vi "Multichannel Lockin.vi"() -> ()   [LabVIEW 2019, in "Instrument.Lockin.lvclass"]
uses:
  Instrument.Lockin/Instrument.Lockin.lvclass
  <vilib>/Utility/error.llb/DialogType.ctl
  <vilib>/measure/NI_MAPro.lvlib
  <vilib>/Waveform/WDTOps.llb/WDT Waveform to XY Pairs DBL.vi
  <vilib>/Utility/config.llb/NI_LVConfig.lvlib
  <vilib>/JKI/JKI SMO/SMO/SMO.lvclass
  Lockin.DAQ/Lockin.DAQ.lvclass
  <userlib>/LevyLab/Levylab Instruments/SMOs/RemoteControl/RemoteControl.lvclass
  <userlib>/LevyLab/Levylab Instruments/SMOs/RemoteControl/Typedefs/Message--Cluster.ctl
  <userlib>/LevyLab/Levylab Instruments/SMOs/RemoteControl/Typedefs/PrivateEvents--RemoteControl.Configure.ctl
  Lockin.DAQ/Typedefs/Results--Cluster.ctl
  <userlib>/LevyLab/Levylab Instruments/SMOs/Instrument/Instrument.lvclass
  Lockin.DAQ/Typedefs/Set State-enum.ctl
  <vilib>/JKI/JKI SMO/SMO/Typedefs/Reserve State--Enum.ctl
  <vilib>/JKI/JKI SMO/SMO/Typedefs/Public Events.ctl
  <vilib>/JKI/JKI SMO/SMO/Typedefs/SMOState --Enum.ctl
  Lockin.DAQ/Typedefs/Sample Mode--Ring.ctl
  Lockin.DAQ/Typedefs/Sweep Configuration--Cluster.ctl
  Lockin.DAQ/Typedefs/SweepResults--Cluster.ctl
  Lockin.DAQ/Typedefs/PrivateEvents--Lockin.DAQ.zeroOffset.ctl
  Lockin.DAQ/Typedefs/PrivateEvents--Lockin.DAQ.measureOffset.ctl
  Instrument.Lockinl.UI/Instrument.Lockin.UI.lvclass
  Lockin.DAQ/Typedefs/PublicEvents--Lockin.DAQ.getSweepWaveforms.ctl
  Lockin.DAQ/Typedefs/PrivateEvents--LockinDAQ.setCalibration.ctl
  Instrument.Lockin/Typedefs/Offset Mode--Enum.ctl
  Lockin.DAQ/Typedefs/Sweep Pattern--Enum.ctl
  Instrument.Lockinl.UI/Typedefs/Sweep Channel--Cluster.ctl
  Lockin.DAQ/Typedefs/Sampling.ctl
  Lockin.DAQ/Typedefs/PrivateEvents--Lockin.DAQ.Reset Phase.ctl
  <vilib>/Platform/browser.llb/Open URL in Default Browser (string).vi
  <vilib>/Waveform/WDTOps.llb/WDT Waveform Duration DBL.vi
  Lockin.DAQ/Typedefs/AO_Channel-Numeric.ctl
  Instrument.Lockin/Typedefs/API/Lockin.setAUX--cluster.ctl
  <userlib>/_OpenG.lib/error/error.llb/Filter Error Codes (Array)__ogtk.vi
  <userlib>/LevyLab/Levylab Instruments/SMOs/Logger.Error/Logger.Error.lvclass
  <vilib>/Utility/sysdir.llb/System Directory Type.ctl
  C:/Program Files (x86)/National Instruments/LabVIEW 2019/vi.lib/JKI/JKI SMO/SMO/SMO.lvclass
  b3b4868b-d429-4095-be3c-1c606df9f133.vi
  f8e81ae1-39f2-419c-8ba3-60eeaa59b30a.vi
  69b91500-227a-4616-af62-c626a830a60f.vi
  C:/Program Files (x86)/National Instruments/LabVIEW 2019/user.lib/LevyLab/Levylab Instruments/SMOs/Instrument/Instrument.lvclass
  C:/Program Files (x86)/National Instruments/LabVIEW 2019/user.lib/LevyLab/Levylab Instruments/SMOs/Logger/Logger.lvclass
  <vilib>/measure/maspectr.llb/FFT Power Spectrum and PSD for N Chan.vi
  Lockin.DAQ/Typedefs/AI.coupling-enum.ctl
  Lockin.DAQ/Typedefs/446xAI-enum.ctl
  Lockin.DAQ/Typedefs/446xAO-enum.ctl
  Lockin.DAQ/Typedefs/Function-enum.ctl
  Lockin.DAQ/Typedefs/Cal Info - Cluster.ctl
  Lockin.DAQ/Typedefs/DAQType-enum.ctl
  Instrument.Lockinl.UI/Typedefs/Display-Enum.ctl
  Lockin.DAQ/Typedefs/AI Simulation-enum.ctl
  Instrument.Lockin/Typedefs/Sample Mode--Enum.ctl
  Instrument.Lockinl.UI/Typedefs/Device Configuration--Cluster.ctl
  Instrument.Lockinl.UI/Typedefs/AO Channel--Cluster.ctl
  Instrument.Lockinl.UI/Typedefs/REF Channel--Cluster.ctl
  Instrument.Lockinl.UI/Typedefs/AI Channel--Cluster.ctl
  Instrument.Lockin/Typedefs/Results Type--Enum.ctl
panel:
  out "Results Plot Names":string[](array[string])
  out "Version":string="vDevelopment" caption="V"
  in  "Tab Control 4":T1(tab)
  in  "Disable all AI Ref":bool
  in  "Enable only AI Ref1":bool
  in  "Reset Phase":bool
  in  "AI Channels":T2[](array[typedef]) {"References" items=["", "1"]}
  in  "AO freq link":dbl=13.0 format="%.3p"
  in  "AO Amp Limit":dbl=0.009999999 format="%.3p"
  in  "Limit Amplitudes":bool
  in  "Link Frequencies":bool
  in  "LP f (Hz)":dbl=100.0 format="%.3p"
  in  "Line":bool
  in  "Lowpass":bool
  in  "AO Channels":T3[](array[typedef]) {"Phase" format="%.3g"; "Frequency" min=0.0001 max=10000.0 format="%.3g"; "Offset" format="%.3p"; "Amplitude" min=0.0 max=10.0 format="%.3p"}
  in  "REF Channels":T5[](array[typedef]) {"Roll-Off" min=1; "TC" min=0.0001 format="%#_3p"; "Phase" format="%.3g"; "Frequency" min=0.0001 max=10000.0 format="%.3g"}
  in  "DAQ Config":T6[](array[typedef]) {"AI.Coupling" items=["AC"=10045, "DC"=10050, "GND"=10066]}
  in  "auto DAQ":bool
  in  "Max Fs Refresh Rate (Hz)":dbl=10.0 format="%#_13g"
  in  "Sampling Mode":T10
  in  "Sampling":T11={"Fs"=10000.0, "#s"=1000}
  in  "DAQ Type":T12=enum."PXI 446x"
  in  "Auto x*F1":dbl=5000.0 format="%#_13g"
  in  "Load Configuration":bool
  in  "Save Configuration":bool
  in  "AI Simulation mode":T13=enum."AI = noise*AO"
  in  "decimating factor":i32=1
  in  "Remove":bool
  in  "Measure":bool
  in  "Stop Sweep":bool caption="Stop"
  in  "Sweep Time (s)":dbl=20.0 format="%#_1f"
  in  "Start Sweep":bool caption="Start"
  in  "Initial Wait (s)":dbl=1.0
  out "Sweep Timer (s)":dbl caption="Timer (s)"
  in  "Return to Start?":bool
  in  "Channels: Sweep":T14[](array[typedef]) {"Channel" items=["AO1"=1, "AO2"=2, "AO3"=3, "AO4"=4, "AO5"=5, "AO6"=6, "AO7"=7, "AO8"=8]; "Start" format="%#_6p"; "End" format="%#_6p"}
  out "Sampling Status":string="Good"
  in  "Output Gain":cluster{"AI.Ch":string, "Gain":dbl}[](array[cluster])=[{"AI.Ch"="AO1", "Gain"=1.0}, {"AI.Ch"="AO2", "Gain"=1.0}, {"AI.Ch"="AO3", "Gain"=1.0}, {"AI.Ch"="AO4", "Gain"=1.0}, {"AI.Ch"="AO5", "Gain"=1.0}, {"AI.Ch"="AO6", "Gain"=1.0}, {"AI.Ch"="AO7", "Gain"=1.0}, {"AI.Ch"="AO8", "Gain"=1.0}, {"AI.Ch"="AO9", "Gain"=1.0}, {"AI.Ch"="AO10", "Gain"=1.0}, {"AI.Ch"="AO11", "Gain"=1.0}, {"AI.Ch"="AO12", "Gain"=1.0}, {"AI.Ch"="AO13", "Gain"=1.0}, {"AI.Ch"="AO14", "Gain"=1.0}, {"AI.Ch"="AO15", "Gain"=1.0}, {"AI.Ch"="AO16", "Gain"=1.0}]
  in  "Input Gain":cluster{"AI.Ch":string, "Gain":dbl}[](array[cluster])=[{"AI.Ch"="AI1", "Gain"=1.0}, {"AI.Ch"="AI2", "Gain"=1.0}, {"AI.Ch"="AI3", "Gain"=1.0}, {"AI.Ch"="AI4", "Gain"=1.0}, {"AI.Ch"="AI5", "Gain"=1.0}, {"AI.Ch"="AI6", "Gain"=1.0}, {"AI.Ch"="AI7", "Gain"=1.0}, {"AI.Ch"="AI8", "Gain"=1.0}, {"AI.Ch"="AI9", "Gain"=1.0}, {"AI.Ch"="AI10", "Gain"=1.0}, {"AI.Ch"="AI11", "Gain"=1.0}, {"AI.Ch"="AI12", "Gain"=1.0}, {"AI.Ch"="AI13", "Gain"=1.0}, {"AI.Ch"="AI14", "Gain"=1.0}, {"AI.Ch"="AI15", "Gain"=1.0}, {"AI.Ch"="AI16", "Gain"=1.0}]
  out "State History":string=" Exit\r Data: Cleanup\r Events: Unregister\r UI: Cleanup\r UI: Disable Buttons\r Configuration: Write\r Error Logger: Destroy\r Lockin SMO: Stop\r Remote SMO: Stop\r Macro: Exit\r UI: Update Sweep Timer\r UI: Update Lockin Graphs\r UI: Update Waveform Graphs\r 4461: OUT\r UI: Update Sweep Timer\r UI: Update Lockin Graphs\r UI: Update Waveform Graphs\r 4461: OUT\r UI: Update Sweep Timer\r UI: Update Lockin Graphs\r UI: Update Waveform Graphs\r 4461: OUT"
  out "Refresh time (ms)":u32=103
  out "LockinDAQ SMO State":T16=enum."Stopped" caption="SMO State"
  out "RC SMO State":T16=enum."Stopped" caption="SMO State"
  in  "Update":bool
  in  "Enable Output":bool caption="Enable"
  in  "Output Channel":i32=1 min=1
  out "Output (V)":dbl
  in  "Aux Channel":tag="Dev2/ao0"
  in  "Voltage Output (V)":dbl min=-50.0 max=50.0
  in  "Amplifier Gain":dbl=1.0 min=-15.0 max=15.0
  out "DAQ Output (V)":dbl=-0.0 min=-3.5 max=3.5
  out "Amplified Output (V)":dbl=-0.0 min=-3.5 max=3.5
  in  "AI Channel":i32=1
  in  "Reference Channel":i32=1
  in  "Type":T17
  in  "Allowed remote system":string
  in  "Get Calibration":bool
  out "Cal Info":T18[](array[typedef]) {"SelfCal.LastDate/Time" format="%<%I:%M %p\n%m/%d/%Y>T"}
  in  "Self Calibrate":bool
  in  "Save":bool
  in  "Path":path=path "C:/Data/lockin"
  in  "Notes":string
  in  "Tab Control 3":enum32{"Page 1"}(tab)
  out "X":dbl=0.0014996100939563214 caption="X (V)" format="%#_3p"
  out "Y":dbl=-29.79492153733761 caption="Y (V)" format="%#_3p"
  in  "Channel":i32(ring)=1 items=["AI1 Ref1", "AI2 Ref1", "AI3 Ref1", "AI4 Ref1", "AI5 Ref1", "AI6 Ref1", "AI7 Ref1", "AI8 Ref1"]
  out "R":dbl=0.0014996100939563214 caption="R (V)" format="%#_3p"
  out "Theta":dbl=-29.79492153733761 caption="Theta (°)" format="%#_3p"
  in  "Display":T19=enum."R and Theta" caption="Enum"
  in  "Close":bool
  out "Status":string="Shutdown"
  in  "Pause":bool
  in  "Reset":bool
  in  "Start":bool
  in  "Help":bool
  in  "Trigger":bool
  in  "Tab Control 2":T20(tab)
  in  "AI Graph All":bool
  in  "AI Graph None":bool
  in  "Y Axis (Output)":enum16{"Analog Output", "Reference"}(ring) caption="Enum 3"
  in  "Y Axis (Input)":enum16{"Device", "ADC"}(ring) caption="Enum 3"
  in  "Decimate":enum16{"1", "10", "100", "1000"}(ring) caption="Enum 3"
  in  "X Axis":enum16{"Time", "Samples"}(ring) caption="Enum 3"
  out "AI Graph":waveform(dbl)[](graph)
  out "AO Graph":waveform(dbl)[](graph)
  in  "AO Graph All":bool
  in  "AO Graph None":bool
  in  "Y/Theta Range":dbl caption="Axis Range" format="%#_6p"
  in  "X/R Range":dbl caption="Axis Range" format="%#_6p"
  out "Lockin 2":waveform(dbl)[](graph) caption="Lockin Display 2"
  out "Lockin 1":waveform(dbl)[](graph)
  in  "Lockin 1 None":bool
  in  "Lockin 1 All":bool
  out "Results":string[][](table)
  out "XY Graph":cluster{"Wavenumber":dbl[], "Data":dbl[]}[](graph)
  in  "Numeric":dbl caption="Axis Range" format="%#_6p"
  out "Sweep Results Y":waveform(dbl)[](graph)
  out "Sweep Results X":waveform(dbl)[](graph)
  out "Sweep Results AI":waveform(dbl)[](graph)
  out "Sweep Results AO":waveform(dbl)[](graph)
  in  "# averages":u32=10 min=1
  in  "weighting mode":enum16{"Linear", "Exponential"}(ring)=enum."Exponential"
  in  "averaging mode":T21(ring)=enum."RMS averaging"
  in  "window":u16(ring) items=["Rectangle", "Hanning"]
  in  "export mode":u16(ring)=1 items=["Power Spectrum", "Power Spectral Density"]
  in  "restart":bool
  out "done?":bool=TRUE
  out "PS Chart":dbl[][](graph)
  out "PS WFGraph":cluster{"f0":dbl, "df":dbl, "magnitude":dbl[]}[](graph)
  out "averages":dbl=180.0
  # "Output"
  # "Input"
  # ">> DEVICE >>"
  # "Amp (V)"
  # "(*)"
  # "Ch"
  # "DC (V)"
  # "f (Hz)"
  # "Phase (°)"
  # "Function"
  # "Sweep"
  # "(*)"
  # "Ch"
  # "Ref1   2     3    4"
  # "Input: Pre-Filter"
  # "Output Settings"
  # "Reference"
  # "Reference Settings"
  # "Ch"
  # "f (Hz)"
  # "Phase (°)"
  # "TC (s)"
  # "Order"
  # "DAQ Channels"
  # "AI"
  # "Device"
  # "AO"
  # "Input: Offset"
  # "Ch"
  # "Range"
  # "Ch"
  # "Range"
  # "Coupling"
  # "Other Configuration"
  # "Sampling"
  # "Changing settings in this box will automatically\nreset the lockin and restart acquisition"
  # "Sweep"
  # "Channel"
  # "Start"
  # "End"
  # "Pattern"
  # "Status"
  # "Channel"
  # "Channel"
  # "Input Gain"
  # "Output Gain"
  # "Auxiliary Output"
  # "Configuration"
  # "- Use to control an auxiliiary card such as a multifunction DAQ (6115, 6120, etc)"
  # "Forward Lockin Input --> Lockin Output"
  # "- Choose an input lockin channel and value (X,Y, etc) and it will be written as a DC value to an output channel of your choosing.\n- Output is scaled by the input amplifier gain."
  # "Calibration"
  # "Self Cal\nLast Time"
  # "Self Cal\nLast Temp"
  # "Temp\nNow"
  # "Cal\nDue"
  # "Device"
  # "AI Graph"
  # "AO/Reference Graph"
  # "Lockin Results 1"
  # "Lockin Results 2"
  # "Lockin Results 2"
  # "Sweep Results"
  # "Sweep AO/AI"
  # "Power Spectra"
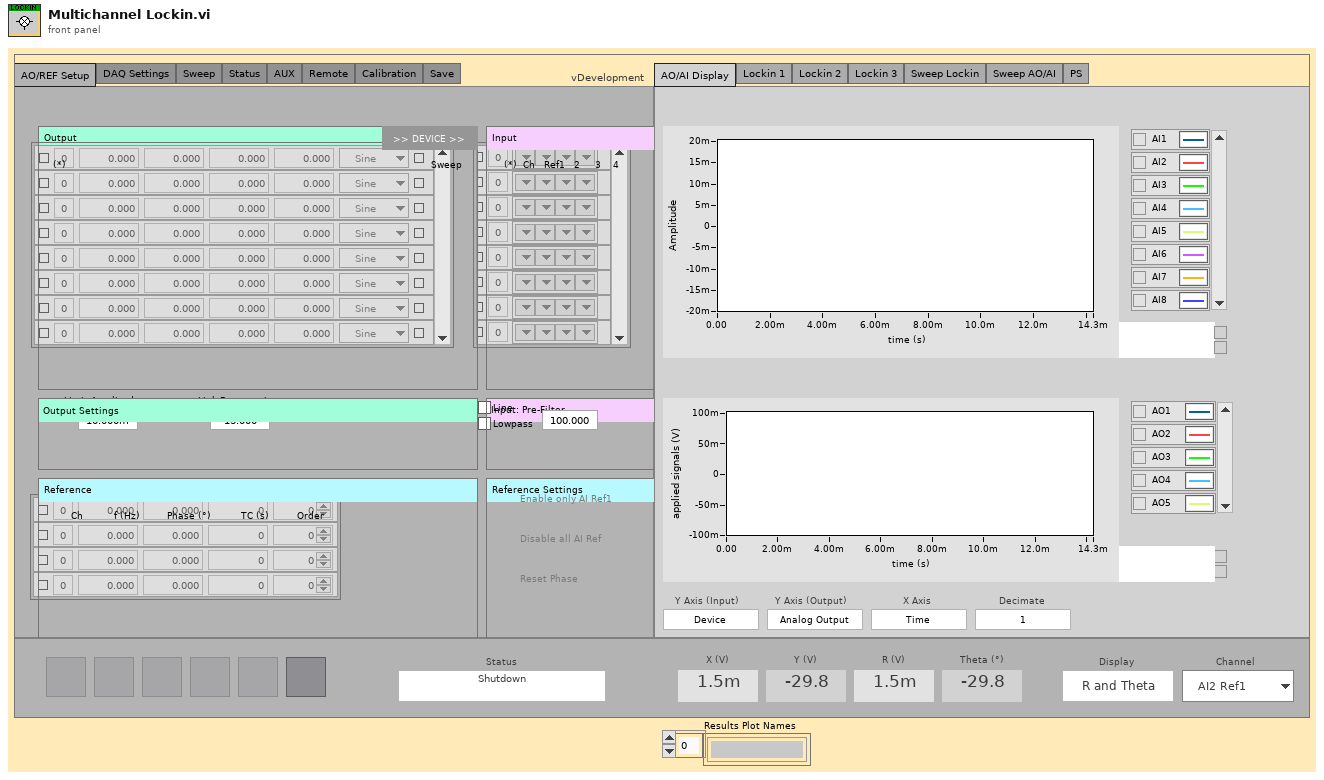
[diagram p1: front panel]
types:
  T1 = enum32{"AO/REF Setup", "DAQ Settings", "Sweep", "Status", "AUX", "Remote", "Calibration", "Save"}
  T2 = typedef "Instrument.Lockin.UI.lvclass/AI Channel--Cluster.ctl" = cluster{"Enable?":bool, "Channel":i32, "References":u16[]}
  T3 = typedef "Instrument.Lockin.UI.lvclass/AO Channel--Cluster.ctl" = cluster{"Enable?":bool, "Channel":i32, "Amplitude":dbl, "Offset":dbl, "Frequency":dbl, "Phase":dbl, "Function":T4, "Sweeping?":bool}
  T4 = typedef "Lockin.DAQ.lvclass/Function-enum.ctl" = enum16{"Sine", "Triangle", "Square"}
  T5 = typedef "Instrument.Lockin.UI.lvclass/REF Channel--Cluster.ctl" = cluster{"Enable?":bool, "Channel":i32, "Frequency":dbl, "Phase":dbl, "TC":dbl, "Roll-Off":i32}
  T6 = typedef "Instrument.Lockin.UI.lvclass/Device Configuration--Cluster.ctl" = cluster{"Device":string, "AO.Ch":string, "AO.Range":T7, "AI.Ch":string, "AI.Range":T8, "AI.Coupling":T9}
  T7 = typedef "Lockin.DAQ.lvclass/446xAO-enum.ctl" = enum16{"±0.1", "±1.0", "±10.0"}
  T8 = typedef "Lockin.DAQ.lvclass/446xAI-enum.ctl" = enum16{"±0.316", "±1.00", "±3.16", "±10.0", "±31.6", "±42.4"}
  T9 = typedef "Lockin.DAQ.lvclass/AI.coupling-enum.ctl" = u16
  T10 = typedef "Instrument.Lockin.lvclass/Sample Mode--Enum.ctl" = enum16{"Manual", "Auto Fs", "Max Fs"}
  T11 = typedef "Lockin.DAQ.lvclass/Sampling.ctl" = cluster{"Fs":dbl, "#s":i32}
  T12 = typedef "Lockin.DAQ.lvclass/DAQType-enum.ctl" = enum16{"None", "USB 4431", "PXI 446x"}
  T13 = typedef "Lockin.DAQ.lvclass/AI Simulation-enum.ctl" = enum16{"AI = HW simulated", "AI = noise*AO", "AI = waveguide"}
  T14 = typedef "Instrument.Lockin.UI.lvclass/Sweep Channel--Cluster.ctl" = cluster{"End":dbl, "Start":dbl, "Channel":u16, "Pattern":T15}
  T15 = typedef "Lockin.DAQ.lvclass/Sweep Pattern--Enum.ctl" = enum16{"Ramp /", "Ramp /\\", "Smooth Ramp _/", "Smooth Ramp _/\\_", "Frequency"}
  T16 = typedef "SMO.lvclass/SMOState --Enum.ctl" = enum16{"unknown", "Created", "Started", "Stopped"}
  T17 = typedef "Instrument.Lockin.lvclass/Results Type--Enum.ctl" = enum16{"X", "Y", "R", "Theta", "Mean"}
  T18 = typedef "Lockin.DAQ.lvclass/Cal Info - Cluster.ctl" = cluster{"Active Device":string, "SelfCal.LastDate/Time":dbl, "SelfCal.LastTemp":dbl, "DevTemp":dbl, "calibration due?":bool}
  T19 = typedef "Instrument.Lockin.UI.lvclass/Display-Enum.ctl" = enum16{"X and Y", "R and Theta", "Mean"}
  T20 = enum32{"AO/AI Display", "Lockin 1", "Lockin 2", "Lockin 3", "Sweep Lockin", "Sweep AO/AI", "PS"}
  T21 = enum16{"No averaging", "Vector averaging", "RMS averaging", "Peak hold"}
  T22 = typedef "Lockin.DAQ.lvclass/Set State-enum.ctl" = enum16{"start", "stop", "reset", "start sweep", "stop sweep"}
  T23 = typedef "Lockin.DAQ.lvclass/Sweep Configuration--Cluster.ctl" = cluster{"Sweep Time (s)":dbl, "Initial Wait (s)":dbl, "Return to Start":bool, "Channels":T14[]}
  T24 = enum32{"invalid app kind", "Development System", "Run Time System", "Student Edition", "Embedded LabVIEW", "Evaluation", "Custom"}
  T25 = enum8{"Enabled", "Disabled", "Disabled and Grayed Out"}
  T26 = enum32{"Invalid", "Standard", "Closed", "Hidden", "Minimized", "Maximized"}
  T27 = typedef "Lockin.DAQ.lvclass/PrivateEvents--LockinDAQ.setCalibration.ctl" = bool
  T28 = typedef "Lockin.DAQ.lvclass/PrivateEvents--Lockin.DAQ.Reset Phase.ctl" = bool
  T29 = typedef "Lockin.DAQ.lvclass/PrivateEvents--Lockin.DAQ.measureOffset.ctl" = bool
  T30 = typedef "Lockin.DAQ.lvclass/PrivateEvents--Lockin.DAQ.zeroOffset.ctl" = bool
  T31 = cluster{"averaging mode":enum16{"No averaging", "Vector averaging", "RMS averaging", "Peak hold"}, "weighting mode":enum16{"Linear", "Exponential"}, "number of averages":u32}
  T32 = typedef "Instrument.Lockin.lvclass/Lockin.setAUX--cluster.ctl" = cluster{"AO Channel":T33, "AUX (V)":dbl}
  T33 = typedef "Lockin.DAQ.lvclass/AO_Channel-Numeric.ctl" = i32
  T34 = typedef "Instrument.Lockin.lvclass/Offset Mode--Enum.ctl" = enum16{"Measure", "Remove"}
  T35 = typedef "Lockin.DAQ.lvclass/State-enum.ctl" = enum16{"idle", "created", "started", "stopped", "sweeping"}
  T36 = typedef "Lockin.DAQ.lvclass/PublicEvents--Lockin.DAQ.getAO.ctl" = waveform(dbl)[]
  T37 = typedef "RemoteControl.lvclass/PrivateEvents--RemoteControl.Configure.ctl" = cluster{"address":string, "Port":u16, "AllowedRemote":string, "Commands":string[], "timeout":i32}
  T38 = typedef "RemoteControl.lvclass/Message--Cluster.ctl" = cluster{"Command":string, "Data":variant, "ID":string}
  T39 = typedef "Lockin.DAQ.lvclass/SweepResults--Cluster.ctl" = cluster{"X results":waveform(dbl)[], "Y Results":waveform(dbl)[]}
  T40 = typedef "Lockin.DAQ.lvclass/PublicEvents--Lockin.DAQ.getSweepWaveforms.ctl" = cluster{"Sweep_AO":waveform(dbl)[], "Sweep_AI":waveform(dbl)[]}
  T41 = cluster{"Core":cluster{"Current VI Reference":refnum<vi>, "Close Panel on Exit?":bool}, "to":i32, "Lockin":refnum<class "Instrument.Lockin.lvclass">, "RemoteControl":refnum<class "RemoteControl.lvclass">, "Lockin.DAQ":refnum<class "Lockin.DAQ.lvclass">, "Logger.Error":refnum<class "Logger.Error.lvclass">, "RemoteControl.Configure":T37, "Message":T38, "HandledMessage":T38, "SweepResults":T39, "SweepWaveforms":T40}
  T42 = typedef "Lockin.DAQ.lvclass/PublicEvents--Lockin.DAQ.getAI.ctl" = waveform(dbl)[]
  T43 = cluster{"X":waveform(dbl)[], "Y":waveform(dbl)[]}
  T44 = typedef "Lockin.DAQ.lvclass/Results--Cluster.ctl" = cluster{"Time Stamp":timestamp, "Results (Dictionary)":cluster{"key":string, "value":dbl}[]}
  T45 = typedef "Lockin.DAQ.lvclass/AO-cluster.ctl" = T3[]
  T46 = typedef "Lockin.DAQ.lvclass/REF-cluster.ctl" = T5[]
  T47 = typedef "Lockin.DAQ.lvclass/PublicEvents--Lockin.DAQ.getCalibration.ctl" = T18[]
  T48 = typedef "Lockin.DAQ.lvclass/PublicEvents--Lockin.DAQ.getDAQconfig.ctl" = T6[]
  T49 = typedef "Lockin.DAQ.lvclass/AO.config-array.ctl" = T50[]
  T50 = typedef "Lockin.DAQ.lvclass/AO.config-cluster.ctl" = cluster{"AO.channels":tag, "AO.Range":T7, "output terminal configuration":i32, "DAQ Type":T12}
  T51 = typedef "Lockin.DAQ.lvclass/AI.config-array.ctl" = T52[]
  T52 = typedef "Lockin.DAQ.lvclass/AI.config-cluster.ctl" = cluster{"AI.channels":tag, "AI.Coupling":T9, "AI.Range":T8, "input terminal configuration":i32, "DAQ Type":T12}
  T53 = typedef "Lockin.DAQ.lvclass/Sample Mode--Ring.ctl" = i32
  T54 = typedef "DialogType.ctl" = u16
  T55 = cluster{"Current VI Reference":refnum<vi>, "Close Panel on Exit?":bool}
  T56 = typedef "SMO.lvclass/Public Events.ctl" = cluster{"Error":refnum<user-event>, "State":refnum<user-event>, "Reserve State":refnum<user-event>}
  T57 = typedef "RemoteControl.lvclass/PublicEvents--Cluster.ctl" = cluster{"SendMessageFromProcess":refnum<user-event>}
  T58 = typedef "Lockin.DAQ.lvclass/PublicEvents--Cluster.ctl" = cluster{"getAO":refnum<user-event>, "getAI":refnum<user-event>, "getREF":refnum<user-event>, "getResults":refnum<user-event>, "getCalibration":refnum<user-event>, "getAOChannels":refnum<user-event>, "getREFChannels":refnum<user-event>, "getDAQState":refnum<user-event>, "getSweepResults":refnum<user-event>, "getSweepWaveforms":refnum<user-event>, "getDAQconfig":refnum<user-event>}
  T59 = typedef "Lockin.DAQ.lvclass/AI-cluster.ctl" = T2[]
  T60 = typedef "System Directory Type.ctl" = i32
  T61 = typedef "RemoteControl.lvclass/RC Com Type--enum.ctl" = enum16{"RC", "STM", "ZMQ"}
  T62 = typedef "Lockin.DAQ.lvclass/AI Prefilter-cluster.ctl" = cluster{"60 Hz prefilter":bool, "LP prefilter":bool, "LP cutoff (Hz)":dbl}
  T63 = typedef "Instrument.Lockin.lvclass/Lockin.Configuration--Cluster.ctl" = cluster{"AO Channels":T45, "REF Channels":T46, "AI Channels":T59, "REF Filter":T62, "Amplifers":cluster{"offsets":dbl[], "Input Gain":dbl[], "Output Gain":dbl[], "Amplifiers":T64}, "DAQ":cluster{"sampling":T11, "sample mode":i32, "buffer size (S)":u32, "decimation":u32}, "Calibration":cluster{"Cal Info":T18[]}, "AI Configuration":T51, "AO Configuration":T49, "Aux Channel":tag, "Simulation mode":T13}
  T64 = typedef "Lockin.DAQ.lvclass/AmplifierType-enum.ctl" = enum16{"Manual", "Krohn Hite", "Femto"}
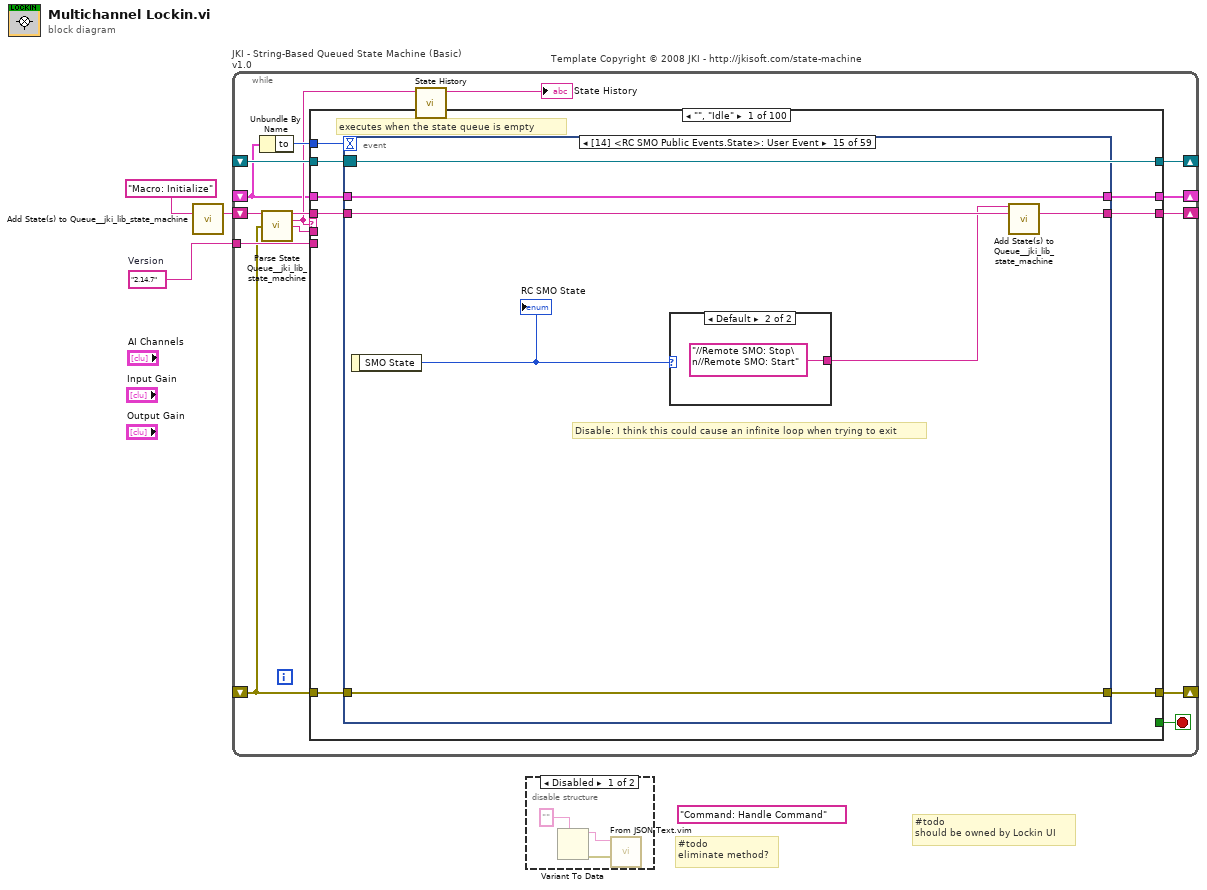
[diagram p0: block diagram]
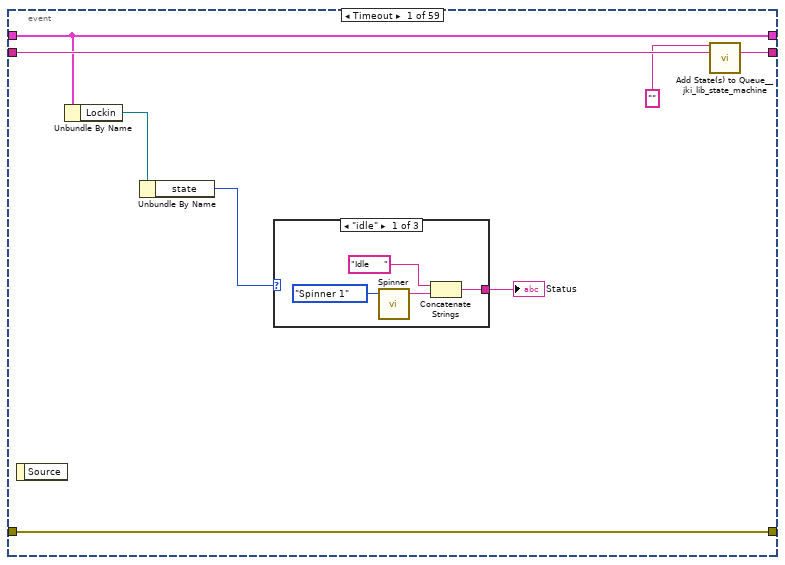
[diagram p3: hidden frame]
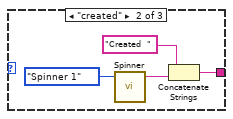
[diagram p4: hidden frame]
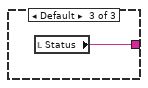
[diagram p5: hidden frame]
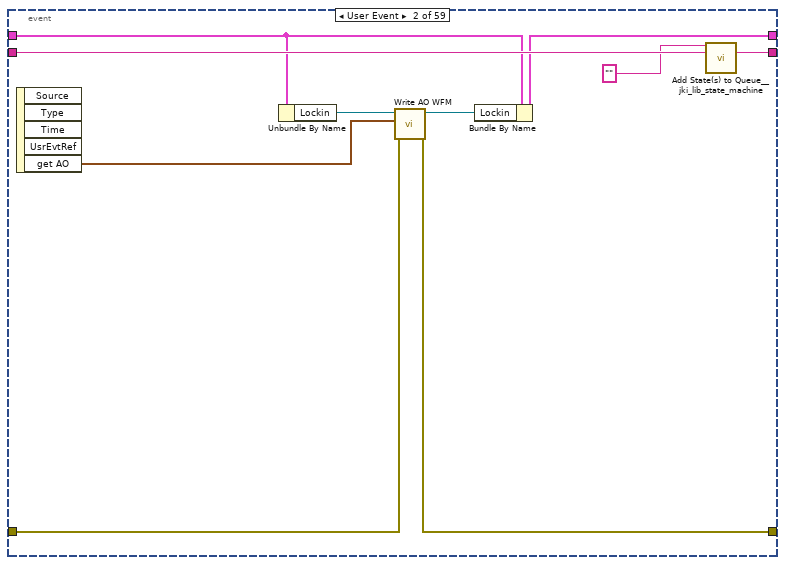
[diagram p6: hidden frame]
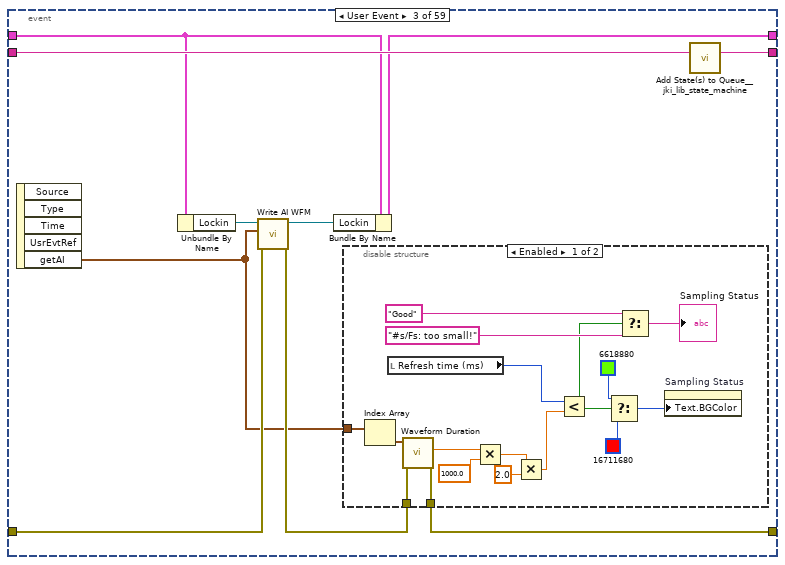
[diagram p7: hidden frame]
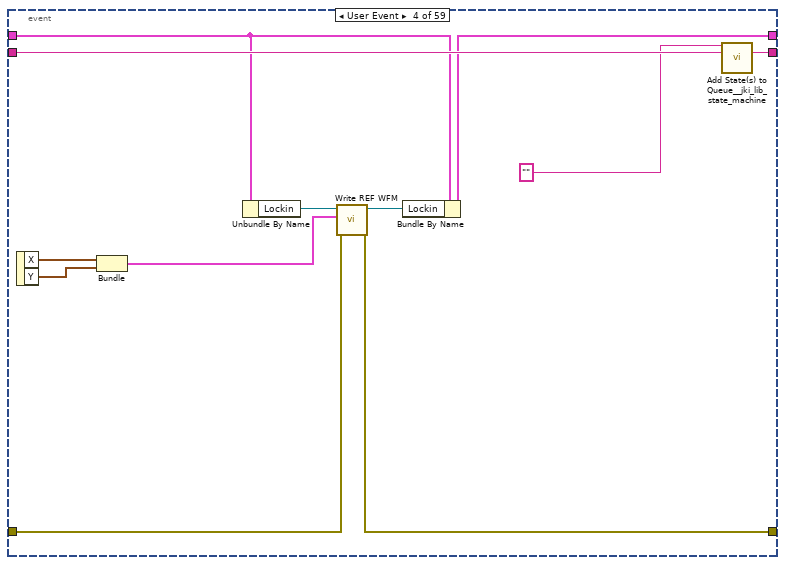
[diagram p9: hidden frame]
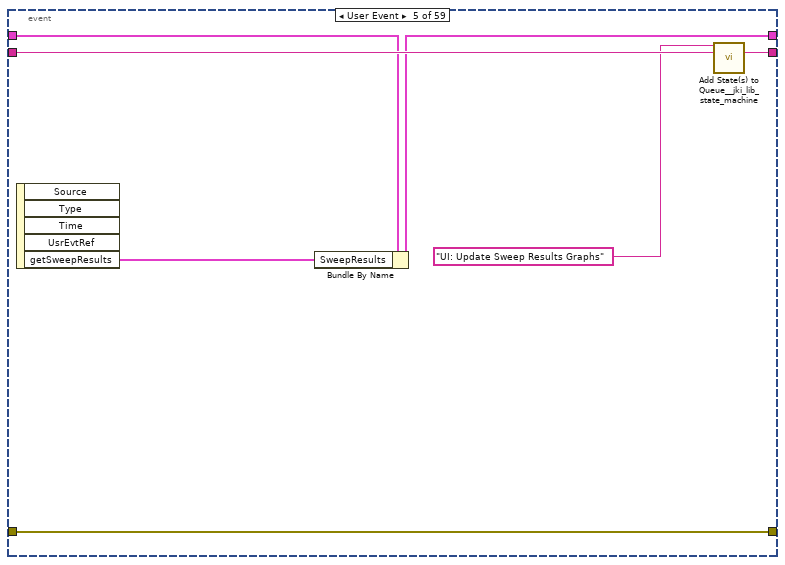
[diagram p10: hidden frame]
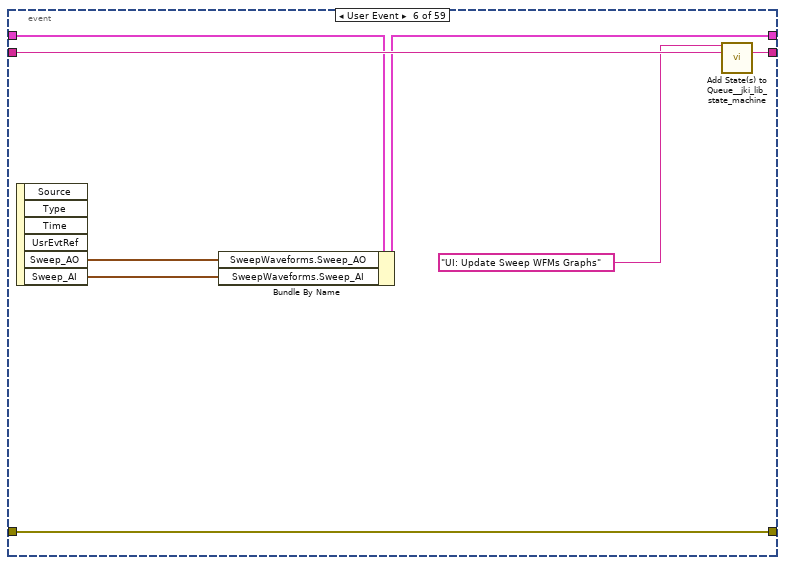
[diagram p11: hidden frame]
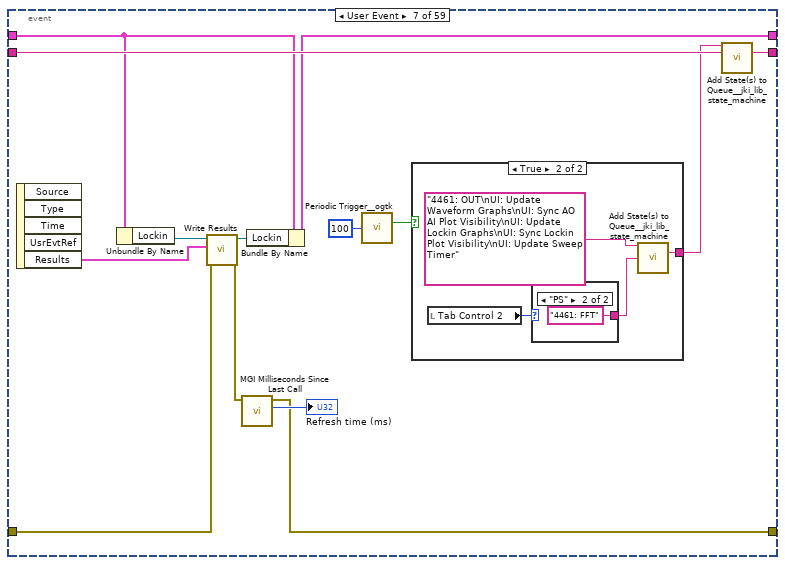
[diagram p12: hidden frame]
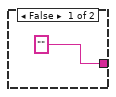
[diagram p13: hidden frame]
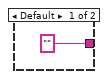
[diagram p14: hidden frame]
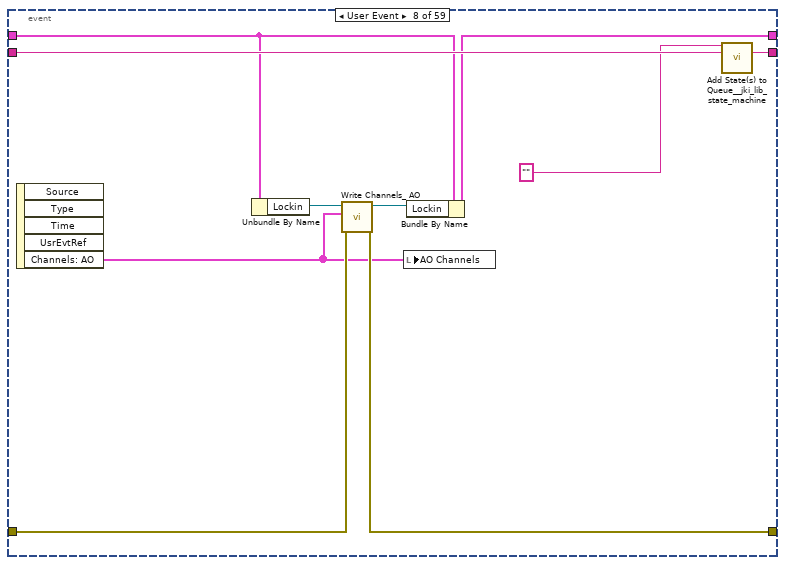
[diagram p15: hidden frame]
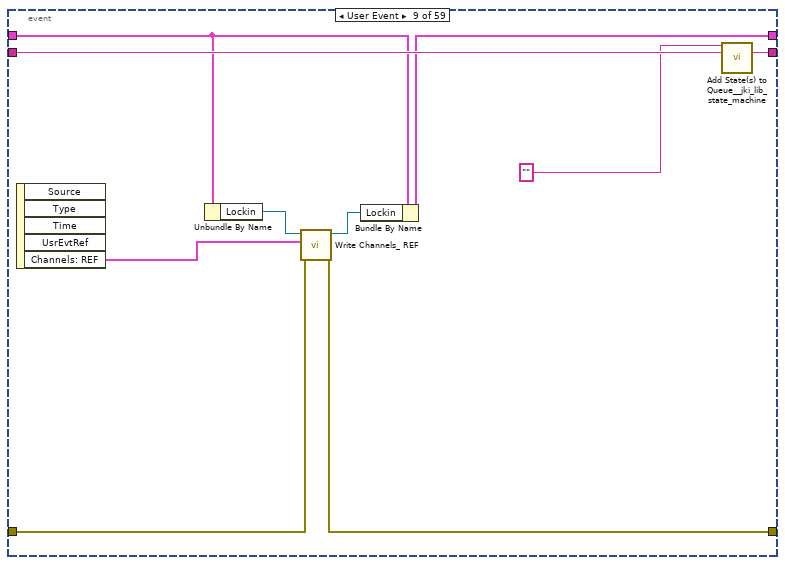
[diagram p16: hidden frame]
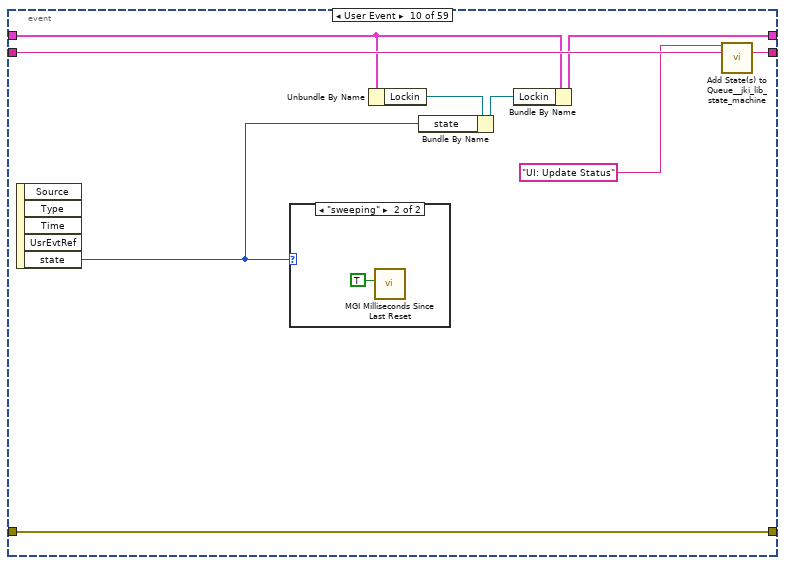
[diagram p17: hidden frame]
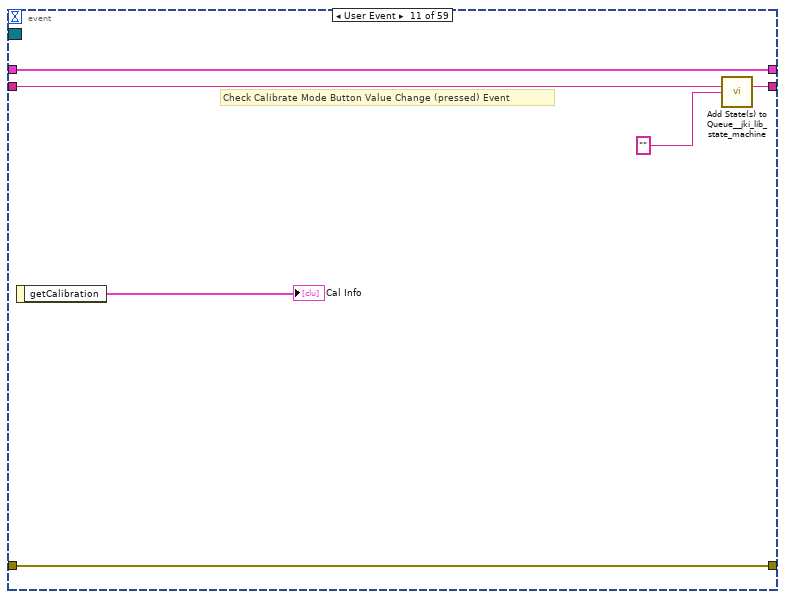
[diagram p19: hidden frame]
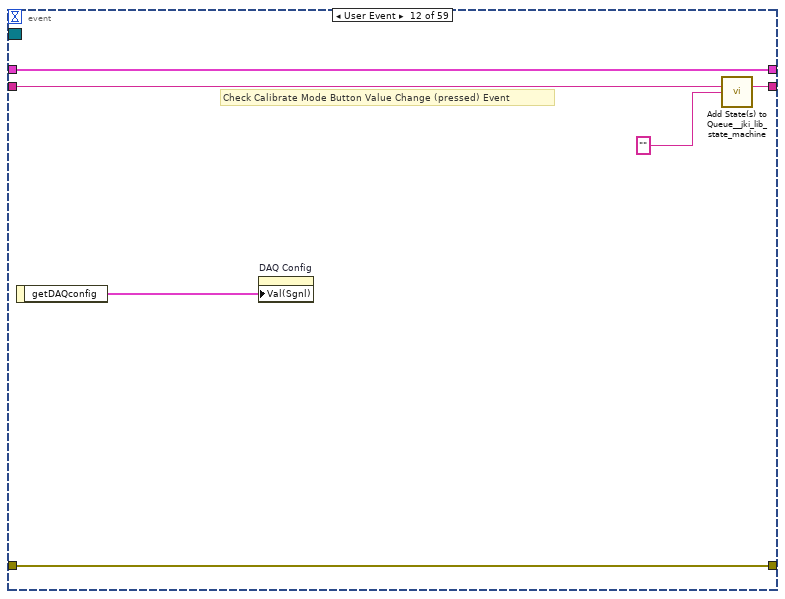
[diagram p20: hidden frame]
diagram:
  (unwired) "Command: Handle Command" ("State(s) in Front (\"\")")
  w1 = "2.14.7"  # Version
  # "#todo\nshould be owned by Lockin UI"
  # "#todo\neliminate method?"
  # "Template Copyright © 2008 JKI - http://jkisoft.com/state-machine"
  n1 = call <vilib>:"Add State(s) to Queue__jki_lib_state_machine.vi"("State(s) in (\"\")"="Macro: Initialize") -> ("States Out"=w3:string)  [unwired: 14 in]
  n2 = while "JKI - String-Based Queued State Machine (Basic) v1.0" {
    shift-right: [w10] -> _
    shift-left: _ -> [w4]
    shift-right: [w7] -> _
    shift-left: _ -> [w5]
    shift-right: [w17] -> _
    shift-left: w3 -> [w14]
    shift-right: [w11] -> _
    shift-left: _ -> [w12]
    tunnel: w1 -> [w6]
    stop <- w16 stop-if-true
    n3 = Unbundle By Name(w4) -> ("to"=w13:i32)
    n4 = call <vilib>:"Parse State Queue__jki_lib_state_machine.vi"("State Queue"=w14, "Error In (no error)"=w5) -> ("Remaining States"=w15:string, "Current State"=w8:string, "Arguments"=w18:string)  [unwired: 11 in]
    n5 = case shown="\"\", \"Idle\"" w8 {
      selector: w8 -> [_ _ w646 _ _ _ _ _ _ _ _ _ _ _ _ _ _ _ _ _ _ _ _ _ _ _ _ _ _ _ _ _ _ _ _ _ _ _ _ _ _ _ _ _ _ _ _ _ _ _ _ _ _ _ _ _ _ _ _ _ _ _ _ _ _ _ _ _ _ _ _ _ _ _ _ _ _ _ _ _ _ _ _ _ _ _ _ _ _ _ _ _ _ _ _ _ _ _ _ _]
      tunnel: w18 -> [_ _ _ _ _ _ _ _ _ _ _ _ _ _ _ _ _ _ w833 _ _ w897 _ _ _ _ w1055 w1069 w1088 _ _ _ _ _ _ _ _ _ w1244 w1257 w1267 _ _ _ _ _ _ _ _ _ _ _ _ _ _ _ _ _ _ _ _ _ _ w1643 _ _ w1684 _ _ _ _ _ _ _ w1769 _ _ _ _ _ _ _ _ _ _ _ _ _ _ _ _ _ _ _ _ _ _ _ _ _]
      tunnel: [w25 w642 w649 w667 w680 w692 w697 w713 w734 w741 w746 w771 w777 w782 w798 w809 w820 w831 w844 w864 w882 w905 w947 w1004 w1033 w1046 w1059 w1072 w1091 w1120 w1150 w1163 w1174 w1182 w1197 w1204 w1212 w1232 w1249 w1258 w1270 w1302 w1307 w1314 w1321 w1329 w1355 w1380 w1399 w1421 w1426 w1455 w1464 w1478 w1491 w1529 w1547 w1556 w1565 w1579 w1592 w1611 w1629 w1649 w1669 w1678 w1691 w1702 w1719 w1731 w1740 w1749 w1758 w1767 w1776 w1785 w1793 w1801 w1809 w1814 w1829 w1857 w1897 w1918 w1943 w1948 w1963 w1968 w1980 w1989 w2006 w2025 w2039 w2044 w2054 w2071 w2087 w2094 w2099 w2104] -> w17
      tunnel: [_ _ _ _ _ TRUE _ _ _ _ _ _ _ _ _ _ _ _ _ _ _ _ _ _ _ _ _ _ _ _ _ _ _ _ _ _ _ _ _ _ _ _ _ _ _ _ _ _ _ _ _ _ _ _ _ _ _ _ _ _ _ _ _ _ _ _ _ _ _ _ _ _ _ _ _ _ _ _ _ _ _ _ _ _ _ _ _ _ _ _ _ _ _ _ _ _ _ _ _ _] -> w16
      tunnel: w13 -> [w20 _ _ _ _ _ _ _ _ _ _ _ _ _ _ _ _ _ _ _ _ _ _ _ _ _ _ _ _ _ _ _ _ _ _ _ _ _ _ _ _ _ _ _ _ _ _ _ _ _ _ _ _ _ _ _ _ _ _ _ _ _ _ _ _ _ _ _ _ _ _ _ _ _ _ _ _ _ _ _ _ _ _ _ _ _ _ _ _ _ _ _ _ _ _ _ _ _ _ _]
      tunnel: w15 -> [w26 w643 w650 w668 w681 w693 w698 w714 w735 w742 w747 w772 w778 w783 w799 w810 w821 w832 w845 w865 w883 w906 w948 w1005 w1034 w1047 w1060 w1073 w1092 w1121 w1151 w1164 w1175 w1183 w1198 w1205 w1213 w1233 w1250 w1259 w1271 w1303 w1308 w1309 w1322 w1330 w1356 w1375 w1400 w1422 w1427 w1456 w1465 w1479 w1492 w1530 w1548 w1557 w1566 w1580 w1593 w1612 w1630 w1650 w1670 w1679 w1692 w1703 w1720 w1732 w1741 w1750 w1759 w1768 w1777 w1786 w1794 w1802 w1810 w1815 w1830 w1856 w1893 w1905 w1944 w1949 w1964 w1969 w1981 w1988 w2005 w2026 w2040 w2045 w2055 w2072 w2088 w2095 w2100 w2105]
      tunnel: w12 -> [w19 w640 w645 w656 w676 w689 w695 w711 w733 w740 w744 _ w774 w779 w796 w808 w819 w830 w843 w863 w881 w904 w945 w1003 w1030 w1043 w1057 w1070 w1089 w1119 w1149 w1161 w1171 w1179 w1195 w1202 w1210 w1229 w1247 w1255 w1264 w1300 w1304 w1312 w1318 w1328 w1354 w1378 w1397 w1414 w1423 w1454 w1463 w1475 w1485 w1524 w1546 w1555 w1561 w1576 w1587 w1607 w1620 w1648 w1668 w1677 w1690 w1701 w1718 w1730 w1739 w1748 w1757 w1766 w1775 w1784 w1792 w1800 w1808 w1811 w1828 w1855 w1894 w1910 w1940 w1945 w1962 w1965 w1979 w1987 w2004 w2022 w2038 w2041 w2053 w2070 w2086 w2091 w2096 w2101]
      tunnel: [w19 w640 w645 w656 w676 w689 w695 w711 w733 w740 w744 w770 w774 w779 w796 w808 w819 w830 w843 w863 w881 w904 w945 w1003 w1030 w1043 w1057 w1070 w1089 w1119 w1149 w1161 w1171 w1179 w1195 w1202 w1210 w1229 w1247 w1255 w1264 w1300 w1304 w1312 w1318 w1328 w1354 w1378 w1397 w1414 w1423 w1454 w1463 w1475 w1485 w1524 w1546 w1555 w1561 w1576 w1587 w1607 w1620 w1648 w1668 w1677 w1690 w1701 w1718 w1730 w1739 w1748 w1757 w1766 w1775 w1784 w1792 w1800 w1808 w1811 w1828 w1855 w1894 w1910 w1940 w1945 w1962 w1965 w1979 w1987 w2004 w2022 w2038 w2041 w2053 w2070 w2086 w2091 w2096 w2101] -> w11
      tunnel: [w22 w639 w648 w666 w673 w688 w694 w708 w720 w737 w743 w769 w776 w780 w797 w807 w818 w829 w842 w862 w880 w890 w946 w999 w1031 w1044 w1058 w1071 w1090 w1111 w1148 w1162 w1172 w1180 w1194 w1201 w1208 w1230 w1248 w1256 w1266 w1301 w1305 w1310 w1319 w1324 w1350 w1376 w1385 w1415 w1424 w1428 w1462 w1476 w1481 w1519 w1545 w1553 w1560 w1577 w1582 w1601 w1619 w1641 w1662 w1672 w1682 w1695 w1710 w1726 w1737 w1742 w1755 w1762 w1774 w1783 w1791 w1795 w1804 w1812 w1816 w1851 w1891 w1904 w1941 w1946 w1957 w1966 w1975 w1982 w1994 w2023 w2028 w2042 w2046 w2068 w2083 w2092 w2097 w2102] -> w10
      tunnel: [w24 w641 w652 w665 w674 w691 w696 w705 w716 w736 w745 w750 w773 w781 w795 w800 w811 w823 w840 w851 w867 w902 w936 w1000 w1032 w1045 w1050 w1063 w1076 w1097 w1136 w1153 w1173 w1181 w1196 w1203 w1211 w1231 w1245 w1253 w1265 w1298 w1306 w1313 w1320 w1323 w1349 w1379 w1398 w1420 w1425 w1435 w1457 w1477 w1490 w1522 w1543 w1551 w1559 w1578 w1584 w1605 w1628 w1645 w1665 w1674 w1687 w1698 w1711 w1728 w1734 w1746 w1751 w1760 w1771 w1780 w1788 w1796 w1803 w1813 w1824 w1852 w1874 w1909 w1942 w1947 w1950 w1967 w1972 w1986 w2003 w2024 w2030 w2043 w2052 w2057 w2074 w2093 w2098 w2103] -> w7
      tunnel: w6 -> [_ _ _ _ _ _ _ _ _ _ _ _ _ _ w786 _ _ _ _ _ _ _ _ _ _ _ _ _ _ _ _ _ _ _ _ _ _ _ _ _ _ _ _ _ _ _ _ _ _ _ _ _ _ _ _ _ _ _ _ _ _ _ _ _ _ _ _ _ _ _ _ _ _ _ _ _ _ _ _ _ _ _ _ _ _ _ _ _ _ _ _ _ _ _ _ _ _ _ _ _]
      tunnel: w5 -> [w23 w641 w651 w665 w670 w691 w696 w705 w723 w738 w745 w749 w773 w781 w793 w803 w814 w825 w835 w859 w877 w887 w937 w995 w1032 w1045 w1054 w1068 w1086 w1101 w1143 w1156 w1173 w1181 w1196 w1203 w1211 w1231 w1246 w1254 w1269 w1298 w1306 w1313 w1320 w1326 w1352 w1379 w1398 w1420 w1425 w1431 w1458 w1477 w1489 w1528 w1544 w1552 w1562 w1578 w1581 w1604 w1622 w1646 w1666 w1675 w1688 w1699 w1716 w1725 w1735 w1743 w1753 w1761 w1772 w1781 w1789 w1797 w1805 w1813 w1825 w1850 w1879 w1909 w1942 w1947 w1951 w1967 w1971 w1983 w2002 w2024 w2031 w2043 w2052 w2056 w2076 w2093 w2098 w2103]
      tunnel: w4 -> [w21 w639 w648 w659 w673 w688 w694 _ w721 w737 w743 w769 w776 w780 w797 w806 w817 w828 w841 w861 w879 w890 w946 w999 w1031 w1044 w1058 w1071 w1090 w1111 w1148 w1162 w1172 w1180 w1194 w1201 w1208 w1230 w1248 w1256 w1266 w1301 w1305 w1310 w1319 w1324 w1350 w1376 w1385 w1415 w1424 w1437 w1462 w1476 w1482 w1520 w1545 w1553 w1560 w1577 w1583 w1600 w1619 w1641 w1662 w1672 w1682 w1695 w1710 w1726 w1737 w1742 w1755 w1762 w1774 w1783 w1791 w1795 w1804 w1812 w1817 w1851 w1891 w1904 w1941 w1946 w1953 w1966 w1970 w1982 w1996 w2023 w2029 w2042 w2050 w2066 w2082 w2092 w2097 w2102]
      frame "", "Idle" {
        # "executes when the state queue is empty"
        n6 = event shown="[14] <RC SMO Public Events.State>: User Event" {
          selector: w19 -> [_ _ _ _ _ _ _ _ _ _ _ _ _ _ _ _ _ _ _ _ _ _ _ _ _ _ _ _ _ _ _ _ _ _ _ _ _ _ _ _ _ _ w444 _ _ _ _ _ _ _ _ _ _ _ _ _ _ _ _]
          dyn-events: _ -> [_ _ _ _ _ _ _ _ _ _ _ _ _ _ _ _ _ _ _ _ _ _ _ _ _ _ _ _ _ _ _ _ _ _ _ _ _ _ _ _ _ _ _ _ _ _ _ _ _ _ _ _ _ _ _ _ _ _ _]
          timeout: w20 -> [_ _ _ _ _ _ _ _ _ _ _ _ _ _ _ _ _ _ _ _ _ _ _ _ _ _ _ _ _ _ _ _ _ _ _ _ _ _ _ _ _ _ _ _ _ _ _ _ _ _ _ _ _ _ _ _ _ _ _]
          tunnel: w26 -> [w34 w53 w63 w93 w100 w108 w122 w139 w149 w158 w165 w171 w177 w192 w199 w206 w222 w227 w238 w244 w253 w262 w278 w306 w322 w335 w337 w347 w353 w357 w362 w367 w372 w377 w382 w387 w392 w397 w402 w407 w412 w421 w451 w499 w511 w521 w528 w536 w544 w551 w558 w564 w584 w593 w602 w611 w617 w623 w630]
          tunnel: [w32 w52 w62 w92 w99 w107 w121 w138 w148 w157 w164 w170 w176 w191 w198 w207 w223 w228 w237 w243 w254 w263 w279 w305 w321 w334 w338 w346 w352 w358 w363 w368 w373 w378 w383 w388 w393 w398 w403 w408 w413 w420 w450 w498 w510 w520 w527 w535 w543 w550 w557 w563 w583 w592 w601 w610 w616 w622 w634] -> w25
          tunnel: [w29 w45 w55 w85 w97 w103 w110 w131 w140 w155 w162 w168 w174 w186 w195 w203 w217 w224 w233 w242 w247 w255 w270 w299 w310 w328 w339 w345 w351 w355 w360 w365 w370 w375 w380 w385 w390 w395 w400 w405 w410 w419 w445 w497 w508 w518 w525 w533 w541 w548 w555 w562 w569 w591 w599 w608 w614 w619 w633] -> w24
          tunnel: w23 -> [w29 w46 w57 w86 w97 w103 w116 w133 w141 w155 w162 w168 w174 w186 w195 w203 w209 w224 w234 w242 w248 w255 w271 w301 w314 w328 w339 w345 w351 w355 w360 w365 w370 w375 w380 w385 w390 w395 w400 w405 w410 w419 w446 w497 w508 w518 w525 w533 w541 w548 w555 w562 w582 w591 w599 w608 w614 w620 w633]
          tunnel: [w33 w50 w61 w90 w95 w105 w120 w136 w146 w150 w163 w169 w172 w193 w200 w204 w220 w225 w236 w241 w252 w261 w276 w304 w319 w332 w340 w343 w349 w356 w361 w366 w371 w376 w381 w386 w391 w396 w401 w406 w411 w418 w449 w496 w509 w519 w526 w534 w542 w549 w556 w561 w573 w590 w600 w609 w615 w621 w632] -> w22
          tunnel: w21 -> [w33 w49 w60 w89 w96 w104 w119 w135 w145 w151 w163 w169 w172 w194 w200 w204 w218 w225 w232 w241 w250 w259 w273 w303 w318 w331 w340 w343 w349 w356 w361 w366 w371 w376 w381 w386 w391 w396 w401 w406 w411 w417 w448 w496 w509 w519 w526 w534 w542 w549 w556 w561 w573 w590 w600 w609 w615 w621 w632]
          event Timeout {
            n7 = event-data() -> ()  [unwired: 1 in, 1 out]
            n8 = Unbundle By Name(w33) -> ("Lockin"=w28:refnum<class "Instrument.Lockin.lvclass">)
            n9 = Unbundle By Name(w28) -> ("state"=w27:T35)
            n10 = case shown="\"idle\"" w27 {
              tunnel: [w37 w41 w43] -> w31
              frame "idle" {
                n11 = call "Spinner.vi"("Enum"=enum16{"Spinner 1", "Spinner 2", "Spinner 3"}."Spinner 1") -> ("Spinner Out"=w35:string)  [unwired: 4 in]
                n12 = Concatenate Strings("Idle     " ("Status"), w35) -> (w37:string)
              }
              frame "created" {
                n13 = call "Spinner.vi"("Enum"=enum16{"Spinner 1", "Spinner 2", "Spinner 3"}."Spinner 1") -> ("Spinner Out"=w39:string)  [unwired: 4 in]
                n14 = Concatenate Strings("Created  " ("Status"), w39) -> (w41:string)
              }
              frame Default {
                n15 = local read "Status"() -> (w43:string)
              }
            }
            "Status" <- w31
            n16 = call <vilib>:"Add State(s) to Queue__jki_lib_state_machine.vi"("State(s) in Front (\"\")"="" ("t"), "State(s) in (\"\")"=w34) -> ("States Out"=w32:string)  [unwired: 13 in]
          }
          event User Event {
            n17 = event-data() -> ("get AO"=w47:T36)  [unwired: 1 in, 4 out]
            n18 = Unbundle By Name(w49) -> ("Lockin"=w48:refnum<class "Instrument.Lockin.lvclass">)
            n19 = call "Write AO WFM.vi"("error in (no error)"=w46, "AO WFM"=w47, "Instrument.Lockin in"=w48) -> ("error out"=w45:errorcluster, "Instrument.Lockin out"=w44:refnum<class "Instrument.Lockin.lvclass">)  [unwired: 7 in]
            n20 = Bundle By Name(cluster=w49, "Lockin"=w44) -> (w50:T41)
            n21 = call <vilib>:"Add State(s) to Queue__jki_lib_state_machine.vi"("State(s) in Front (\"\")"="" ("State(s) in Front (\"\")"), "State(s) in (\"\")"=w53) -> ("States Out"=w52:string)  [unwired: 13 in]
          }
          event User Event {
            n22 = event-data() -> ("getAI"=w54:T42)  [unwired: 1 in, 4 out]
            n23 = Unbundle By Name(w60) -> ("Lockin"=w59:refnum<class "Instrument.Lockin.lvclass">)
            n24 = call "Write AI WFM.vi"("error in (no error)"=w57, "AI WFM"=w54, "Instrument.Lockin in"=w59) -> ("error out"=w56:errorcluster, "Instrument.Lockin out"=w58:refnum<class "Instrument.Lockin.lvclass">)  [unwired: 7 in]
            n25 = Bundle By Name(cluster=w60, "Lockin"=w58) -> (w61:T41)
            n26 = disable-structure shown="Enabled" {
              disable-tunnel: w56 -> [w70 w81]
              disable-tunnel: [w69 w81] -> w55
              disable-tunnel: w54 -> [w68 _]
              frame Enabled {
                n27 = Index Array(array=w68) -> (element=w80:waveform(dbl))  [unwired: 1 in]
                n28 = local read "Refresh time (ms)"() -> (w64:u32)
                n29 = call-poly <vilib>:"Waveform Duration.vi"("error in (no error)"=w70, "waveform in"=w80) -> ("error out"=w69:errorcluster, "duration"=w79:dbl)  [unwired: 7 in, 1 out]
                n30 = Multiply(x=w79, y=1000.0) -> (x*y=w66:dbl)
                n31 = Multiply(x=w66, y=2.0) -> (x*y=w65:dbl)
                n32 = Less?(x=w64, y=w65) -> (x < y?=w71:bool)
                n33 = Select(t=u32 6618880, s=w71, f=u32 16711680) -> (s? t:f=w75:u32)
                n34 = Select(t="Good", s=w71, f="#s/Fs: too small!") -> (s? t:f=→"Sampling Status":string)
                n35 = property on="Sampling Status" class="Str"("Text.BGColor"=w75) -> ()  [unwired: 2 in, 2 out]
              }
              frame Disabled {
              }
            }
            n36 = call <vilib>:"Add State(s) to Queue__jki_lib_state_machine.vi"("State(s) in (\"\")"=w63) -> ("States Out"=w62:string)  [unwired: 14 in]
          }
          event User Event {
            n37 = event-data() -> ("X"=w84:waveform(dbl)[], "Y"=w83:waveform(dbl)[])  [unwired: 1 in]
            n38 = Bundle("X"=w84, "Y"=w83) -> (w82:T43)  [unwired: 1 in]
            n39 = Unbundle By Name(w89) -> ("Lockin"=w88:refnum<class "Instrument.Lockin.lvclass">)
            n40 = call "Write REF WFM.vi"("error in (no error)"=w86, "Reference"=w82, "Instrument.Lockin in"=w88) -> ("error out"=w85:errorcluster, "Instrument.Lockin out"=w87:refnum<class "Instrument.Lockin.lvclass">)  [unwired: 7 in]
            n41 = Bundle By Name(cluster=w89, "Lockin"=w87) -> (w90:T41)
            n42 = call <vilib>:"Add State(s) to Queue__jki_lib_state_machine.vi"("State(s) in Front (\"\")"="" ("State(s) in Front (\"\")"), "State(s) in (\"\")"=w93) -> ("States Out"=w92:string)  [unwired: 13 in]
          }
          event User Event {
            n43 = event-data() -> ("getSweepResults"=w94:T39)  [unwired: 1 in, 4 out]
            n44 = Bundle By Name(cluster=w96, "SweepResults"=w94) -> (w95:T41)
            n45 = call <vilib>:"Add State(s) to Queue__jki_lib_state_machine.vi"("State(s) in Front (\"\")"="UI: Update Sweep Results Graphs" ("State(s) in Front (\"\")"), "State(s) in (\"\")"=w100) -> ("States Out"=w99:string)  [unwired: 13 in]
          }
          event User Event {
            n46 = event-data() -> ("Sweep_AO"=w102:waveform(dbl)[], "Sweep_AI"=w101:waveform(dbl)[])  [unwired: 1 in, 4 out]
            n47 = Bundle By Name(cluster=w104, "SweepWaveforms.Sweep_AO"=w102, "SweepWaveforms.Sweep_AI"=w101) -> (w105:T41)
            n48 = call <vilib>:"Add State(s) to Queue__jki_lib_state_machine.vi"("State(s) in Front (\"\")"="UI: Update Sweep WFMs Graphs" ("State(s) in Front (\"\")"), "State(s) in (\"\")"=w108) -> ("States Out"=w107:string)  [unwired: 13 in]
          }
          event User Event {
            n49 = event-data() -> ("Results"=w115:T44)  [unwired: 1 in, 4 out]
            n50 = Unbundle By Name(w119) -> ("Lockin"=w118:refnum<class "Instrument.Lockin.lvclass">)
            n51 = call "Write Results.vi"("error in (no error)"=w116, "Results"=w115, "Instrument.Lockin in"=w118) -> ("error out"=w112:errorcluster, "Instrument.Lockin out"=w117:refnum<class "Instrument.Lockin.lvclass">)  [unwired: 7 in]
            n52 = call <userlib>:"MGI Milliseconds Since Last Call.vi"("Error In"=w112) -> ("ms"=→"Refresh time (ms)":u32, "Error Out"=w110:errorcluster)  [unwired: 5 in]
            n53 = Bundle By Name(cluster=w119, "Lockin"=w117) -> (w120:T41)
            n54 = call <userlib>:"Periodic Trigger__ogtk.vi"("time (ms)"=u32 100) -> ("Triggered"=w114:bool)  [unwired: 12 in, 2 out]
            n55 = case shown="True" w114 {
              tunnel: ["" ("State(s) in Front (\"\")") w126] -> w109
              frame False {
              }
              frame True {
                n56 = local read "Tab Control 2"() -> (w127:T20)
                n57 = case shown="\"PS\"" w127 {
                  tunnel: ["" ("State(s) in Front (\"\")") "4461: FFT" ("State(s) in Front (\"\")")] -> w125
                  frame Default {
                  }
                  frame "PS" {
                  }
                }
                n58 = call <vilib>:"Add State(s) to Queue__jki_lib_state_machine.vi"("State(s) in Front (\"\")"="4461: OUT\nUI: Update Waveform Graphs\nUI: Sync AO AI Plot Visibility\nUI: Update Lockin Graphs\nUI: Sync Lockin Plot Visibility\nUI: Update Sweep Timer" ("State(s) in Front (\"\")"), "State(s) at Back (\"\")"=w125) -> ("States Out"=w126:string)  [unwired: 13 in]
              }
            }
            n59 = call <vilib>:"Add State(s) to Queue__jki_lib_state_machine.vi"("State(s) in Front (\"\")"=w109, "State(s) in (\"\")"=w122) -> ("States Out"=w121:string)  [unwired: 13 in]
          }
          event User Event {
            n60 = event-data() -> ("Channels: AO"=w130:T45)  [unwired: 1 in, 4 out]
            n61 = Unbundle By Name(w135) -> ("Lockin"=w134:refnum<class "Instrument.Lockin.lvclass">)
            n62 = call "Write Channels_ AO.vi"("error in (no error)"=w133, "Channels: AO"=w130, "Instrument.Lockin in"=w134) -> ("error out"=w131:errorcluster, "Instrument.Lockin out"=w132:refnum<class "Instrument.Lockin.lvclass">)  [unwired: 7 in]
            n63 = local write "AO Channels"(w130) -> ()
            n64 = Bundle By Name(cluster=w135, "Lockin"=w132) -> (w136:T41)
            n65 = call <vilib>:"Add State(s) to Queue__jki_lib_state_machine.vi"("State(s) in Front (\"\")"="" ("State(s) in Front (\"\")"), "State(s) in (\"\")"=w139) -> ("States Out"=w138:string)  [unwired: 13 in]
          }
          event User Event {
            n66 = event-data() -> ("Channels: REF"=w142:T46)  [unwired: 1 in, 4 out]
            n67 = Unbundle By Name(w145) -> ("Lockin"=w144:refnum<class "Instrument.Lockin.lvclass">)
            n68 = call "Write Channels_ REF.vi"("error in (no error)"=w141, "Channels: REF"=w142, "Instrument.Lockin in"=w144) -> ("error out"=w140:errorcluster, "Instrument.Lockin out"=w143:refnum<class "Instrument.Lockin.lvclass">)  [unwired: 7 in]
            n69 = Bundle By Name(cluster=w145, "Lockin"=w143) -> (w146:T41)
            n70 = call <vilib>:"Add State(s) to Queue__jki_lib_state_machine.vi"("State(s) in Front (\"\")"="" ("State(s) in Front (\"\")"), "State(s) in (\"\")"=w149) -> ("States Out"=w148:string)  [unwired: 13 in]
          }
          event User Event {
            n71 = event-data() -> ("state"=w152:T35)  [unwired: 1 in, 4 out]
            n72 = case shown="\"sweeping\"" w152 {
              frame Default {
              }
              frame "sweeping" {
                n73 = call <userlib>:"MGI Milliseconds Since Last Reset.vi"("Reset (F)"=TRUE) -> ()  [unwired: 5 in, 2 out]
              }
            }
            n74 = Unbundle By Name(w151) -> ("Lockin"=w154:refnum<class "Instrument.Lockin.lvclass">)
            n75 = Bundle By Name(cluster=w154, "state"=w152) -> (w153:refnum<class "Instrument.Lockin.lvclass">)
            n76 = Bundle By Name(cluster=w151, "Lockin"=w153) -> (w150:T41)
            n77 = call <vilib>:"Add State(s) to Queue__jki_lib_state_machine.vi"("State(s) in Front (\"\")"="UI: Update Status" ("State(s) in Front (\"\")"), "State(s) in (\"\")"=w158) -> ("States Out"=w157:string)  [unwired: 13 in]
          }
          event User Event {
            # "Check Calibrate Mode Button Value Change (pressed) Event"
            n78 = event-data() -> ("getCalibration"=→"Cal Info":T47)  [unwired: 1 in]
            n79 = call <vilib>:"Add State(s) to Queue__jki_lib_state_machine.vi"("State(s) in (\"\")"=w165, "State(s) at Back (\"\")"="" ("State(s) at Back (\"\")")) -> ("States Out"=w164:string)  [unwired: 13 in]
          }
          event User Event {
            # "Check Calibrate Mode Button Value Change (pressed) Event"
            n80 = event-data() -> ("getDAQconfig"=w166:T48)  [unwired: 1 in]
            n81 = property on="DAQ Config" class="Arr (strict)"("Val(Sgnl)"=w166) -> ()  [unwired: 2 in, 2 out]
            n82 = call <vilib>:"Add State(s) to Queue__jki_lib_state_machine.vi"("State(s) in (\"\")"=w171, "State(s) at Back (\"\")"="" ("State(s) at Back (\"\")")) -> ("States Out"=w170:string)  [unwired: 13 in]
          }
          event User Event {
            # "#framework\n????"
            n83 = event-data() -> ("SMO State"=w173:T16)  [unwired: 1 in]
            "LockinDAQ SMO State" <- w173
            n84 = case shown="Default" w173 {
              tunnel: ["UI: Enable Buttons" ("State Queue") "Lockin SMO: Stop\nLockin SMO: Start" ("State Queue")] -> w175
              frame "Started" {
              }
              frame Default {
              }
            }
            n85 = call <vilib>:"Add State(s) to Queue__jki_lib_state_machine.vi"("State(s) in Front (\"\")"=w175, "State(s) in (\"\")"=w177) -> ("States Out"=w176:string)  [unwired: 13 in]
          }
          event User Event {
            # "#framework"
            # "here command should be argument?"
            # "#todo: future: call Command: Handle Command"
            # "Message sent by the RemoteControl.lvclass:process"
            n86 = event-data() -> ("Message"=w187:T38, "Message.Command"=w183:string)  [unwired: 1 in, 3 out]
            n87 = Concatenate Strings("Command: ", w183) -> (w182:string)
            n88 = call <userlib>:"MGI String Pattern Match Exists.vi"("Patterns to Try"=string[] ["getAOconfig", "getSampling", "getREFconfig", "getInputGain", "getOutputGain", "getAO", "getAI", "getResults", "getStatus", "getSweepResults", "getSweepWaveforms", "getAutoSampling", "getState", "setAO", "setAO_Amplitude", "setAO_DC", "setAO_Frequency", "setAO_Phase", "setAO_Function", "setREF", "setREF_Frequency", "setREF_Phase", "setREF_TC", "setREF_RollOff", "setSweepConfiguration", "setState", "setSampling", "setSamplingMode", "setInputGain", "setOutputGain", "setDAQ", "HELP", "ACK", "getAll"] ("Array"), "String"=w183) -> ("Match Found"=w185:bool)  [unwired: 1 out]
            n89 = Select(t="Command: Handle Command" ("State(s) in Front (\"\")"), s=w185, f=w182) -> (s? t:f=w180:string)
            n90 = Bundle By Name(cluster=w194, "Message"=w187) -> (w193:T41)
            n91 = call <vilib>:"Add State(s) to Queue__jki_lib_state_machine.vi"("State(s) in Front (\"\")"=w180, "State(s) at Back (\"\")"="Remote SMO: Reply to Command") -> ("States Out"=w189:string)  [unwired: 13 in]
            n92 = call <vilib>:"Add State(s) to Queue__jki_lib_state_machine.vi"("State(s) in Front (\"\")"=w189, "State(s) in (\"\")"=w192) -> ("States Out"=w191:string)  [unwired: 13 in]
          }
          event User Event {
            # "Disable: I think this could cause an infinite loop when trying to exit"
            n93 = event-data() -> ("SMO State"=w196:T16)  [unwired: 1 in]
            "RC SMO State" <- w196
            n94 = case shown="Default" w196 {
              tunnel: ["" ("State Queue") "//Remote SMO: Stop\n//Remote SMO: Start" ("State Queue")] -> w197
              frame "Started" {
              }
              frame Default {
              }
            }
            n95 = call <vilib>:"Add State(s) to Queue__jki_lib_state_machine.vi"("State(s) in Front (\"\")"=w197, "State(s) in (\"\")"=w199) -> ("States Out"=w198:string)  [unwired: 13 in]
          }
          event Value Change {
            n96 = event-data() -> ()  [unwired: 1 in, 6 out]
            n97 = call <vilib>:"Add State(s) to Queue__jki_lib_state_machine.vi"("State(s) in Front (\"\")"="Configuration: Write" ("State(s) in Front (\"\")"), "State(s) in (\"\")"=w206) -> ("States Out"=w207:string)  [unwired: 13 in]
          }
          event "DAQ Config": Value Change {
            w212 = -1 items=["Default"=-1, "RSE"=10083, "Differential"=10106, "Pseudodifferential"=12529] ("output terminal configuration")
            w213 = -1 items=["Default"=-1, "RSE"=10083, "NRSE"=10078, "Differential"=10106, "Pseudodifferential"=12529] ("input terminal configuration")
            n98 = event-data() -> ("NewVal"=w211:T6[])  [unwired: 1 in]
            n99 = Unbundle By Name(w218) -> ("Lockin"=w214:refnum<class "Instrument.Lockin.lvclass">)
            n100 = call "config UI to not UI (AO and AI).vi"("output terminal configuration"=w212, "input terminal configuration"=w213, "New Ch []"=w211) -> ("AO Config"=w216:T49, "AI Config"=w210:T51)  [unwired: 7 in]
            n101 = call "Write AI Configuration.vi"("error in (no error)"=w209, "AI Configuration"=w210, "Instrument.Lockin in"=w214) -> ("error out"=w208:errorcluster, "Instrument.Lockin out"=w215:refnum<class "Instrument.Lockin.lvclass">)  [unwired: 7 in]
            n102 = call "Write AO Configuration.vi"("error in (no error)"=w208, "AO Configuration"=w216, "Instrument.Lockin in"=w215) -> ("error out"=w217:errorcluster, "Instrument.Lockin out"=w219:refnum<class "Instrument.Lockin.lvclass">)  [unwired: 7 in]
            n103 = Bundle By Name(cluster=w218, "Lockin"=w219) -> (w220:T41)
            n104 = call <vilib>:"Add State(s) to Queue__jki_lib_state_machine.vi"("State(s) in Front (\"\")"="Configuration: Write\nLockin SMO: Set AO Config\nLockin SMO: Set AI Config\nUI: Initialize REF Ch\nUI: Initialize AO Ch\nUI: Update AI Ch\nUI: Initialize Gains\nUI: Update Plot Names" ("State(s) in Front (\"\")"), "State(s) in (\"\")"=w222) -> ("States Out"=w223:string)  [unwired: 13 in]
          }
          event Value Change {
            n105 = event-data() -> ()  [unwired: 1 in, 1 out]
            n106 = call <vilib>:"Add State(s) to Queue__jki_lib_state_machine.vi"("State(s) in Front (\"\")"="Configuration: Write\nLockin SMO: Set AI Config" ("State(s) in Front (\"\")"), "State(s) in (\"\")"=w227) -> ("States Out"=w228:string)  [unwired: 13 in]
          }
          event Value Change {
            n107 = event-data() -> ("NewVal"=w231:T11)  [unwired: 1 in, 1 out]
            n108 = Unbundle By Name(w232) -> ("Lockin"=w230:refnum<class "Instrument.Lockin.lvclass">)
            n109 = call "Write sampling.vi"("error in (no error)"=w234, "sampling"=w231, "Instrument.Lockin in"=w230) -> ("error out"=w233:errorcluster, "Instrument.Lockin out"=w235:refnum<class "Instrument.Lockin.lvclass">)  [unwired: 7 in]
            n110 = Bundle By Name(cluster=w232, "Lockin"=w235) -> (w236:T41)
            n111 = call <vilib>:"Add State(s) to Queue__jki_lib_state_machine.vi"("State(s) in Front (\"\")"="Macro: Update Sampling" ("State(s) in Front (\"\")"), "State(s) in (\"\")"=w238) -> ("States Out"=w237:string)  [unwired: 13 in]
          }
          event "Auto x*F1", "Max Fs Refresh Rate (Hz)", "decimating factor": Value Change {
            n112 = event-data() -> ()  [unwired: 1 in, 6 out]
            n113 = call <vilib>:"Add State(s) to Queue__jki_lib_state_machine.vi"("State(s) in Front (\"\")"="Macro: Update Sampling" ("State(s) in Front (\"\")")) -> ("States Out"=w240:string)  [unwired: 14 in]
            n114 = call <vilib>:"Add State(s) to Queue__jki_lib_state_machine.vi"("State(s) in Front (\"\")"=w240, "State(s) in (\"\")"=w244) -> ("States Out"=w243:string)  [unwired: 13 in]
          }
          event "AO Channels": Value Change {
            n115 = event-data() -> ("NewVal"=w245:T3[])  [unwired: 1 in, 5 out]
            n116 = Unbundle By Name(w250) -> ("Lockin"=w249:refnum<class "Instrument.Lockin.lvclass">)
            n117 = call "Write Channels_ AO.vi"("error in (no error)"=w248, "Channels: AO"=w245, "Instrument.Lockin in"=w249) -> ("error out"=w247:errorcluster, "Instrument.Lockin out"=w246:refnum<class "Instrument.Lockin.lvclass">)  [unwired: 7 in]
            n118 = Bundle By Name(cluster=w250, "Lockin"=w246) -> (w252:T41)
            n119 = call <vilib>:"Add State(s) to Queue__jki_lib_state_machine.vi"("State(s) in Front (\"\")"="Data: Adjust Channels\nUI: Update Rings\nConfiguration: Write\nLockin SMO: Set AO" ("f"), "State(s) in (\"\")"=w253) -> ("States Out"=w254:string)  [unwired: 13 in]
          }
          event "AI Channels": Value Change {
            n120 = event-data() -> ("NewVal"=w256:T2[])  [unwired: 1 in]
            n121 = Unbundle By Name(w259) -> ("Lockin"=w258:refnum<class "Instrument.Lockin.lvclass">)
            n122 = Bundle By Name(cluster=w258, "AI Channels"=w256) -> (w257:refnum<class "Instrument.Lockin.lvclass">)
            n123 = Bundle By Name(cluster=w259, "Lockin"=w257) -> (w261:T41)
            n124 = call <vilib>:"Add State(s) to Queue__jki_lib_state_machine.vi"("State(s) in Front (\"\")"="UI: Update Rings\nConfiguration: Write\nLockin SMO: Set AI" ("f"), "State(s) in (\"\")"=w262) -> ("States Out"=w263:string)  [unwired: 13 in]
          }
          event "REF Channels": Value Change {
            # "#todo\nthis \"macro\" needs to\nbe handled by Lockin.DAQ\nor Handle Command"
            # "if number of lockin channels is not the same as before reset the lockin\nupdate: no, just reset phase...?"
            n125 = event-data() -> ("NewVal"=w266:T5[], "OldVal"=w267:T5[])  [unwired: 1 in]
            n126 = Unbundle By Name(w273) -> ("Lockin"=w272:refnum<class "Instrument.Lockin.lvclass">)
            n127 = Not Equal?(x=w266, y=w267) -> (x != y?=w268:bool)
            n128 = call "Write Channels_ REF.vi"("error in (no error)"=w271, "Channels: REF"=w266, "Instrument.Lockin in"=w272) -> ("error out"=w270:errorcluster, "Instrument.Lockin out"=w265:refnum<class "Instrument.Lockin.lvclass">)  [unwired: 7 in]
            n129 = Unbundle By Name(w265) -> ("state"=w264:T35)
            n130 = case shown="\"created\"" w264 {
              tunnel: ["" ("f") w287] -> _
              tunnel: w268 -> [_ w286]
              frame "idle", Default {
              }
              frame "created" {
                n131 = Format Into String(Set_State-enum."start" ("State")) -> (resulting string=w289:string)  [unwired: 3 in, 1 out]
                n132 = call <vilib>:"Build State String with Arguments__JKI_lib_State_Machine.vi"("Arguments (\"\")"=w289, "State"="Lockin SMO: Set State" ("f")) -> ("State with Arguments"=w292:string)  [unwired: 4 in]
                n133 = Select(t=w292, s=w286, f="") -> (s? t:f=w287:string)
              }
            }
            n134 = case shown="\"created\"" w264 {
              tunnel: ["" ("State with Arguments") w281] -> w274
              frame "idle", Default {
              }
              frame "created" {
                n135 = Format Into String(Set_State-enum."stop" ("State")) -> (resulting string=w284:string)  [unwired: 3 in, 1 out]
                n136 = call <vilib>:"Build State String with Arguments__JKI_lib_State_Machine.vi"("Arguments (\"\")"=w284, "State"="Lockin SMO: Set State" ("f")) -> ("State with Arguments"=w281:string)  [unwired: 4 in]
              }
            }
            n137 = Bundle By Name(cluster=w273, "Lockin"=w265) -> (w276:T41)
            n138 = Select(t=w274, s=w268, f="") -> ()  [unwired: 1 out]
            n139 = call <vilib>:"Add State(s) to Queue__jki_lib_state_machine.vi"("State(s) in (\"\")"="Data: Adjust Channels\nUI: Update Rings\nUI: Update Plot Names\nConfiguration: Write\nLockin SMO: Set REF\nLockin SMO: Reset Phase" ("f")) -> ("States Out"=w275:string)  [unwired: 14 in]
            n140 = call <vilib>:"Add State(s) to Queue__jki_lib_state_machine.vi"("State(s) in Front (\"\")"=w275, "State(s) in (\"\")"=w278) -> ("States Out"=w279:string)  [unwired: 13 in]
          }
          event "Input Gain": Value Change {
            n141 = event-data() -> ("NewVal"=w296:cluster{"AI.Ch":string, "Gain":dbl}[])  [unwired: 1 in, 5 out]
            n142 = for {
              tunnel: w296 -> [w308] mode=indexing
              tunnel: [w307] -> w295 mode=indexing
              n143 = Unbundle(w308) -> ("Gain"=w307:dbl)  [unwired: 1 out]
            }
            n144 = Unbundle By Name(w303) -> ("Lockin"=w302:refnum<class "Instrument.Lockin.lvclass">)
            n145 = call "Write Input Gain.vi"("error in (no error)"=w301, "InputGain"=w295, "Instrument.Lockin in"=w302) -> ("error out"=w300:errorcluster, "Instrument.Lockin out"=w298:refnum<class "Instrument.Lockin.lvclass">)  [unwired: 7 in]
            n146 = call "Initialize Input Gain.vi"("error in (no error)"=w300, "Instrument.Lockin"=w298) -> ("error out"=w299:errorcluster, "Input Gain"=w294:cluster{string, "Gain":dbl}[], "Instrument.Lockin out"=w297:refnum<class "Instrument.Lockin.lvclass">)  [unwired: 7 in]
            n147 = local write "Input Gain"(w294) -> ()
            n148 = Bundle By Name(cluster=w303, "Lockin"=w297) -> (w304:T41)
            n149 = call <vilib>:"Add State(s) to Queue__jki_lib_state_machine.vi"("State(s) in Front (\"\")"="Configuration: Write\nLockin SMO: Set Input Gain" ("State(s) in Front (\"\")"), "State(s) in (\"\")"=w306) -> ("States Out"=w305:string)  [unwired: 13 in]
          }
          event "Output Gain": Value Change {
            n150 = event-data() -> ("NewVal"=w317:cluster{"AI.Ch":string, "Gain":dbl}[])  [unwired: 1 in, 5 out]
            n151 = for {
              tunnel: w317 -> [w324] mode=indexing
              tunnel: [w323] -> w316 mode=indexing
              n152 = Unbundle(w324) -> ("Gain"=w323:dbl)  [unwired: 1 out]
            }
            n153 = Unbundle By Name(w318) -> ("Lockin"=w315:refnum<class "Instrument.Lockin.lvclass">)
            n154 = call "Write Output Gain.vi"("error in (no error)"=w314, "OutputGain"=w316, "Instrument.Lockin in"=w315) -> ("error out"=w312:errorcluster, "Instrument.Lockin out"=w313:refnum<class "Instrument.Lockin.lvclass">)  [unwired: 7 in]
            n155 = call "Initialize Ouput Gain.vi"("error in (no error)"=w312, "Instrument.Lockin"=w313) -> ("error out"=w310:errorcluster, "Ouput Gain"=w309:cluster{string, "Gain":dbl}[], "Instrument.Lockin out"=w311:refnum<class "Instrument.Lockin.lvclass">)  [unwired: 7 in]
            n156 = local write "Output Gain"(w309) -> ()
            n157 = Bundle By Name(cluster=w318, "Lockin"=w311) -> (w319:T41)
            n158 = call <vilib>:"Add State(s) to Queue__jki_lib_state_machine.vi"("State(s) in Front (\"\")"="Configuration: Write\nLockin SMO: Set Output Gain" ("State(s) in Front (\"\")"), "State(s) in (\"\")"=w322) -> ("States Out"=w321:string)  [unwired: 13 in]
          }
          event "Line", "Lowpass", "LP f (Hz)": Value Change {
            n159 = event-data() -> ()  [unwired: 1 in, 6 out]
            n160 = Unbundle By Name(w331) -> ("Lockin"=w330:refnum<class "Instrument.Lockin.lvclass">)
            n161 = Bundle By Name(cluster=w330, "60 Hz prefilter"="Line", "LP prefilter"="Lowpass", "LP cutoff (Hz)"="LP f (Hz)") -> (w329:refnum<class "Instrument.Lockin.lvclass">)
            n162 = Bundle By Name(cluster=w331, "Lockin"=w329) -> (w332:T41)
            n163 = call <vilib>:"Add State(s) to Queue__jki_lib_state_machine.vi"("State(s) in Front (\"\")"="Configuration: Write\nLockin SMO: Set Prefilter" ("State(s) in Front (\"\")"), "State(s) in (\"\")"=w335) -> ("States Out"=w334:string)  [unwired: 13 in]
          }
          event "Allowed remote system": Value Change {
            n164 = event-data() -> ()  [unwired: 1 in, 6 out]
            n165 = call <vilib>:"Add State(s) to Queue__jki_lib_state_machine.vi"("State(s) in Front (\"\")"="Remote SMO: AllowedRemote" ("State(s) in Front (\"\")"), "State(s) in (\"\")"=w337) -> ("States Out"=w338:string)  [unwired: 13 in]
          }
          event "Self Calibrate": Value Change {
            # "Self Calibrate Mode Button Value Change (pressed) Event"
            n166 = event-data() -> ()  [unwired: 1 in, 2 out]
            n167 = local write "Self Calibrate"(FALSE ("Self Calibrate")) -> ()
            n168 = property on="Pause" class="Bool (strict)"("Val(Sgnl)"=TRUE ("Value (Signaling)")) -> ()  [unwired: 2 in, 2 out]
            n169 = call <vilib>:"Add State(s) to Queue__jki_lib_state_machine.vi"("State(s) in Front (\"\")"="\nLockin SMO: Calibration >> True" ("f"), "State(s) in (\"\")"=w347) -> ("States Out"=w346:string)  [unwired: 13 in]
          }
          event "Get Calibration": Value Change {
            # "Self Calibrate Mode Button Value Change (pressed) Event"
            n170 = event-data() -> ()  [unwired: 1 in, 2 out]
            n171 = local write "Get Calibration"(FALSE ("Self Calibrate")) -> ()
            n172 = call <vilib>:"Add State(s) to Queue__jki_lib_state_machine.vi"("State(s) in Front (\"\")"="Lockin SMO: Calibration >> False" ("f"), "State(s) in (\"\")"=w353) -> ("States Out"=w352:string)  [unwired: 13 in]
          }
          event "X Axis": Value Change {
            # "X Axis, Y Axis Out Value Change (pressed) Event\ncall: UI: Update Waveform Graph Labels"
            n173 = event-data() -> ()  [unwired: 1 in, 6 out]
            n174 = call <vilib>:"Add State(s) to Queue__jki_lib_state_machine.vi"("State(s) in Front (\"\")"="UI: Update Waveform Graph Labels" ("State(s) in Front (\"\")"), "State(s) in (\"\")"=w357) -> ("States Out"=w358:string)  [unwired: 13 in]
          }
          event "Y Axis (Output)": Value Change {
            # "X Axis, Y Axis Out Value Change (pressed) Event\ncall: UI: Update Waveform Graph Labels"
            n175 = event-data() -> ()  [unwired: 1 in, 6 out]
            n176 = call <vilib>:"Add State(s) to Queue__jki_lib_state_machine.vi"("State(s) in Front (\"\")"="UI: Update Plot Names" ("State(s) in Front (\"\")"), "State(s) in (\"\")"=w362) -> ("States Out"=w363:string)  [unwired: 13 in]
          }
          event "AI Graph All": Value Change {
            # "X Axis, Y Axis Out Value Change (pressed) Event\ncall: UI: Update Waveform Graph Labels"
            n177 = event-data() -> ()  [unwired: 1 in, 6 out]
            n178 = call <vilib>:"Add State(s) to Queue__jki_lib_state_machine.vi"("State(s) in Front (\"\")"="UI: AI Graph Plot Visible >> All" ("State(s) in Front (\"\")"), "State(s) in (\"\")"=w367) -> ("States Out"=w368:string)  [unwired: 13 in]
          }
          event "AI Graph None": Value Change {
            # "X Axis, Y Axis Out Value Change (pressed) Event\ncall: UI: Update Waveform Graph Labels"
            n179 = event-data() -> ()  [unwired: 1 in, 6 out]
            n180 = call <vilib>:"Add State(s) to Queue__jki_lib_state_machine.vi"("State(s) in Front (\"\")"="UI: AI Graph Plot Visible >> None" ("State(s) in Front (\"\")"), "State(s) in (\"\")"=w372) -> ("States Out"=w373:string)  [unwired: 13 in]
          }
          event "AO Graph All": Value Change {
            # "X Axis, Y Axis Out Value Change (pressed) Event\ncall: UI: Update Waveform Graph Labels"
            n181 = event-data() -> ()  [unwired: 1 in, 6 out]
            n182 = call <vilib>:"Add State(s) to Queue__jki_lib_state_machine.vi"("State(s) in Front (\"\")"="UI: AO Graph Plot Visible >> All" ("State(s) in Front (\"\")"), "State(s) in (\"\")"=w377) -> ("States Out"=w378:string)  [unwired: 13 in]
          }
          event "AO Graph None": Value Change {
            # "X Axis, Y Axis Out Value Change (pressed) Event\ncall: UI: Update Waveform Graph Labels"
            n183 = event-data() -> ()  [unwired: 1 in, 6 out]
            n184 = call <vilib>:"Add State(s) to Queue__jki_lib_state_machine.vi"("State(s) in Front (\"\")"="UI: AO Graph Plot Visible >> None" ("State(s) in Front (\"\")"), "State(s) in (\"\")"=w382) -> ("States Out"=w383:string)  [unwired: 13 in]
          }
          event "Lockin 1 All": Value Change {
            # "X Axis, Y Axis Out Value Change (pressed) Event\ncall: UI: Update Waveform Graph Labels"
            n185 = event-data() -> ()  [unwired: 1 in, 6 out]
            n186 = call <vilib>:"Add State(s) to Queue__jki_lib_state_machine.vi"("State(s) in Front (\"\")"="UI: Lockin 1 Plot Visible >> All" ("State(s) in Front (\"\")"), "State(s) in (\"\")"=w387) -> ("States Out"=w388:string)  [unwired: 13 in]
          }
          event "Lockin 1 None": Value Change {
            # "X Axis, Y Axis Out Value Change (pressed) Event\ncall: UI: Update Waveform Graph Labels"
            n187 = event-data() -> ()  [unwired: 1 in, 6 out]
            n188 = call <vilib>:"Add State(s) to Queue__jki_lib_state_machine.vi"("State(s) in Front (\"\")"="UI: Lockin 1 Plot Visible >> None" ("State(s) in Front (\"\")"), "State(s) in (\"\")"=w392) -> ("States Out"=w393:string)  [unwired: 13 in]
          }
          event "Update": Value Change {
            # "Update Value Change (pressed) Event\ncall: AUX: Set AUX"
            n189 = event-data() -> ()  [unwired: 1 in, 6 out]
            n190 = call <vilib>:"Add State(s) to Queue__jki_lib_state_machine.vi"("State(s) in Front (\"\")"="AUX: Set AUX" ("State(s) in Front (\"\")"), "State(s) in (\"\")"=w397) -> ("States Out"=w398:string)  [unwired: 13 in]
          }
          event "Numeric", "X/R Range", "Y/Theta Range": Value Change {
            # "X&Y Axis Range\", \"XorR Axis Range\", \"YorTheta Axis Range\" Value Change (pressed) Event\ncall: UI: Update Lockin Graph Range"
            n191 = event-data() -> ()  [unwired: 1 in, 6 out]
            n192 = call <vilib>:"Add State(s) to Queue__jki_lib_state_machine.vi"("State(s) in Front (\"\")"="UI: Update Lockin Graph Range" ("State(s) in Front (\"\")"), "State(s) in (\"\")"=w402) -> ("States Out"=w403:string)  [unwired: 13 in]
          }
          event "Link Frequencies", "Limit Amplitudes", "AO freq link": Value Change {
            # "Same f\", \"Limit Amp\", \"AO freq link\": Value Change Value Change (pressed) Event\ncall:\nData: Adjust Channels\nConfiguration: Write\nLockin SMO: Set AO\nLockin SMO: Set REF"
            n193 = event-data() -> ()  [unwired: 1 in, 6 out]
            n194 = call <vilib>:"Add State(s) to Queue__jki_lib_state_machine.vi"("State(s) in Front (\"\")"="Data: Adjust Channels\nUI: Update Rings\nConfiguration: Write\nLockin SMO: Set AO\nLockin SMO: Set REF" ("f"), "State(s) in (\"\")"=w407) -> ("States Out"=w408:string)  [unwired: 13 in]
          }
          event Value Change {
            # "Display Value Change Value Change (pressed) Event\ncall:\nUI: Update Displays"
            n195 = event-data() -> ()  [unwired: 1 in, 6 out]
            n196 = call <vilib>:"Add State(s) to Queue__jki_lib_state_machine.vi"("State(s) in Front (\"\")"="UI: Update Displays" ("f"), "State(s) in (\"\")"=w412) -> ("States Out"=w413:string)  [unwired: 13 in]
          }
          event "Start": Value Change {
            # "Start Button Value Change (pressed) Event\nIf DAQ=idle:\n1. Set Sampling to Continuous Samples\n2. Start acquisition\n3. Set Pause=False\n4. Set timout=10\n\nIf DAQ=running:\n1. Do nothing"
            n197 = event-data() -> ()  [unwired: 1 in, 2 out]
            n198 = Unbundle By Name(w417) -> ("Lockin"=w415:refnum<class "Instrument.Lockin.lvclass">)
            n199 = Unbundle By Name(w415) -> ("state"=w414:T35)
            n200 = case shown="\"idle\", Default" w414 {
              tunnel: [w428 "" ("State with Arguments")] -> w416
              tunnel: w417 -> [w434 w440]
              tunnel: [w433 w440] -> w418
              frame "idle", Default {
                w429 = T53 10123 items=["Finite Samples"=10178, "Continuous Samples"=10123] ("Sample Mode")
                n201 = local write "Pause"(FALSE ("Pause")) -> ()
                n202 = Format Into String(w429) -> (resulting string=w430:string)  [unwired: 3 in, 1 out]
                n203 = Format Into String(Set_State-enum."start" ("State")) -> (resulting string=w438:string)  [unwired: 3 in, 1 out]
                n204 = First Call?() -> (First Call?: T/F=w425:bool)
                n205 = call <vilib>:"Build State String with Arguments__JKI_lib_State_Machine.vi"("Arguments (\"\")"=w430, "State"="Lockin SMO: Set Sampling" ("f")) -> ("State with Arguments"=w427:string)  [unwired: 4 in]
                n206 = call <vilib>:"Build State String with Arguments__JKI_lib_State_Machine.vi"("Arguments (\"\")"=w438, "State"="Lockin SMO: Set State" ("f")) -> ("State with Arguments"=w426:string)  [unwired: 4 in]
                n207 = Select(t="Macro: Update Sampling" ("f"), s=w425, f="") -> (s? t:f=w423:string)
                n208 = call <vilib>:"Add State(s) to Queue__jki_lib_state_machine.vi"("State(s) in Front (\"\")"=w423, "State(s) in (\"\")"=w427, "State(s) at Back (\"\")"=w426) -> ("States Out"=w428:string)  [unwired: 12 in]
                n209 = Bundle By Name(cluster=w434, "to"=-1) -> (w433:T41)
              }
              frame "created" {
              }
            }
            n210 = call <vilib>:"Add State(s) to Queue__jki_lib_state_machine.vi"("State(s) in (\"\")"=w421, "State(s) at Back (\"\")"=w416) -> ("States Out"=w420:string)  [unwired: 13 in]
          }
          event "Pause": Value Change {
            # "Pause Button Value Change (pressed) Event\nPause=True & DAQ=running:\n1. Set Sampling to Finite Samples\n2. STOP acquisition\n3. Set timeout=-1 (wait forever)\nPause=True & DAQ=idle\n1. Set timeout=-1\n2. Set Sampling to Finite\nPause=False:\n1. send T=Val(Sgnl) to Start"
            n211 = event-data() -> ("NewVal"=w447:bool)  [unwired: 1 in]
            n212 = Unbundle By Name(w448) -> ("Lockin"=w442:refnum<class "Instrument.Lockin.lvclass">)
            n213 = Unbundle By Name(w442) -> ("state"=w441:T35)
            n214 = Flush Event Queue(0:w444, 3:w446) -> (11:w445:errorcluster)  [unwired: 4 in, 2 out]
            n215 = case shown="True" w447 {
              tunnel: [w453 "" ("States Out")] -> w443
              tunnel: w448 -> [w455 w481]
              tunnel: [w454 w481] -> w449
              tunnel: w441 -> [w452 _]
              frame True {
                n216 = case shown="\"started\"" w452 {
                  tunnel: w455 -> [w460 w476]
                  tunnel: [w459 w475] -> w454
                  tunnel: [w456 w466] -> w453
                  frame "idle", Default {
                    w462 = T53 10178 items=["Finite Samples"=10178, "Continuous Samples"=10123] ("Sample Mode")
                    n217 = Format Into String(w462) -> (resulting string=w463:string)  [unwired: 3 in, 1 out]
                    n218 = call <vilib>:"Build State String with Arguments__JKI_lib_State_Machine.vi"("Arguments (\"\")"=w463, "State"="Lockin SMO: Set Sampling" ("f")) -> ("State with Arguments"=w457:string)  [unwired: 4 in]
                    n219 = call <vilib>:"Add State(s) to Queue__jki_lib_state_machine.vi"("State(s) at Back (\"\")"=w457) -> ("States Out"=w456:string)  [unwired: 14 in]
                    n220 = Bundle By Name(cluster=w460, "to"=100) -> (w459:T41)
                  }
                  frame "started" {
                    w471 = T53 10178 items=["Finite Samples"=10178, "Continuous Samples"=10123] ("Sample Mode")
                    n221 = Format Into String(Set_State-enum."stop" ("State")) -> (resulting string=w479:string)  [unwired: 3 in, 1 out]
                    n222 = Format Into String(w471) -> (resulting string=w472:string)  [unwired: 3 in, 1 out]
                    n223 = call <vilib>:"Build State String with Arguments__JKI_lib_State_Machine.vi"("Arguments (\"\")"=w479, "State"="Lockin SMO: Set State" ("f")) -> ("State with Arguments"=w464:string)  [unwired: 4 in]
                    n224 = call <vilib>:"Build State String with Arguments__JKI_lib_State_Machine.vi"("Arguments (\"\")"=w472, "State"="Lockin SMO: Set Sampling" ("f")) -> ("State with Arguments"=w465:string)  [unwired: 4 in]
                    n225 = local write "Status"("Finite Acquisition" ("Status")) -> ()
                    n226 = call <vilib>:"Add State(s) to Queue__jki_lib_state_machine.vi"("State(s) in Front (\"\")"="Lockin SMO: Set AO Zero Amplitude" ("f"), "State(s) in (\"\")"=w465, "State(s) at Back (\"\")"=w464) -> ("States Out"=w468:string)  [unwired: 12 in]
                    n227 = Bundle By Name(cluster=w476, "to"=100) -> (w475:T41)
                    n228 = call <vilib>:"Add State(s) to Queue__jki_lib_state_machine.vi"("State(s) in Front (\"\")"=w468, "State(s) at Back (\"\")"="Lockin SMO: Set AO" ("f")) -> ("States Out"=w466:string)  [unwired: 13 in]
                  }
                }
              }
              frame False {
                n229 = property on="Start" class="Bool (strict)"("Val(Sgnl)"=TRUE ("Value (Signaling)")) -> ()  [unwired: 2 in, 2 out]
              }
            }
            n230 = call <vilib>:"Add State(s) to Queue__jki_lib_state_machine.vi"("State(s) in Front (\"\")"=w443, "State(s) in (\"\")"=w451) -> ("States Out"=w450:string)  [unwired: 13 in]
          }
          event "Trigger": Value Change {
            w495 = T53 10178 items=["Finite Samples"=10178, "Continuous Samples"=10123] ("Sample Mode")
            # "Trigger Button Value Change (pressed) Event\nIf DAQ=idle:\n1. put into finite sample mode\n2. start (one) acquisition)\nIf DAQ=running:\n1. Stop current acquisition\n2. put into finite sample mode\n3. start (one) acquisition)"
            n231 = event-data() -> ()  [unwired: 1 in, 2 out]
            n232 = disable-structure shown="Disabled" {
              frame Disabled {
                n233 = local write "Trigger"(FALSE ("Trigger")) -> ()
              }
              frame Enabled {
              }
            }
            n234 = Unbundle By Name(w496) -> ("Lockin"=w483:refnum<class "Instrument.Lockin.lvclass">)
            n235 = Unbundle By Name(w483) -> ("state"=w484:T35)
            n236 = case shown="\"created\"" w484 {
              tunnel: ["" ("State with Arguments") w502] -> w487
              frame "idle", Default {
              }
              frame "created" {
                n237 = Format Into String(Set_State-enum."stop" ("State")) -> (resulting string=w505:string)  [unwired: 3 in, 1 out]
                n238 = call <vilib>:"Build State String with Arguments__JKI_lib_State_Machine.vi"("Arguments (\"\")"=w505, "State"="Lockin SMO: Set State" ("f")) -> ("State with Arguments"=w502:string)  [unwired: 4 in]
              }
            }
            n239 = local write "Pause"(TRUE ("Pause")) -> ()
            n240 = Format Into String(w495) -> (resulting string=w494:string)  [unwired: 3 in, 1 out]
            n241 = Format Into String(Set_State-enum."start" ("State")) -> (resulting string=w490:string)  [unwired: 3 in, 1 out]
            n242 = call <vilib>:"Build State String with Arguments__JKI_lib_State_Machine.vi"("Arguments (\"\")"=w494, "State"="Lockin SMO: Set Sampling" ("f")) -> ("State with Arguments"=w489:string)  [unwired: 4 in]
            n243 = call <vilib>:"Build State String with Arguments__JKI_lib_State_Machine.vi"("Arguments (\"\")"=w490, "State"="Lockin SMO: Set State" ("f")) -> ("State with Arguments"=w488:string)  [unwired: 4 in]
            n244 = call <vilib>:"Add State(s) to Queue__jki_lib_state_machine.vi"("State(s) in Front (\"\")"=w487, "State(s) in (\"\")"=w489, "State(s) at Back (\"\")"=w488) -> ("States Out"=w486:string)  [unwired: 12 in]
            n245 = call <vilib>:"Add State(s) to Queue__jki_lib_state_machine.vi"("State(s) in Front (\"\")"=w486, "State(s) in (\"\")"=w499) -> ("States Out"=w498:string)  [unwired: 13 in]
          }
          event "Reset": Value Change {
            # "RESET Button Value Change (pressed) Event\n1. Call 4461: SETUP State to calculate new Sampling\ninformation\n2. If sampling information changes, \"Sampling: value\nchange event will be triggered.\n3. Sampling: Value Change will call Stop, Set Sampling, Start"
            n246 = event-data() -> ()  [unwired: 1 in, 1 out]
            n247 = disable-structure shown="Disabled" {
              frame Disabled {
                n248 = Format Into String(Set_State-enum."reset" ("State")) -> (resulting string=w514:string)  [unwired: 3 in, 1 out]
                n249 = call <vilib>:"Build State String with Arguments__JKI_lib_State_Machine.vi"("Arguments (\"\")"=w514, "State"="Lockin SMO: Set State" ("f")) -> ()  [unwired: 4 in, 1 out]
              }
              frame Enabled {
              }
            }
            n250 = local write "Reset"(FALSE ("Reset")) -> ()
            n251 = call <vilib>:"Add State(s) to Queue__jki_lib_state_machine.vi"("State(s) in Front (\"\")"="Macro: Initialize UI\nMacro: Reset DAQ SMO\nMacro: Reset RC SMO\n//UI: Update Plot Names >>Reset" ("State(s) in Front (\"\")"), "State(s) in (\"\")"=w511) -> ("States Out"=w510:string)  [unwired: 13 in]
          }
          event "Measure": Value Change {
            # "Measure Offset Button Value Change (pressed) Event\n1. send \"measure offset\" command to DAQ"
            n252 = event-data() -> ()  [unwired: 1 in, 1 out]
            n253 = local write "Measure"(FALSE ("Measure\nOffset")) -> ()
            n254 = call <vilib>:"Add State(s) to Queue__jki_lib_state_machine.vi"("State(s) in Front (\"\")"="Lockin SMO: Measure Offset" ("State(s) in Front (\"\")")) -> ("States Out"=w517:string)  [unwired: 14 in]
            n255 = call <vilib>:"Add State(s) to Queue__jki_lib_state_machine.vi"("State(s) in Front (\"\")"=w517, "State(s) in (\"\")"=w521) -> ("States Out"=w520:string)  [unwired: 13 in]
          }
          event "Reset Phase": Value Change {
            # "Measure Offset Button Value Change (pressed) Event\n1. send \"measure offset\" command to DAQ"
            n256 = event-data() -> ()  [unwired: 1 in, 1 out]
            n257 = local write "Reset Phase"(FALSE ("Measure\nOffset")) -> ()
            n258 = call <vilib>:"Add State(s) to Queue__jki_lib_state_machine.vi"("State(s) in Front (\"\")"="Lockin SMO: Reset Phase" ("State(s) in Front (\"\")")) -> ("States Out"=w524:string)  [unwired: 14 in]
            n259 = call <vilib>:"Add State(s) to Queue__jki_lib_state_machine.vi"("State(s) in Front (\"\")"=w524, "State(s) in (\"\")"=w528) -> ("States Out"=w527:string)  [unwired: 13 in]
          }
          event "Disable all AI Ref": Value Change {
            # "Measure Offset Button Value Change (pressed) Event\n1. send \"measure offset\" command to DAQ"
            n260 = event-data() -> ()  [unwired: 1 in, 1 out]
            n261 = local write "Disable all AI Ref"(FALSE ("Measure\nOffset")) -> ()
            n262 = call <vilib>:"Build State String with Arguments__JKI_lib_State_Machine.vi"("Arguments (\"\")"="Disable" ("Arguments (\"\")"), "State"="UI: Update AI Reference Channels" ("State(s) in Front (\"\")")) -> ("State with Arguments"=w532:string)  [unwired: 4 in]
            n263 = call <vilib>:"Add State(s) to Queue__jki_lib_state_machine.vi"("State(s) in Front (\"\")"=w532, "State(s) in (\"\")"=w536) -> ("States Out"=w535:string)  [unwired: 13 in]
          }
          event "Enable only AI Ref1": Value Change {
            # "Measure Offset Button Value Change (pressed) Event\n1. send \"measure offset\" command to DAQ"
            n264 = event-data() -> ()  [unwired: 1 in, 1 out]
            n265 = local write "Enable only AI Ref1"(FALSE ("Measure\nOffset")) -> ()
            n266 = call <vilib>:"Build State String with Arguments__JKI_lib_State_Machine.vi"("Arguments (\"\")"="All 1" ("Arguments (\"\")"), "State"="UI: Update AI Reference Channels" ("State(s) in Front (\"\")")) -> ("State with Arguments"=w540:string)  [unwired: 4 in]
            n267 = call <vilib>:"Add State(s) to Queue__jki_lib_state_machine.vi"("State(s) in Front (\"\")"=w540, "State(s) in (\"\")"=w544) -> ("States Out"=w543:string)  [unwired: 13 in]
          }
          event "auto DAQ": Value Change {
            # "Measure Offset Button Value Change (pressed) Event\n1. send \"measure offset\" command to DAQ"
            n268 = event-data() -> ()  [unwired: 1 in, 1 out]
            n269 = local write "auto DAQ"(FALSE ("Measure\nOffset")) -> ()
            n270 = call <vilib>:"Add State(s) to Queue__jki_lib_state_machine.vi"("State(s) in Front (\"\")"="Lockin SMO: Auto DAQ" ("State(s) in Front (\"\")")) -> ("States Out"=w547:string)  [unwired: 14 in]
            n271 = call <vilib>:"Add State(s) to Queue__jki_lib_state_machine.vi"("State(s) in Front (\"\")"=w547, "State(s) in (\"\")"=w551) -> ("States Out"=w550:string)  [unwired: 13 in]
          }
          event "Remove": Value Change {
            # "Zero Offset Button Value Change (pressed) Event\n1. send \"zero offset\" command to DAQ"
            n272 = event-data() -> ()  [unwired: 1 in, 1 out]
            n273 = local write "Remove"(FALSE ("Zero\nOffset")) -> ()
            n274 = call <vilib>:"Add State(s) to Queue__jki_lib_state_machine.vi"("State(s) in Front (\"\")"="Lockin SMO: Remove Offset" ("State(s) in Front (\"\")")) -> ("States Out"=w554:string)  [unwired: 14 in]
            n275 = call <vilib>:"Add State(s) to Queue__jki_lib_state_machine.vi"("State(s) in Front (\"\")"=w554, "State(s) in (\"\")"=w558) -> ("States Out"=w557:string)  [unwired: 13 in]
          }
          event "Close": Value Change {
            w559 = "Macro: Exit"
            # "Stop Button Value Change (pressed) Event\n(this executes Macro: Exit to terminate the VI)"
            n276 = event-data() -> ("OldVal"=w560:bool)  [unwired: 1 in]
            n277 = local write "Close"(w560) -> ()
            n278 = disable-structure shown="Disabled" {
              disable-tunnel: w559 -> [w565 _]
              frame Disabled {
                n279 = Two Button Dialog(message="Are you sure you want to exit?") -> (T button?=w567:bool)  [unwired: 2 in]
                n280 = Select(t=w565, s=w567, f="") -> ()  [unwired: 1 out]
              }
              frame Enabled {
              }
            }
            n281 = call <vilib>:"Add State(s) to Queue__jki_lib_state_machine.vi"("State(s) in Front (\"\")"=w559, "State(s) in (\"\")"=w564) -> ("States Out"=w563:string)  [unwired: 13 in]
          }
          event "Start Sweep": Value Change {
            # "New Start Button Value Change (pressed) Event"
            n282 = event-data() -> ()  [unwired: 1 in, 1 out]
            n283 = Unbundle By Name(w573) -> ("Lockin.DAQ"=w571:refnum<class "Lockin.DAQ.lvclass">)
            n284 = Bundle By Name(cluster=T23 {"Sweep Time (s)"=0.0, "Initial Wait (s)"=0.0, "Return to Start"=FALSE, "Channels"=[]} ("Configure Sweep"), "Channels"="Channels: Sweep", "Sweep Time (s)"="Sweep Time (s)", "Initial Wait (s)"="Initial Wait (s)", "Return to Start"="Return to Start?") -> (w580:T23)
            n285 = call "Lockin.DAQ.setSweep.vi"("error in (no error)"=w582, "setSweep"=w580, "Lockin.DAQ"=w571) -> ("error out"=w569:errorcluster)  [unwired: 7 in, 1 out]
            n286 = Format Into String(Set_State-enum."start sweep" ("State")) -> (resulting string=w579:string)  [unwired: 3 in, 1 out]
            n287 = call <vilib>:"Build State String with Arguments__JKI_lib_State_Machine.vi"("Arguments (\"\")"=w579, "State"="Lockin SMO: Set State" ("f")) -> ("State with Arguments"=w576:string)  [unwired: 4 in]
            n288 = call <vilib>:"Add State(s) to Queue__jki_lib_state_machine.vi"("State(s) in Front (\"\")"=w576, "State(s) in (\"\")"=w584) -> ("States Out"=w583:string)  [unwired: 13 in]
          }
          event "Stop Sweep": Value Change {
            # "New Start Button Value Change (pressed) Event"
            n289 = event-data() -> ()  [unwired: 1 in, 6 out]
            n290 = local write "Stop Sweep"(FALSE ("Sweep Start")) -> ()
            n291 = Format Into String(Set_State-enum."stop sweep" ("State")) -> (resulting string=w588:string)  [unwired: 3 in, 1 out]
            n292 = call <vilib>:"Build State String with Arguments__JKI_lib_State_Machine.vi"("Arguments (\"\")"=w588, "State"="Lockin SMO: Set State" ("f")) -> ("State with Arguments"=w585:string)  [unwired: 4 in]
            n293 = call <vilib>:"Add State(s) to Queue__jki_lib_state_machine.vi"("State(s) in Front (\"\")"=w585, "State(s) in (\"\")"=w593) -> ("States Out"=w592:string)  [unwired: 13 in]
          }
          event "Load Configuration": Value Change {
            # "LOAD CONFIG Button Value Change (pressed) Event"
            n294 = event-data() -> ("NewVal"=w598:bool)  [unwired: 1 in, 1 out]
            n295 = local write "Load Configuration"(FALSE ("load config")) -> ()
            n296 = Select(t="Configuration: Read" ("State(s) at Back (\"\")"), s=w598, f="") -> (s? t:f=w595:string)
            n297 = call <vilib>:"Add State(s) to Queue__jki_lib_state_machine.vi"("State(s) in Front (\"\")"=w595, "State(s) in (\"\")"=w602) -> ("States Out"=w601:string)  [unwired: 13 in]
          }
          event "Save Configuration": Value Change {
            # "save config Button Value Change (pressed) Event"
            n298 = event-data() -> ("NewVal"=w605:bool)  [unwired: 1 in]
            n299 = local write "Save Configuration"(FALSE ("save config")) -> ()
            n300 = Select(t="Configuration: Write" ("State(s) at Back (\"\")"), s=w605, f="") -> (s? t:f=w606:string)
            n301 = call <vilib>:"Add State(s) to Queue__jki_lib_state_machine.vi"("State(s) in Front (\"\")"=w606, "State(s) in (\"\")"=w611) -> ("States Out"=w610:string)  [unwired: 13 in]
          }
          event "Save": Value Change {
            # "Save Mode Button Value Change (pressed) Event"
            n302 = event-data() -> ("OldVal"=w612:bool)  [unwired: 1 in]
            n303 = local write "Save"(w612) -> ()
            n304 = call <vilib>:"Add State(s) to Queue__jki_lib_state_machine.vi"("State(s) in (\"\")"=w617, "State(s) at Back (\"\")"="4461: SAVE") -> ("States Out"=w616:string)  [unwired: 13 in]
          }
          event "Help": Value Change {
            # "Help Button Value Change (pressed) Event\nIf Help = True: Send user to help webpage; Set Help=False\nIf Help=Fale, Do nothing"
            n305 = event-data() -> ("NewVal"=w618:bool)  [unwired: 1 in]
            n306 = case shown="False" w618 {
              tunnel: w620 -> [w624 w628]
              tunnel: [w624 w626] -> w619
              frame False {
              }
              frame True {
                n307 = local write "Help"(FALSE ("Help")) -> ()
                n308 = call-poly <vilib>:"Open URL in Default Browser.vi"("error in (no error)"=w628, "URL"="https://app.asana.com/0/205665857037275/list") -> ("error out"=w626:errorcluster)  [unwired: 4 in, 1 out]
              }
            }
            n309 = call <vilib>:"Add State(s) to Queue__jki_lib_state_machine.vi"("State(s) in (\"\")"=w623) -> ("States Out"=w622:string)  [unwired: 14 in]
          }
          event Panel Close? {
            w629 = "Macro: Exit"
            # "Discard the event because we'll close the front panel ourselves in Macro: Exit"
            # "Close Panel button (pressed) Event\n(this executes Macro: Exit to terminate the VI)"
            n310 = event-data() -> ()  [unwired: 1 in, 1 out]
            n311 = disable-structure shown="Disabled" {
              disable-tunnel: w629 -> [w635 _]
              frame Disabled {
                n312 = Two Button Dialog(message="Are you sure you want to exit?") -> (T button?=w637:bool)  [unwired: 2 in]
                n313 = Select(t=w635, s=w637, f="") -> ()  [unwired: 1 out]
              }
              frame Enabled {
              }
            }
            n314 = call <vilib>:"Add State(s) to Queue__jki_lib_state_machine.vi"("State(s) in Front (\"\")"=w629, "State(s) in (\"\")"=w630) -> ("States Out"=w634:string)  [unwired: 13 in]
            n315 = event-data("Discard?"=TRUE) -> ()  [unwired: 1 in, 1 out]
          }
        }
      }
      frame "---------- Core ----------" {
        # "Do not put any code in this frame.\n(it is a separator no-op)"
        n316 = call <vilib>:"Add State(s) to Queue__jki_lib_state_machine.vi"("State(s) in (\"\")"=w643) -> ("States Out"=w642:string)  [unwired: 14 in]
      }
      frame Default {
        w655 = 42 items=["No error", "Argument error", "Memory is full", "Out of zone", "End of file", "File already open", "Generic file I/O error", "File not found", "File permission error", "Disk is full", "Duplicate path", "Too many files open", "System feature not enabled", "Resource file not found", "Cannot add resource", "Resource not found", "Image not found", "Image memory error", "Pen does not exist", "Config type invalid", "Config token not found", "Config parse error", "Config memory error", "Bad external code format", "Bad external code offset", "External code not present", "Null window", "Destroy window error", "Null menu", "Print aborted", "Bad print record", "Print driver error", "Windows error during printing", "Memory error during printing", "Print dialog error", "Generic print error", "Invalid device refnum", "Device not found", "Device parameter error", "Device unit error", "Cannot open device", "Device call aborted", "Generic error", "Cancelled by user", "Object ID too low", "Object ID too high", "Object not in heap", "Unknown heap", "Unknown object (invalid DefProc)", "Unknown object (DefProc not in table)", "Message out of range", "Invalid (null) method", "Unknown message", "Manager call not supported", "Bad address", "Network operation in progress", "Network operation timed out", "Connection is busy", "Network attribute not supported", "Network error", "Address in use", "System out of memory", "Connection aborted", "Connection refused", "Not connected", "Already connected", "Connection closed", "Initialization error (interapplication manager)", "Bad occurrence", "Wait on unbound occurrence handler", "Occurrence queue overflow", "Datalog type conflict", "Unused", "Unrecognized type (interapplication manager)", "Memory corrupt", "Failed to make temporary DLL", "Old CIN version", "Drag socket not found", "Failed to load drop-object", "Failed to register OLE object", "Failed to release OLE object", "Format specifier type mismatch", "Unknown format specifier", "Too few format specifiers", "Too many format specifiers", "Scan failed", "Newer CIN version", "Error converting to variant", "Runtime menu error", "Password tampered", "Variant attribute not found", "Incompatible variant data type", "Event data is not available", "Event Store is not present", "Occurrence is not found", "Event Queue is not created", "Event info is not available", "Refnum passed is NULL", "Error retrieving Class GUID", "Error retrieving CoClass GUID", "Error retrieving TypeLib GUID.", "Bad built application magic bytes.", "Specific driver is different from the specific driver associated with the Logical Name.", "There is no session opened to the class driver.", "Max Error", "MAX - Error with config objects", "MAX - Error loading configuration", "MAX - Group not supported"]
        # "Current State"
        # "Do not delete, rename, or modify this frame.\n(this is used to capture unhandled states and typos)"
        # "Handle mistyped state name (developer tool)"
        n317 = Format Into String(format string="Software Exception: Unhandled State \"%s\"." ("message"), error in=w651, w646) -> (resulting string=w654:string, error out=w653:errorcluster)  [unwired: 1 in]
        n318 = call <vilib>:"Error Cluster From Error Code.vi"("show call chain? (False)"=TRUE, "error in (no error)"=w653, "error message (\"\")"=w654, "error code (0)"=w655) -> ("error out"=w652:errorcluster)  [unwired: 5 in]
        n319 = call <vilib>:"Add State(s) to Queue__jki_lib_state_machine.vi"("State(s) in (\"\")"=w650) -> ("States Out"=w649:string)  [unwired: 14 in]
      }
      frame "Initialize Core Data" {
        # "Do not delete, rename, or modify this frame.\n(this is used to determine panel behavior on exit)"
        # "originally closed?"
        # "exe?"
        # "If panel starts closed or is an EXE, then close it when we exit"
        n320 = property class="VI"() -> ("Front Panel.Open"=w664:bool)  [unwired: 2 in, 2 out]
        n321 = property class="App"() -> ("App.Kind"=w663:T24)  [unwired: 2 in, 2 out]
        n322 = control-ref of="Current VI Reference"() -> (w657:refnum<vi>)
        n323 = Not(x=w664) -> (.not. x?=w661:bool)
        n324 = Equal?(x=w663, y=T24."Run Time System" ("Application:Kind")) -> (x = y?=w660:bool)
        n325 = Or(x=w661, y=w660) -> (x .or. y?=w658:bool)
        n326 = Bundle By Name(cluster=w659, "Core.Current VI Reference"=w657, "Core.Close Panel on Exit?"=w658) -> (w666:T41)
        n327 = call <vilib>:"Add State(s) to Queue__jki_lib_state_machine.vi"("State(s) in (\"\")"=w668) -> ("States Out"=w667:string)  [unwired: 14 in]
      }
      frame "Error Handler" {
        # "Handle any errors here.\nYou can also output any states to clean-up after errors occur"
        # "Clear error"
        n328 = Unbundle By Name(w673) -> ("Lockin"=w672:refnum<class "Instrument.Lockin.lvclass">)
        n329 = call-dynamic "Handle Error.vi"("Stop on Unhandled Error (T)"=FALSE, "error in"=w670, "SMO"=w672) -> ("handling error"=w669:errorcluster)  [unwired: 6 in, 2 out]
        n330 = call-poly <userlib>:"Filter Error Codes__ogtk.vi"("Error In"=w669, "Error Codes to Filter"=i32[] [-200077, -200462, -200245, -200279]) -> ("Error Out"=w677:errorcluster)  [unwired: 7 in, 2 out]
        n331 = case shown="Error" w677 {
          selector: w677 -> [w682 w687]
          tunnel: ["" "Macro: Exit"] -> w679
          tunnel: [w682 w684] -> w675
          frame No Error {
          }
          frame Error {
            w685 = T54 1 items=["no dialog", "OK message", "continue or stop message", "OK message + warnings", "continue/stop + warnings"] ("type of dialog (OK msg:1)")
            # "Unhandled Error -- Display it"
            n332 = call <vilib>:"General Error Handler.vi"("type of dialog (OK msg:1)"=w685, "error in (no error)"=w687) -> ("error out"=w684:errorcluster)  [unwired: 9 in, 4 out]
          }
        }
        n333 = call <userlib>:"Clear All Errors__ogtk.vi"("Error In"=w675) -> ("Error Out"=w674:errorcluster)  [unwired: 3 in]
        n334 = call <vilib>:"Add State(s) to Queue__jki_lib_state_machine.vi"("State(s) in Front (\"\")"=w679, "State(s) in (\"\")"=w681) -> ("States Out"=w680:string)  [unwired: 13 in]
      }
      frame "Exit" {
        # "Do not put any code in this frame.\n(No errors that occur here will be handled.)"
        n335 = call <vilib>:"Add State(s) to Queue__jki_lib_state_machine.vi"("State(s) in (\"\")"=w693) -> ("States Out"=w692:string)  [unwired: 14 in]
      }
      frame "---------- Data ----------" {
        # "Do not put any code in this frame.\n(It is a separator no-op. You can make a copy of this frame to create a new Data frame)"
        n336 = call <vilib>:"Add State(s) to Queue__jki_lib_state_machine.vi"("State(s) in (\"\")"=w698) -> ("States Out"=w697:string)  [unwired: 14 in]
      }
      frame "Data: Initialize" {
        w699 = T38 {"Command"="", "Data"=variant, "ID"=""}  # Message
        w700 = refnum<class "Logger.Error.lvclass"> refnum  # Logger.Error
        w703 = refnum<class "Lockin.DAQ.lvclass"> refnum  # Lockin.DAQ
        w706 = T40 {"Sweep_AO"=[], "Sweep_AI"=[]}  # SweepWaveforms
        w707 = T39 {"X results"=[], "Y Results"=[]}  # SweepResults
        w709 = T37 {"address"="", "Port"=0, "AllowedRemote"="", "Commands"=[], "timeout"=0}  # RemoteControl.Configure
        (unwired) T44 {"Time Stamp"=timestamp(0 s since 1904-01-01), "Results (Dictionary)"=[]}  # Results
        w710 = T38 {"Command"="", "Data"=variant, "ID"=""}  # HandledMessage
        w702 = refnum<class "Instrument.Lockin.lvclass"> refnum  # Lockin
        w701 = refnum<class "RemoteControl.lvclass"> refnum  # RemoteControl
        (unwired) waveform(dbl)[] []  # AI WFM
        w704 = 100  # to
        (unwired) waveform(dbl)[] []  # AO WFM
        (unwired) waveform(dbl)[] []  # REF WFM
        w712 = T55 {"Current VI Reference"=refnum, "Close Panel on Exit?"=FALSE}  # Core
        # "#todo\nPut all of this stuff on the class wire\nso I can use Handle Command.vi..."
        # "is sent to RC:process"
        # "comes from RC:process"
        # "do not delete - used by framework"
        # "Initialize the shift-register data, here.\n(data names are defined by what you wire into the bundle function)"
        n337 = call <vilib>:"Add State(s) to Queue__jki_lib_state_machine.vi"("State(s) in (\"\")"=w714) -> ("States Out"=w713:string)  [unwired: 14 in]
        n338 = Bundle("Core"=w712, "to"=w704, "Lockin"=w702, "RemoteControl"=w701, "Lockin.DAQ"=w703, "Logger.Error"=w700, "RemoteControl.Configure"=w709, "Message"=w699, "HandledMessage"=w710, "SweepResults"=w707, "SweepWaveforms"=w706) -> (w708:T41)  [unwired: 1 in]
      }
      frame "Data: Adjust Channels" {
        # "#todo\nshould some of these methods be owned by Lockin.DAQ?"
        n339 = Unbundle By Name(w721) -> ("Lockin"=w722:refnum<class "Instrument.Lockin.lvclass">)
        n340 = call "Initialize REF Channels.vi"("error in (no error)"=w723, "Instrument.Lockin"=w722) -> ("error out"=w724:errorcluster, "Instrument.Lockin out"=w725:refnum<class "Instrument.Lockin.lvclass">)  [unwired: 7 in, 1 out]
        n341 = call "Initialize AO Channels.vi"("error in (no error)"=w724, "Instrument.Lockin"=w725) -> ("error out"=w729:errorcluster, "Instrument.Lockin out"=w731:refnum<class "Instrument.Lockin.lvclass">)  [unwired: 7 in, 1 out]
        n342 = call "Limit AO Amplitude.vi"("error in (no error)"=w729, "Limit Amplitudes"="Limit Amplitudes", "AO Amp Limit"="AO Amp Limit", "Instrument.Lockin in"=w731) -> ("error out"=w728:errorcluster, "Instrument.Lockin out"=w730:refnum<class "Instrument.Lockin.lvclass">)  [unwired: 6 in]
        n343 = call "Set all f same.vi"("error in (no error)"=w728, "Link Frequencies"="Link Frequencies", "AO f"="AO freq link", "Instrument.Lockin"=w730) -> ("error out"=w716:errorcluster, "Instrument.Lockin out"=w726:refnum<class "Instrument.Lockin.lvclass">)  [unwired: 6 in]
        n344 = Unbundle By Name(w726) -> ("AO Channels"=w715:T45, "REF Channels"=w732:T46)
        n345 = Bundle By Name(cluster=w721, "Lockin"=w726) -> (w720:T41)
        n346 = local write "REF Channels"(w732) -> ()
        n347 = local write "AO Channels"(w715) -> ()
        n348 = call <vilib>:"Add State(s) to Queue__jki_lib_state_machine.vi"("State(s) in (\"\")"=w735) -> ("States Out"=w734:string)  [unwired: 14 in]
      }
      frame "Data: Cleanup" {
        # "Cleanup any data and references, here.\n(this is called automatically, by the Macro: Exit)"
        n349 = Unbundle By Name(w737) -> ("Core.Current VI Reference"=w739:refnum<vi>)
        n350 = Close Reference(reference=w739, error in (no error)=w738) -> (error out=w736:errorcluster)
        n351 = call <vilib>:"Add State(s) to Queue__jki_lib_state_machine.vi"("State(s) in (\"\")"=w742) -> ("States Out"=w741:string)  [unwired: 14 in]
      }
      frame "---------- Events ----------" {
        # "Template Separator\n(You can make a copy of, or modify, this frame)"
        n352 = call <vilib>:"Add State(s) to Queue__jki_lib_state_machine.vi"("State(s) in (\"\")"=w747) -> ("States Out"=w746:string)  [unwired: 14 in]
      }
      frame "Events: Register" {
        w756 = T56 {"Error"=refnum, "State"=refnum, "Reserve State"=refnum}  # LockinDAQ SMO Public Events
        w765 = T56 {"Error"=refnum, "State"=refnum, "Reserve State"=refnum}  # RC SMO Public Events
        n353 = Unbundle By Name(w769) -> ("RemoteControl"=w761:refnum<class "RemoteControl.lvclass">, "Lockin.DAQ"=w748:refnum<class "Lockin.DAQ.lvclass">)
        n354 = call <vilib>:"GetPublicEvents.vi"("SMO"=w761) -> ("error out"=w760:errorcluster, "Public Events"=w764:T56, "SMO out"=w758:refnum<class "RemoteControl.lvclass">)  [unwired: 8 in]
        n355 = Variant To Data(error in=w760, type=w765, Variant=w764) -> (data=w763:T56, error out=w759:errorcluster)
        n356 = call <vilib>:"GetPublicEvents.vi"("SMO"=w748) -> ("error out"=w753:errorcluster, "Public Events"=w755:T56, "SMO out"=w751:refnum<class "Lockin.DAQ.lvclass">)  [unwired: 8 in]
        n357 = call <userlib>:"RemoteControl.GetPublicEvents.vi"("RemoteControl"=w758) -> ("error out"=w757:errorcluster, "RC Public Events"=w768:T57)  [unwired: 8 in, 1 out]
        n358 = Variant To Data(error in=w753, type=w756, Variant=w755) -> (data=w754:T56, error out=w752:errorcluster)
        n359 = call "Lockin.DAQ.GetPublicEvents.vi"("Lockin.DAQ"=w751) -> ("error out"=w766:errorcluster, "LIADAQ Public Events"=w762:T58)  [unwired: 8 in, 1 out]
        n360 = register-events(w763, w768, w754, w762) -> (reference out=w770:refnum<event-registration>, error out=w767:errorcluster)  [unwired: 2 in]
        n361 = Merge Errors(w767, w766, w757, w752, w759, w749) -> (w750:errorcluster)
        n362 = call <vilib>:"Add State(s) to Queue__jki_lib_state_machine.vi"("State(s) in (\"\")"=w772) -> ("States Out"=w771:string)  [unwired: 14 in]
      }
      frame "Events: Unregister" {
        n363 = Unregister For Events(event registration refnum=w774, error in=w773) -> (error out=w775:errorcluster)
        n364 = call <vilib>:"Clear Errors.vi"("error in (no error)"=w775) -> ()  [unwired: 5 in, 2 out]
        n365 = call <vilib>:"Add State(s) to Queue__jki_lib_state_machine.vi"("State(s) in (\"\")"=w778) -> ("States Out"=w777:string)  [unwired: 14 in]
      }
      frame "---------- UI ----------" {
        # "Do not put any code in this frame.\n(It is a separator no-op. You can make a copy of this frame to create a new UI frame)"
        n366 = call <vilib>:"Add State(s) to Queue__jki_lib_state_machine.vi"("State(s) in (\"\")"=w783) -> ("States Out"=w782:string)  [unwired: 14 in]
      }
      frame "UI: Initialize" {
        w784 = waveform(dbl)[][] [] ("History Data")
        # "Initialize the User Interface, here.\n(this is called automatically, by the Macro: Init)"
        n367 = call <userlib>:"MGI Get Executable Version.vi"() -> ("Version"=w789:string)  [unwired: 7 in]
        n368 = Empty String/Path?(string/path=w789) -> (empty?=w790:bool)
        n369 = invoke on="Start" class="Bool (strict)" method="Reinit To Default"() -> ()  [unwired: 3 in, 3 out]
        n370 = invoke on="Start Sweep" class="Bool (strict)" method="Reinit To Default"() -> ()  [unwired: 3 in, 3 out]
        n371 = Select(t=w786, s=w790, f=w789) -> (s? t:f=w788:string)
        n372 = Format Into String(format string="v%s", w788) -> (resulting string=→"Version":string)  [unwired: 2 in, 1 out]
        n373 = invoke on="Reset" class="Bool (strict)" method="Reinit To Default"() -> ()  [unwired: 3 in, 3 out]
        n374 = invoke on="Close" class="Bool (strict)" method="Reinit To Default"() -> ()  [unwired: 3 in, 3 out]
        n375 = property on="Lockin 1" class="WFChart (strict)"("History Data"=w784) -> ()  [unwired: 2 in, 2 out]
        n376 = local write "Tab Control 2"(T20."AO/AI Display" ("Tab Control 2")) -> ()
        n377 = local write "Tab Control 4"(T1."AO/REF Setup" ("Tab Control 4")) -> ()
        n378 = property on="Lockin 2" class="WFChart (strict)"("History Data"=w784) -> ()  [unwired: 2 in, 2 out]
        n379 = local write "Status"("Starting" ("Status")) -> ()
        n380 = invoke on="Trigger" class="Bool (strict)" method="Reinit To Default"() -> ()  [unwired: 3 in, 3 out]
        n381 = invoke on="Help" class="Bool (strict)" method="Reinit To Default"() -> ()  [unwired: 3 in, 3 out]
        n382 = call <userlib>:"Fit VI window to Largest Dec__ogtk.vi"("error in (no error)"=w793) -> ("error out"=w795:errorcluster)  [unwired: 5 in, 1 out]
        n383 = call <vilib>:"Add State(s) to Queue__jki_lib_state_machine.vi"("State(s) in (\"\")"=w799) -> ("States Out"=w798:string)  [unwired: 14 in]
      }
      frame "UI: Initialize REF Ch" {
        n384 = Unbundle By Name(w806) -> ("Lockin"=w805:refnum<class "Instrument.Lockin.lvclass">)
        n385 = call "Initialize REF Channels.vi"("error in (no error)"=w803, "Instrument.Lockin"=w805) -> ("error out"=w801:errorcluster, "REF Channels out"=w802:T46, "Instrument.Lockin out"=w804:refnum<class "Instrument.Lockin.lvclass">)  [unwired: 7 in]
        n386 = property on="REF Channels" class="Arr (strict)"(error in=w801, "Val(Sgnl)"=w802) -> (error out=w800:errorcluster)  [unwired: 1 in, 1 out]
        n387 = Bundle By Name(cluster=w806, "Lockin"=w804) -> (w807:T41)
        n388 = call <vilib>:"Add State(s) to Queue__jki_lib_state_machine.vi"("State(s) in (\"\")"=w810) -> ("States Out"=w809:string)  [unwired: 14 in]
      }
      frame "UI: Initialize AO Ch" {
        n389 = Unbundle By Name(w817) -> ("Lockin"=w816:refnum<class "Instrument.Lockin.lvclass">)
        n390 = call "Initialize AO Channels.vi"("error in (no error)"=w814, "Instrument.Lockin"=w816) -> ("error out"=w813:errorcluster, "Channels: AO"=w812:T45, "Instrument.Lockin out"=w815:refnum<class "Instrument.Lockin.lvclass">)  [unwired: 7 in]
        n391 = property on="AO Channels" class="Arr (strict)"(error in=w813, "Val(Sgnl)"=w812) -> (error out=w811:errorcluster)  [unwired: 1 in, 1 out]
        n392 = Bundle By Name(cluster=w817, "Lockin"=w815) -> (w818:T41)
        n393 = call <vilib>:"Add State(s) to Queue__jki_lib_state_machine.vi"("State(s) in (\"\")"=w821) -> ("States Out"=w820:string)  [unwired: 14 in]
      }
      frame "UI: Update AI Ch" {
        # "Add or remove AI channels"
        n394 = Unbundle By Name(w828) -> ("Lockin"=w826:refnum<class "Instrument.Lockin.lvclass">)
        n395 = call "Initialize AI Channels.vi"("error in (no error)"=w825, "Instrument.Lockin"=w826) -> ("error out"=w824:errorcluster, "AI Channels"=w827:T2[], "Instrument.Lockin out"=w822:refnum<class "Instrument.Lockin.lvclass">)  [unwired: 7 in]
        n396 = property on="AI Channels" class="Arr (strict)"(error in=w824, "Val(Sgnl)"=w827) -> (error out=w823:errorcluster)  [unwired: 1 in, 1 out]
        n397 = Bundle By Name(cluster=w828, "Lockin"=w822) -> (w829:T41)
        n398 = call <vilib>:"Add State(s) to Queue__jki_lib_state_machine.vi"("State(s) in (\"\")"=w832) -> ("States Out"=w831:string)  [unwired: 14 in]
      }
      frame "UI: Update AI Reference Channels" {
        # "Add or remove AI channels"
        n399 = Unbundle By Name(w841) -> ("Lockin"=w838:refnum<class "Instrument.Lockin.lvclass">)
        n400 = case shown="\"All 1\"" w833 {
          tunnel: [u16[] [1] ("References") u16[] [0] ("References")] -> w834
          frame "All 1" {
          }
          frame "Disable", Default {
          }
        }
        n401 = Unbundle By Name(w838) -> ("AI Channels"=w839:T59)
        n402 = for {
          tunnel: w839 -> [w850] mode=indexing
          tunnel: [w849] -> w837 mode=indexing
          tunnel: w834 -> [w848]
          n403 = Bundle By Name(cluster=w850, "References"=w848) -> (w849:T2)
        }
        n404 = Bundle By Name(cluster=w838, "AI Channels"=w837) -> (w836:refnum<class "Instrument.Lockin.lvclass">)
        n405 = property on="AI Channels" class="Arr (strict)"(error in=w835, "Val(Sgnl)"=w837) -> (error out=w840:errorcluster)  [unwired: 1 in, 1 out]
        n406 = Bundle By Name(cluster=w841, "Lockin"=w836) -> (w842:T41)
        n407 = call <vilib>:"Add State(s) to Queue__jki_lib_state_machine.vi"("State(s) in (\"\")"=w845) -> ("States Out"=w844:string)  [unwired: 14 in]
      }
      frame "UI: Initialize Gains" {
        n408 = Unbundle By Name(w861) -> ("Lockin"=w860:refnum<class "Instrument.Lockin.lvclass">)
        n409 = call "Initialize Input Gain.vi"("error in (no error)"=w859, "Instrument.Lockin"=w860) -> ("error out"=w857:errorcluster, "Input Gain"=w855:cluster{string, "Gain":dbl}[], "Instrument.Lockin out"=w858:refnum<class "Instrument.Lockin.lvclass">)  [unwired: 7 in]
        n410 = property on="Input Gain" class="Arr (strict)"(error in=w857, "Val(Sgnl)"=w855) -> (error out=w856:errorcluster)  [unwired: 1 in, 1 out]
        n411 = call "Initialize Ouput Gain.vi"("error in (no error)"=w856, "Instrument.Lockin"=w858) -> ("error out"=w852:errorcluster, "Ouput Gain"=w854:cluster{string, "Gain":dbl}[], "Instrument.Lockin out"=w853:refnum<class "Instrument.Lockin.lvclass">)  [unwired: 7 in]
        n412 = property on="Output Gain" class="Arr (strict)"(error in=w852, "Val(Sgnl)"=w854) -> (error out=w851:errorcluster)  [unwired: 1 in, 1 out]
        n413 = Bundle By Name(cluster=w861, "Lockin"=w853) -> (w862:T41)
        n414 = call <vilib>:"Add State(s) to Queue__jki_lib_state_machine.vi"("State(s) in (\"\")"=w865) -> ("States Out"=w864:string)  [unwired: 14 in]
      }
      frame "UI: Update Rings" {
        # "update Sweep Channel ring"
        n415 = Unbundle By Name(w879) -> ("Lockin"=w878:refnum<class "Instrument.Lockin.lvclass">)
        n416 = disable-structure shown="Enabled" {
          frame Disabled {
            n417 = call "Get AI REF (f) StringsAndValues.vi"() -> ("error out"=w886:errorcluster, "AI REF (f) StringsAndValues"=w885:cluster{string, i32}[], "Instrument.Lockin out"=w884:refnum<class "Instrument.Lockin.lvclass">)  [unwired: 9 in]
            n418 = property on="Channel" class="Ring (strict)"(error in=w886, "StringsAndValues[]"=w885) -> ()  [unwired: 1 in, 2 out]
          }
          frame Enabled {
          }
        }
        n419 = call "Get AO StringsAndValues.vi"("error in (no error)"=w877, "Instrument.Lockin in"=w878) -> ("error out"=w875:errorcluster, "AO Strings and Values"=w876:cluster{string, i32}[], "Instrument.Lockin out"=w873:refnum<class "Instrument.Lockin.lvclass">)  [unwired: 7 in]
        n420 = property on="Channel" class="Ring (strict)"(error in=w875, "StringsAndValues[]"=w876) -> (error out=w872:errorcluster)  [unwired: 1 in, 1 out]
        n421 = call "Get REF StringsAndValues.vi"("error in (no error)"=w872, "Instrument.Lockin in"=w873) -> ("error out"=w874:errorcluster, "REF Strings and Values"=w871:cluster{string, i32}[], "Instrument.Lockin out"=w870:refnum<class "Instrument.Lockin.lvclass">)  [unwired: 7 in]
        n422 = property on="Reference" class="Ring (strict)"(error in=w874, "StringsAndValues[]"=w871) -> (error out=w868:errorcluster)  [unwired: 1 in, 1 out]
        n423 = call "Remote Unused References.vi"("error in (no error)"=w868, "Instrument.Lockin in"=w870) -> ("error out"=w867:errorcluster, "Array"=w866:T2[], "Instrument.Lockin out"=w869:refnum<class "Instrument.Lockin.lvclass">)  [unwired: 7 in]
        n424 = Bundle By Name(cluster=w879, "Lockin"=w869) -> (w880:T41)
        n425 = local write "AI Channels"(w866) -> ()
        n426 = call <vilib>:"Add State(s) to Queue__jki_lib_state_machine.vi"("State(s) in (\"\")"=w883) -> ("States Out"=w882:string)  [unwired: 14 in]
      }
      frame "UI: Update Plot Names" {
        n427 = Unbundle By Name(w890) -> ("Lockin"=w895:refnum<class "Instrument.Lockin.lvclass">)
        n428 = Equal?(x=w897, y="Reset") -> ()  [unwired: 1 out]
        n429 = call "Get AO StringsAndValues.vi"("error in (no error)"=w887, "Instrument.Lockin in"=w895) -> ("error out"=w899:errorcluster, "AO Strings and Values"=w892:cluster{string, i32}[])  [unwired: 7 in, 1 out]
        n430 = call "Get AI StringsAndValues.vi"("error in (no error)"=w887, "Instrument.Lockin in"=w895) -> ("error out"=w900:errorcluster, "AI StringsAndValues"=w901:cluster{string, i32}[])  [unwired: 7 in, 1 out]
        n431 = call "Get AI REF StringsAndValues.vi"("error in (no error)"=w887, "Instrument.Lockin in"=w895) -> ("error out"=w888:errorcluster, "REF StringsAndValues"=w889:cluster{string, i32}[])  [unwired: 7 in, 1 out]
        n432 = for {
          tunnel: w892 -> [w918] mode=indexing
          tunnel: w899 -> [w919]
          tunnel: [w916] -> w898
          i -> [w920]
          n433 = control-ref of="Sweep Results AO"() -> (w917:refnum<vi>)
          n434 = Unbundle(w918) -> (w921:string)  [unwired: 1 out]
          n435 = call "Legend - WaveformGraph.vi"("error in (no error)"=w919, "Plot.Plot Name"=w921, "Active Plot"=w920, "WFGraph in"=w917) -> ("error out"=w916:errorcluster)  [unwired: 4 in, 3 out]
        }
        n436 = for {
          tunnel: w901 -> [w931] mode=indexing
          tunnel: w900 -> [w932]
          tunnel: [w924] -> w903
          i -> [w933]
          n437 = control-ref of="AI Graph"() -> (w934:refnum<vi>)
          n438 = Unbundle(w931) -> (w935:string)  [unwired: 1 out]
          n439 = control-ref of="Sweep Results AI"() -> (w927:refnum<vi>)
          n440 = call "Legend - WaveformGraph.vi"("error in (no error)"=w932, "Plot.Plot Name"=w935, "Active Plot"=w933, "WFGraph in"=w934) -> ("error out"=w930:errorcluster, "Plot.Plot Name"=w929:string, "Active Plot"=w928:i32)  [unwired: 4 in, 1 out]
          n441 = call "Legend - WaveformGraph.vi"("error in (no error)"=w930, "Plot.Plot Name"=w929, "Active Plot"=w928, "WFGraph in"=w927) -> ("error out"=w926:errorcluster, "Plot.Plot Name"=w923:string, "Active Plot"=w922:i32)  [unwired: 4 in, 1 out]
          n442 = control-ref of="PS WFGraph"() -> (w925:refnum<vi>)
          n443 = call "Legend - WDTWaveformGraph.vi"("error in (no error)"=w926, "Plot.Plot Name"=w923, "Active Plot"=w922, "WFGraph (WDT) in"=w925) -> ("error out"=w924:errorcluster)  [unwired: 4 in, 3 out]
        }
        n444 = local read "Y Axis (Output)"() -> (w891:enum16{"Analog Output", "Reference"})
        n445 = case shown="\"Analog Output\", Default" w891 {
          tunnel: [w907 w909] -> w894
          tunnel: w889 -> [_ w908]
          tunnel: w892 -> [w907 _]
          frame "Analog Output", Default {
          }
          frame "Reference" {
            n446 = Interleave 1D Arrays(w908, w908) -> (w909:cluster{string, i32}[])
          }
        }
        n447 = for {
          tunnel: w894 -> [w914] mode=indexing
          tunnel: w888 -> [w912]
          tunnel: [w911] -> w893
          i -> [w913]
          n448 = Unbundle(w914) -> (w910:string)  [unwired: 1 out]
          n449 = control-ref of="AO Graph"() -> (w915:refnum<vi>)
          n450 = call "Legend - WaveformGraph.vi"("error in (no error)"=w912, "Plot.Plot Name"=w910, "Active Plot"=w913, "WFGraph in"=w915) -> ("error out"=w911:errorcluster)  [unwired: 4 in, 3 out]
        }
        n451 = call <vilib>:"Add State(s) to Queue__jki_lib_state_machine.vi"("State(s) in (\"\")"=w906) -> ("States Out"=w905:string)  [unwired: 14 in]
        n452 = Merge Errors(w898, w903, w893, w887) -> (w902:errorcluster)
      }
      frame "UI: Sync Lockin Plot Visibility" {
        # "#todo\nshould be owned by Lockin UI"
        # "#todo\nshould be owned by Lockin UI"
        # "Do not put any code in this frame.\n(It is a separator no-op. You can make a copy of this frame to create a new UI frame)"
        n453 = local read "Results Plot Names"() -> (w938:string[])
        n454 = Array Size(array=w938) -> (size(s)=w939:i32)
        n455 = feedback #1() -> (w941:string[])  [unwired: 1 in]
        n456 = feedback-in #1(w938) -> ()
        n457 = Not Equal?(x=w941, y=w938) -> (x != y?=w943:bool)
        n458 = First Call?() -> (First Call?: T/F=w944:bool)
        n459 = Or(x=w944, y=w943) -> (x .or. y?=w942:bool)
        n460 = case shown="True" w942 {
          tunnel: w937 -> [w966 w970]
          tunnel: w938 -> [_ w971]
          tunnel: [w966 w967] -> w940
          frame False {
          }
          frame True {
            n461 = for {
              tunnel: w970 -> [w992]
              tunnel: [w977] -> w968
              tunnel: w971 -> [w972] mode=indexing
              i -> [w987]
              n462 = control-ref of="XY Graph"() -> (w982:refnum<vi>)
              n463 = control-ref of="Lockin 2"() -> (w983:refnum<vi>)
              n464 = control-ref of="Lockin 1"() -> (w984:refnum<vi>)
              n465 = call "Legend - WaveformChart.vi"("error in (no error)"=w992, "Plot.Plot Name"=w972, "Active Plot"=w987, "WaveformChart in"=w984) -> ("error out"=w988:errorcluster, "Plot.Plot Name"=w986:string, "Active Plot"=w991:i32)  [unwired: 4 in, 1 out]
              n466 = control-ref of="Sweep Results Y"() -> (w980:refnum<vi>)
              n467 = control-ref of="Sweep Results X"() -> (w981:refnum<vi>)
              n468 = call "Legend - WaveformChart.vi"("error in (no error)"=w988, "Plot.Plot Name"=w986, "Active Plot"=w991, "WaveformChart in"=w983) -> ("error out"=w989:errorcluster, "Plot.Plot Name"=w985:string, "Active Plot"=w990:i32)  [unwired: 4 in, 1 out]
              n469 = call "Legend - XYGraph.vi"("error in (no error)"=w989, "Plot.Plot Name"=w985, "Active Plot"=w990, "XYGraph in"=w982) -> ("error out"=w979:errorcluster, "Plot.Plot Name"=w973:string, "Active Plot"=w976:i32)  [unwired: 4 in, 1 out]
              n470 = call "Legend - WaveformGraph.vi"("error in (no error)"=w979, "Plot.Plot Name"=w973, "Active Plot"=w976, "WFGraph in"=w981) -> ("error out"=w978:errorcluster, "Plot.Plot Name"=w974:string, "Active Plot"=w975:i32)  [unwired: 4 in, 1 out]
              n471 = call "Legend - WaveformGraph.vi"("error in (no error)"=w978, "Plot.Plot Name"=w974, "Active Plot"=w975, "WFGraph in"=w980) -> ("error out"=w977:errorcluster)  [unwired: 4 in, 3 out]
            }
            n472 = property on="Channel" class="Ring (strict)"(error in=w970, "Strings []"=w971) -> (error out=w969:errorcluster)  [unwired: 1 in, 1 out]
            n473 = Merge Errors(w969, w968) -> (w967:errorcluster)
          }
        }
        n474 = for {
          N: w939 -> [_]
          tunnel: w940 -> [w955]
          tunnel: [w950] -> w936
          i -> [w964]
          n475 = control-ref of="Lockin 1"() -> (w965:refnum<vi>)
          n476 = call "Get Plot Visibility - WaveformChart.vi"("error in (no error)"=w955, "ActPlot"=w964, "WaveformChart in"=w965) -> ("error out"=w954:errorcluster, "Plot.Visible?"=w949:bool, "Active Plot"=w959:i32)  [unwired: 6 in]
          n477 = control-ref of="Lockin 2"() -> (w963:refnum<vi>)
          n478 = call "Set Plot Visibility - WaveformChart.vi"("error in (no error)"=w954, "Plot.Visible?"=w949, "ActPlot"=w959, "WaveformChart in"=w963) -> ("error out"=w953:errorcluster, "Active Plot"=w958:i32)  [unwired: 6 in]
          n479 = control-ref of="XY Graph"() -> (w962:refnum<vi>)
          n480 = call "Set Plot Visibility - XYGraph.vi"("error in (no error)"=w953, "Plot.Visible?"=w949, "ActPlot"=w958, "XYGraph in"=w962) -> ("error out"=w952:errorcluster, "Active Plot"=w957:i32)  [unwired: 6 in]
          n481 = control-ref of="Sweep Results Y"() -> (w961:refnum<vi>)
          n482 = control-ref of="Sweep Results X"() -> (w960:refnum<vi>)
          n483 = call "Set Plot Visibility - WaveformGraph.vi"("error in (no error)"=w952, "Plot.Visible?"=w949, "ActPlot"=w957, "WFGraph in"=w961) -> ("error out"=w951:errorcluster, "Active Plot"=w956:i32)  [unwired: 6 in]
          n484 = call "Set Plot Visibility - WaveformGraph.vi"("error in (no error)"=w951, "Plot.Visible?"=w949, "ActPlot"=w956, "WFGraph in"=w960) -> ("error out"=w950:errorcluster)  [unwired: 6 in, 1 out]
        }
        n485 = call <vilib>:"Add State(s) to Queue__jki_lib_state_machine.vi"("State(s) in (\"\")"=w948) -> ("States Out"=w947:string)  [unwired: 14 in]
      }
      frame "UI: Sync AO AI Plot Visibility" {
        # "Do not put any code in this frame.\n(It is a separator no-op. You can make a copy of this frame to create a new UI frame)"
        n486 = Unbundle By Name(w999) -> ("Lockin"=w997:refnum<class "Instrument.Lockin.lvclass">)
        n487 = call "Get AO StringsAndValues.vi"("error in (no error)"=w995, "Instrument.Lockin in"=w997) -> ("error out"=w993:errorcluster, "AO Strings and Values"=w996:cluster{string, i32}[])  [unwired: 7 in, 1 out]
        n488 = call "Get AI StringsAndValues.vi"("error in (no error)"=w995, "Instrument.Lockin in"=w997) -> ("error out"=w994:errorcluster, "AI StringsAndValues"=w998:cluster{string, i32}[])  [unwired: 7 in, 1 out]
        n489 = for {
          tunnel: w994 -> [w1019]
          tunnel: [w1015] -> w1001
          tunnel: w998 -> [_] mode=indexing
          i -> [w1022]
          n490 = control-ref of="AI Graph"() -> (w1018:refnum<vi>)
          n491 = property on="Property Node" class="WFGraph (strict)"(reference=w1018, error in=w1019, "Active Plot"=w1022) -> (error out=w1023:errorcluster, "Plot.Visible?"=w1021:bool)  [unwired: 1 out]
          n492 = control-ref of="Sweep Results AI"() -> (w1020:refnum<vi>)
          n493 = property on="Property Node" class="WFGraph (strict)"(reference=w1020, error in=w1023, "Active Plot"=w1022, "Plot.Visible?"=w1021) -> (error out=w1016:errorcluster)  [unwired: 1 out]
          n494 = call <vilib>:"Clear Errors.vi"("error in (no error)"=w1016, "specific error code to clear (0: all)"=1077) -> ("error out"=w1015:errorcluster)  [unwired: 4 in, 1 out]
        }
        n495 = for {
          tunnel: w993 -> [w1009]
          tunnel: [w1006] -> w1002
          tunnel: w996 -> [_] mode=indexing
          i -> [w1013]
          n496 = control-ref of="AO Graph"() -> (w1010:refnum<vi>)
          n497 = property on="Property Node" class="WFGraph (strict)"(reference=w1010, error in=w1009, "Active Plot"=w1013) -> (error out=w1014:errorcluster, "Plot.Visible?"=w1012:bool)  [unwired: 1 out]
          n498 = control-ref of="Sweep Results AO"() -> (w1011:refnum<vi>)
          n499 = property on="Property Node" class="WFGraph (strict)"(reference=w1011, error in=w1014, "Active Plot"=w1013, "Plot.Visible?"=w1012) -> (error out=w1007:errorcluster)  [unwired: 1 out]
          n500 = call <vilib>:"Clear Errors.vi"("error in (no error)"=w1007, "specific error code to clear (0: all)"=1077) -> ("error out"=w1006:errorcluster)  [unwired: 4 in, 1 out]
        }
        n501 = Merge Errors(w1001, w1002) -> (w1000:errorcluster)
        n502 = call <vilib>:"Add State(s) to Queue__jki_lib_state_machine.vi"("State(s) in (\"\")"=w1005) -> ("States Out"=w1004:string)  [unwired: 14 in]
      }
      frame "UI: Disable Buttons" {
        n503 = control-ref of="Start"() -> (w1029:refnum<vi>)
        n504 = control-ref of="Pause"() -> (w1028:refnum<vi>)
        n505 = control-ref of="Trigger"() -> (w1027:refnum<vi>)
        n506 = control-ref of="Reset"() -> (w1026:refnum<vi>)
        n507 = control-ref of="Help"() -> (w1025:refnum<vi>)
        n508 = Build Array(w1029, w1028, w1027, w1026, w1025) -> (w1024:refnum<vi>[])
        n509 = for {
          tunnel: w1024 -> [w1036] mode=indexing
          n510 = property class="Bool (strict)"(reference=w1036, "DisabledEnum"=T25."Disabled and Grayed Out" ("Disabled")) -> ()  [unwired: 1 in, 2 out]
        }
        n511 = call <vilib>:"Add State(s) to Queue__jki_lib_state_machine.vi"("State(s) in (\"\")"=w1034) -> ("States Out"=w1033:string)  [unwired: 14 in]
      }
      frame "UI: Enable Buttons" {
        n512 = control-ref of="Start"() -> (w1042:refnum<vi>)
        n513 = control-ref of="Pause"() -> (w1041:refnum<vi>)
        n514 = control-ref of="Trigger"() -> (w1040:refnum<vi>)
        n515 = control-ref of="Reset"() -> (w1039:refnum<vi>)
        n516 = control-ref of="Help"() -> (w1038:refnum<vi>)
        n517 = Build Array(w1042, w1041, w1040, w1039, w1038) -> (w1037:refnum<vi>[])
        n518 = for {
          tunnel: w1037 -> [w1049] mode=indexing
          n519 = property class="Bool (strict)"(reference=w1049, "DisabledEnum"=T25."Enabled" ("Disabled")) -> ()  [unwired: 1 in, 2 out]
        }
        n520 = call <vilib>:"Add State(s) to Queue__jki_lib_state_machine.vi"("State(s) in (\"\")"=w1047) -> ("States Out"=w1046:string)  [unwired: 14 in]
      }
      frame "UI: AI Graph Plot Visible" {
        # "Do not put any code in this frame.\n(It is a separator no-op. You can make a copy of this frame to create a new UI frame)"
        n521 = case shown="\"ALL\"" w1055 {
          tunnel: [FALSE TRUE] -> w1052
          frame "None", Default {
          }
          frame "ALL" {
          }
        }
        n522 = control-ref of="AI Graph"() -> (w1056:refnum<vi>)
        n523 = control-ref of="Sweep Results AI"() -> (w1053:refnum<vi>)
        n524 = call "Plots Visible - All or None - WaveformGraph.vi"("error in (no error)"=w1054, "All Visible?"=w1052, "WFGraph in"=w1056) -> ("error out"=w1051:errorcluster)  [unwired: 7 in, 1 out]
        n525 = call "Plots Visible - All or None - WaveformGraph.vi"("error in (no error)"=w1051, "All Visible?"=w1052, "WFGraph in"=w1053) -> ("error out"=w1050:errorcluster)  [unwired: 7 in, 1 out]
        n526 = call <vilib>:"Add State(s) to Queue__jki_lib_state_machine.vi"("State(s) in (\"\")"=w1060) -> ("States Out"=w1059:string)  [unwired: 14 in]
      }
      frame "UI: AO Graph Plot Visible" {
        # "Do not put any code in this frame.\n(It is a separator no-op. You can make a copy of this frame to create a new UI frame)"
        n527 = case shown="\"ALL\"" w1069 {
          tunnel: [FALSE TRUE] -> w1065
          frame "None", Default {
          }
          frame "ALL" {
          }
        }
        n528 = control-ref of="AO Graph"() -> (w1067:refnum<vi>)
        n529 = call "Plots Visible - All or None - WaveformGraph.vi"("error in (no error)"=w1068, "All Visible?"=w1065, "WFGraph in"=w1067) -> ("error out"=w1064:errorcluster)  [unwired: 7 in, 1 out]
        n530 = control-ref of="Sweep Results AO"() -> (w1066:refnum<vi>)
        n531 = call "Plots Visible - All or None - WaveformGraph.vi"("error in (no error)"=w1064, "All Visible?"=w1065, "WFGraph in"=w1066) -> ("error out"=w1063:errorcluster)  [unwired: 7 in, 1 out]
        n532 = call <vilib>:"Add State(s) to Queue__jki_lib_state_machine.vi"("State(s) in (\"\")"=w1073) -> ("States Out"=w1072:string)  [unwired: 14 in]
      }
      frame "UI: Lockin 1 Plot Visible" {
        # "#todo\nshould be owned by Lockin UI"
        # "#todo\nshould be owned by Lockin UI"
        # "#todo\nshould be owned by Lockin UI"
        # "Do not put any code in this frame.\n(It is a separator no-op. You can make a copy of this frame to create a new UI frame)"
        n533 = case shown="\"ALL\"" w1088 {
          tunnel: [FALSE TRUE] -> w1084
          frame "None", Default {
          }
          frame "ALL" {
          }
        }
        n534 = control-ref of="Lockin 1"() -> (w1087:refnum<vi>)
        n535 = control-ref of="Lockin 2"() -> (w1085:refnum<vi>)
        n536 = control-ref of="Sweep Results X"() -> (w1083:refnum<vi>)
        n537 = control-ref of="Sweep Results Y"() -> (w1082:refnum<vi>)
        n538 = call "Plots Visible - All or None - WaveformChart.vi"("error in (no error)"=w1086, "All Visible?"=w1084, "WaveformChart in"=w1087) -> ("error out"=w1080:errorcluster)  [unwired: 7 in, 1 out]
        n539 = call "Plots Visible - All or None - WaveformChart.vi"("error in (no error)"=w1080, "All Visible?"=w1084, "WaveformChart in"=w1085) -> ("error out"=w1079:errorcluster)  [unwired: 7 in, 1 out]
        n540 = call "Plots Visible - All or None - WaveformGraph.vi"("error in (no error)"=w1079, "All Visible?"=w1084, "WFGraph in"=w1083) -> ("error out"=w1078:errorcluster)  [unwired: 7 in, 1 out]
        n541 = control-ref of="XY Graph"() -> (w1081:refnum<vi>)
        n542 = call "Plots Visible - All or None - WaveformGraph.vi"("error in (no error)"=w1078, "All Visible?"=w1084, "WFGraph in"=w1082) -> ("error out"=w1077:errorcluster)  [unwired: 7 in, 1 out]
        n543 = call "Plots Visible - All or None - XYGraph.vi"("error in (no error)"=w1077, "All Visible?"=w1084, "XYGraph in"=w1081) -> ("error out"=w1076:errorcluster)  [unwired: 7 in, 1 out]
        n544 = call <vilib>:"Add State(s) to Queue__jki_lib_state_machine.vi"("State(s) in (\"\")"=w1092) -> ("States Out"=w1091:string)  [unwired: 14 in]
      }
      frame "UI: Update Waveform Graphs" {
        # "#todo\nshould be owned by Lockin UI"
        # "private"
        # "private"
        n545 = Unbundle By Name(w1111) -> ("Lockin"=w1102:refnum<class "Instrument.Lockin.lvclass">)
        n546 = Unbundle By Name(w1102) -> ("Input Gain"=w1098:dbl[], "AI WFM"=w1114:waveform(dbl)[], "AO WFM"=w1105:waveform(dbl)[], "REF WFM"=w1104:waveform(dbl)[])
        n547 = local read "Y Axis (Output)"() -> (w1095:enum16{"Analog Output", "Reference"})
        n548 = case shown="\"Analog Output\", Default" w1095 {
          tunnel: w1105 -> [w1122 _]
          tunnel: w1104 -> [_ w1123]
          tunnel: [w1122 w1123] -> w1103
          frame "Analog Output", Default {
          }
          frame "Reference" {
          }
        }
        n549 = local read "X Axis"() -> (w1100:enum16{"Time", "Samples"})
        n550 = Power Of 10(x="Decimate") -> (10^x=w1106:dbl)
        n551 = call "Display n or dt.vi"("error in (no error)"=w1101, "X Axis"=w1100, "Input Waveforms"=w1114) -> ("error out"=w1113:errorcluster, "Output Waveforms"=w1099:waveform(dbl)[])  [unwired: 7 in]
        n552 = call "Display n or dt.vi"("error in (no error)"=w1101, "X Axis"=w1100, "Input Waveforms"=w1103) -> ("error out"=w1112:errorcluster, "Output Waveforms"=w1117:waveform(dbl)[])  [unwired: 7 in]
        n553 = call "decimate_waveforms.vi"("WFM"=w1117, "averaging"=FALSE, "decimating factor"=w1106, "error in (no error)"=w1112) -> ("WFM out"=→"AO Graph":waveform(dbl)[])  [unwired: 5 in, 1 out]
        n554 = call "decimate_waveforms.vi"("WFM"=w1099, "averaging"=FALSE, "decimating factor"=w1106, "error in (no error)"=w1113) -> ("WFM out"=w1110:waveform(dbl)[], "error out"=w1108:errorcluster)  [unwired: 5 in]
        n555 = case shown="\"ADC\"" "Y Axis (Input)" {
          tunnel: w1110 -> [w1125 w1130]
          tunnel: w1098 -> [_ w1128]
          tunnel: [w1125 w1129] -> w1109
          tunnel: w1108 -> [w1124 w1127]
          tunnel: [w1124 w1126] -> w1097
          frame "Device", Default {
          }
          frame "ADC" {
            n556 = call "Multiply by Gain.vi"("error in (no error)"=w1127, "Gain"=w1128, "WFM in"=w1130) -> ("error out"=w1126:errorcluster, "WFM out"=w1129:waveform(dbl)[])  [unwired: 7 in]
          }
        }
        "AI Graph" <- w1109
        n557 = call <vilib>:"Add State(s) to Queue__jki_lib_state_machine.vi"("State(s) in (\"\")"=w1121) -> ("States Out"=w1120:string)  [unwired: 14 in]
      }
      frame "UI: Update Lockin Graphs" {
        # "#todo\nshould be owned by Lockin UI"
        # "#todo\nshould be owned by Lockin UI"
        # "#todo\nshould be owned by Lockin UI"
        n558 = Unbundle By Name(w1148) -> ("Lockin"=w1138:refnum<class "Instrument.Lockin.lvclass">)
        n559 = call "Parse Results (table).vi"("error in (no error)"=w1143, "Instrument.Lockin"=w1138) -> ("error out"=w1142:errorcluster, "Table Control"=→"Results":string[][], "Results (Dictionary)"=w1137:cluster{"key":string, "value":dbl}[])  [unwired: 6 in, 1 out]
        n560 = call "Dictionary to Chart.vi"("error in (no error)"=w1142, "Display"="Display", "Results.Results (Dictionary)"=w1137) -> ("error out"=w1144:errorcluster, "XY Graph"=→"XY Graph":cluster{dbl[], dbl[]}[], "Y/Theta Array"=→"Lockin 2":waveform(dbl)[], "X/R Array"=→"Lockin 1":waveform(dbl)[], "Plot Names"=→"Results Plot Names":string[])  [unwired: 4 in]
        n561 = call "Dictionary to Indicator.vi"("Results.Results (Dictionary)"=w1137, "AI Channel"="Channel", "error in (no error)"=w1144) -> ("X"=→"X":dbl, "Y"=→"Y":dbl, "R"=→"R":dbl, "Theta"=→"Theta":dbl, "error out"=w1136:errorcluster)  [unwired: 8 in]
        n562 = call <vilib>:"Add State(s) to Queue__jki_lib_state_machine.vi"("State(s) in (\"\")"=w1151) -> ("States Out"=w1150:string)  [unwired: 14 in]
      }
      frame "UI: Update Waveform Graph Labels" {
        n563 = control-ref of="AI Graph"() -> (w1160:refnum<vi>)
        n564 = control-ref of="AO Graph"() -> (w1155:refnum<vi>)
        n565 = call "X Axis WFM Graph.vi"("error in (no error)"=w1156, "X Axis"="X Axis", "WaveformGraph in"=w1160) -> ("error out"=w1158:errorcluster)  [unwired: 8 in]
        n566 = call "X Axis WFM Graph.vi"("error in (no error)"=w1158, "X Axis"="X Axis", "WaveformGraph in"=w1155) -> ("error out"=w1157:errorcluster)  [unwired: 8 in]
        n567 = control-ref of="AO Graph"() -> (w1154:refnum<vi>)
        n568 = call "Y Axis Output WFM Graph.vi"("error in (no error)"=w1157, "Y Axis Out"="Y Axis (Output)", "WaveformGraph in"=w1154) -> ("error out"=w1153:errorcluster)  [unwired: 8 in]
        n569 = call <vilib>:"Add State(s) to Queue__jki_lib_state_machine.vi"("State(s) in (\"\")"=w1164) -> ("States Out"=w1163:string)  [unwired: 14 in]
      }
      frame "UI: Update Lockin Graph Range" {
        n570 = Negate(x="Numeric") -> (-x=w1167:dbl)
        n571 = Negate(x="X/R Range") -> (-x=w1169:dbl)
        n572 = Negate(x="Y/Theta Range") -> (-x=w1170:dbl)
        n573 = property on="Lockin 1" class="WFChart (strict)"("YScale.Maximum"="X/R Range", "YScale.Minimum"=w1169) -> ()  [unwired: 2 in, 2 out]
        n574 = property on="Lockin 2" class="WFChart (strict)"("YScale.Maximum"="Y/Theta Range", "YScale.Minimum"=w1170) -> ()  [unwired: 2 in, 2 out]
        n575 = property on="XY Graph" class="XYGraph (strict)"("XScale.Maximum"="Numeric", "XScale.Minimum"=w1167, "YScale.Maximum"="Numeric", "YScale.Minimum"=w1167) -> ()  [unwired: 2 in, 2 out]
        n576 = call <vilib>:"Add State(s) to Queue__jki_lib_state_machine.vi"("State(s) in (\"\")"=w1175) -> ("States Out"=w1174:string)  [unwired: 14 in]
      }
      frame "UI: Update Displays" {
        n577 = local read "Display"() -> (w1178:T19)
        n578 = case shown="\"X and Y\", Default" w1178 {
          tunnel: ["X (V)" "R (V)"] -> _
          tunnel: ["Y (V)" "Theta (°)"] -> _
          tunnel: ["Lockin X (V)" "R (V)"] -> w1177
          tunnel: ["Lockin Y (V)" "Theta (°)"] -> w1176
          frame "X and Y", Default {
          }
          frame "R and Theta" {
          }
        }
        n579 = property on="Lockin 1" class="WFChart (strict)"("YScale.NameLbl.Text"=w1177) -> ()  [unwired: 2 in, 2 out]
        n580 = property on="Lockin 2" class="WFChart (strict)"("YScale.NameLbl.Text"=w1176) -> ()  [unwired: 2 in, 2 out]
        n581 = call <vilib>:"Add State(s) to Queue__jki_lib_state_machine.vi"("State(s) in (\"\")"=w1183) -> ("States Out"=w1182:string)  [unwired: 14 in]
      }
      frame "UI: Update Sweep Results Graphs" {
        n582 = Unbundle By Name(w1194) -> ("SweepResults.X results"=→"Sweep Results X":waveform(dbl)[], "SweepResults.Y Results"=→"Sweep Results Y":waveform(dbl)[])
        n583 = call <vilib>:"Add State(s) to Queue__jki_lib_state_machine.vi"("State(s) in (\"\")"=w1198) -> ("States Out"=w1197:string)  [unwired: 14 in]
      }
      frame "UI: Update Sweep WFMs Graphs" {
        n584 = Unbundle By Name(w1201) -> ("SweepWaveforms.Sweep_AO"=→"Sweep Results AO":waveform(dbl)[], "SweepWaveforms.Sweep_AI"=→"Sweep Results AI":waveform(dbl)[])
        n585 = call <vilib>:"Add State(s) to Queue__jki_lib_state_machine.vi"("State(s) in (\"\")"=w1205) -> ("States Out"=w1204:string)  [unwired: 14 in]
      }
      frame "UI: Update Status" {
        n586 = Unbundle By Name(w1208) -> ("Lockin"=w1207:refnum<class "Instrument.Lockin.lvclass">)
        n587 = Unbundle By Name(w1207) -> ("state"=w1206:T35)
        n588 = case shown="\"started\"" w1206 {
          tunnel: ["Idle" ("Status") "Started" ("Status") "Stopped" ("Status") "Running" ("Status") "Sweeping" ("Status")] -> w1209
          frame "idle", Default {
            w1215 = FALSE ("Trigger")
            n589 = local write "Reset"(w1215) -> ()
            n590 = local write "Trigger"(w1215) -> ()
            n591 = local write "Start"(w1215) -> ()
          }
          frame "started" {
            w1216 = FALSE ("Trigger")
            n592 = local write "Start Sweep"(w1216) -> ()
            n593 = local write "Reset"(w1216) -> ()
            n594 = local write "Stop Sweep"(w1216) -> ()
            n595 = disable-structure shown="Disabled" {
              frame Disabled {
                n596 = local read "Trigger"() -> ()  [unwired: 1 in]
              }
              frame Enabled {
              }
            }
            n597 = local write "Start"(TRUE ("Trigger")) -> ()
          }
          frame "stopped" {
            w1221 = FALSE ("Trigger")
            n598 = local write "Reset"(w1221) -> ()
            n599 = local write "Trigger"(w1221) -> ()
            n600 = local write "Start"(FALSE ("Trigger")) -> ()
          }
          frame "created" {
            n601 = local write "Start"(TRUE ("Start")) -> ()
            n602 = local write "Reset"(FALSE ("Reset")) -> ()
          }
          frame "sweeping" {
            n603 = call <userlib>:"MGI Milliseconds Since Last Reset.vi"("Reset (F)"=TRUE) -> ()  [unwired: 5 in, 2 out]
          }
        }
        n604 = local write "Status"(w1209) -> ()
        n605 = call <vilib>:"Add State(s) to Queue__jki_lib_state_machine.vi"("State(s) in (\"\")"=w1213) -> ("States Out"=w1212:string)  [unwired: 14 in]
      }
      frame "UI: Update Sweep Timer" {
        n606 = local read "Status"() -> (w1228:string)
        n607 = case shown="\"Sweeping\"" w1228 {
          tunnel: [0.0 w1236] -> w1227
          frame Default {
          }
          frame "Sweeping" {
            # "some overhead"
            n608 = call <userlib>:"MGI Milliseconds Since Last Reset.vi"() -> ("ms"=w1242:u32)  [unwired: 6 in, 1 out]
            n609 = local read "Sweep Time (s)"() -> (w1238:dbl)
            n610 = local read "Initial Wait (s)"() -> (w1239:dbl)
            n611 = Divide(x=w1242, y=u32 1000) -> (x/y=w1240:dbl)
            n612 = Negate(x=w1240) -> (-x=w1237:dbl)
            n613 = Compound Arithmetic op=ADD(2.0 ("value"), w1239, w1238, w1237) -> (w1236:dbl)
          }
        }
        "Sweep Timer (s)" <- w1227
        n614 = call <vilib>:"Add State(s) to Queue__jki_lib_state_machine.vi"("State(s) in (\"\")"=w1233) -> ("States Out"=w1232:string)  [unwired: 14 in]
      }
      frame "UI: Defer Panel Updates" {
        n615 = case shown="\"True\"" w1244 {
          tunnel: [FALSE ("Defer Updates?") TRUE ("Defer Updates?")] -> w1243
          frame "False", Default {
          }
          frame "True" {
          }
        }
        n616 = call <userlib>:"MGI Defer Panel Updates.vi"("Error In"=w1246, "Defer Updates?"=w1243) -> ("Error Out"=w1245:errorcluster)  [unwired: 9 in]
        n617 = call <vilib>:"Add State(s) to Queue__jki_lib_state_machine.vi"("State(s) in (\"\")"=w1250) -> ("States Out"=w1249:string)  [unwired: 14 in]
      }
      frame "UI: Cursor Set" {
        # "Argument"
        # "Set and Unset Cursor Busy.\n(Usage: \"UI: Cursor Set >> Busy|Idle\")"
        n618 = case shown="\"Busy\"" w1257 {
          tunnel: w1254 -> [w1261 w1263]
          tunnel: [w1260 w1262] -> w1253
          frame "Idle", Default {
            n619 = call <vilib>:"Unset Busy.vi"("error in (no error)"=w1261) -> ("error out"=w1260:errorcluster)  [unwired: 10 in]
          }
          frame "Busy" {
            n620 = call <vilib>:"Set Busy.vi"("error in (no error)"=w1263) -> ("error out"=w1262:errorcluster)  [unwired: 9 in, 1 out]
          }
        }
        n621 = call <vilib>:"Add State(s) to Queue__jki_lib_state_machine.vi"("State(s) in (\"\")"=w1259) -> ("States Out"=w1258:string)  [unwired: 14 in]
      }
      frame "UI: Front Panel State" {
        # "Argument"
        n622 = Unbundle By Name(w1266) -> ("Core.Current VI Reference"=w1268:refnum<vi>)
        n623 = case shown="\"Open\", Default" w1267 {
          tunnel: w1269 -> [w1275 w1288]
          tunnel: [w1277 w1289] -> w1265
          tunnel: w1268 -> [w1276 w1286]
          frame "Open", Default {
            n624 = property class="VI"(reference=w1276, error in=w1275) -> (reference out=w1273:refnum<vi>, error out=w1274:errorcluster, "Front Panel.Open"=w1272:bool)
            n625 = case shown="True" w1272 {
              tunnel: [w1280 w1283] -> w1277
              tunnel: w1274 -> [w1279 w1283]
              tunnel: w1273 -> [w1278 _]
              frame False {
                n626 = invoke class="VI" method="FP.Open"(reference=w1278, error in=w1279, "Activate"=TRUE, "State"=T26."Standard") -> (error out=w1280:errorcluster)  [unwired: 1 in, 4 out]
              }
              frame True {
              }
            }
          }
          frame "Close" {
            n627 = property class="VI"(reference=w1286, error in=w1288) -> (reference out=w1285:refnum<vi>, error out=w1287:errorcluster, "Front Panel.Open"=w1284:bool)
            n628 = case shown="True" w1284 {
              tunnel: [w1290 w1293] -> w1289
              tunnel: w1287 -> [w1290 w1292]
              tunnel: w1285 -> [_ w1291]
              frame False {
              }
              frame True {
                n629 = invoke class="VI" method="FP.Close"(reference=w1291, error in=w1292) -> (error out=w1293:errorcluster)  [unwired: 1 in, 2 out]
              }
            }
          }
        }
        n630 = call <vilib>:"Add State(s) to Queue__jki_lib_state_machine.vi"("State(s) in (\"\")"=w1271) -> ("States Out"=w1270:string)  [unwired: 14 in]
      }
      frame "UI: Cleanup" {
        w1295 = FALSE ("Close")
        w1294 = waveform(dbl)[] [] ("Signals Graph")
        w1297 = waveform(dbl)[][] [] ("History Data")
        # "Initialize the User Interface, here.\n(this is called automatically, by the Macro: Exit)"
        n631 = property on="Lockin 1" class="WFChart (strict)"("History Data"=w1297) -> ()  [unwired: 2 in, 2 out]
        n632 = local write "Sweep Results X"(w1294) -> ()
        n633 = local write "Sweep Results Y"(w1294) -> ()
        n634 = property on="AI Graph" class="WFGraph (strict)"("Value"=w1294) -> (error out=w1296:errorcluster)  [unwired: 2 in, 1 out]
        n635 = property on="Lockin 2" class="WFChart (strict)"("History Data"=w1297) -> ()  [unwired: 2 in, 2 out]
        n636 = property on="AO Graph" class="WFGraph (strict)"(error in=w1296, "Value"=w1294) -> ()  [unwired: 1 in, 2 out]
        n637 = local write "Self Calibrate"(w1295) -> ()
        n638 = local write "Trigger"(w1295) -> ()
        n639 = local write "Close"(w1295) -> ()
        n640 = local write "Pause"(w1295) -> ()
        n641 = local write "Reset"(w1295) -> ()
        n642 = local write "Start"(w1295) -> ()
        n643 = local write "Status"("Shutdown" ("Status")) -> ()
        n644 = call <vilib>:"Add State(s) to Queue__jki_lib_state_machine.vi"("State(s) in (\"\")"=w1303) -> ("States Out"=w1302:string)  [unwired: 14 in]
      }
      frame "---------- Macro ----------" {
        # "Do not put any code in this frame.\n(It is a separator no-op. You can make a copy of this frame to create a new Macro frame)"
        n645 = call <vilib>:"Add State(s) to Queue__jki_lib_state_machine.vi"("State(s) in (\"\")"=w1308) -> ("States Out"=w1307:string)  [unwired: 14 in]
      }
      frame "Macro: Initialize" {
        n646 = call <vilib>:"Add State(s) to Queue__jki_lib_state_machine.vi"("State(s) in Front (\"\")"="Data: Initialize\nInitialize Core Data\n\nUI: Initialize\n\nRemote SMO: Create\nLockin SMO: Create\nEvents: Register\nRemote SMO: Start\nLockin SMO: Start\n\nError Logger: Create\n\nUI: Front Panel State >> Open\n\nConfiguration: Initialize\nConfiguration: Read\n\nMacro: Initialize UI\nUI: Update Sweep WFMs Graphs\nUI: Disable Buttons\n\nRemote SMO: AllowedRemote\n\nMacro: Initialize DAQ SMO", "State(s) in (\"\")"=w1309) -> ("States Out"=w1314:string)  [unwired: 13 in]
      }
      frame "Macro: Initialize UI" {
        w1315 = "UI: Initialize REF Ch\nUI: Initialize AO Ch\nUI: Initialize Gains\nUI: Update AI Ch\nUI: Update Plot Names\nUI: Update Waveform Graph Labels\nUI: Update Displays" ("State(s) in Front (\"\")")
        n647 = First Call?() -> (First Call?: T/F=w1316:bool)
        n648 = Select(t=w1315, s=w1316, f="UI: Update Plot Names\nUI: Update Waveform Graph Labels\nUI: Update Displays" ("State(s) in Front (\"\")")) -> ()  [unwired: 1 out]
        n649 = call <vilib>:"Add State(s) to Queue__jki_lib_state_machine.vi"("State(s) in Front (\"\")"=w1315, "State(s) in (\"\")"=w1322) -> ("States Out"=w1321:string)  [unwired: 13 in]
      }
      frame "Macro: Initialize DAQ SMO" {
        n650 = Unbundle By Name(w1324) -> ("Lockin.DAQ"=w1327:refnum<class "Lockin.DAQ.lvclass">)
        n651 = while {
          tunnel: [w1342] -> w1325
          tunnel: w1327 -> [w1341]
          tunnel: w1326 -> [w1340]
          tunnel: [w1338] -> w1323
          i -> [w1335]
          stop <- w1332 stop-if-true
          n652 = call <vilib>:"GetState.vi"("error in (no error)"=w1340, "SMO"=w1341) -> ("error out"=w1339:errorcluster, "SMO State"=w1337:T16)  [unwired: 7 in, 1 out]
          n653 = case shown="\"Started\"" w1337 {
            tunnel: ["" "Lockin SMO: Set AI Config\nLockin SMO: Set AO Config\nLockin SMO: Set AI\nLockin SMO: Set AO\nLockin SMO: Set REF\nLockin SMO: Set Input Gain\nLockin SMO: Set Output Gain\nMacro: Update Sampling\n//Lockin SMO: Set Sampling"] -> w1342
            tunnel: w1339 -> [w1344 w1347]
            tunnel: [w1343 w1347] -> w1338
            frame Default {
              n654 = call <userlib>:"Wait (ms)__ogtk.vi"("error in (no error)"=w1344, "milliseconds to wait"=u32 100) -> ("error out"=w1343:errorcluster)  [unwired: 8 in, 1 out]
            }
            frame "Started" {
              # "send all stuff to the Lockin.DAQ"
            }
          }
          n655 = Equal?(x=w1337, y=SMOState_--Enum."Started") -> (x = y?=w1333:bool)
          n656 = Greater?(x=w1335, y=10) -> (0:w1331:bool)
          n657 = Or(x=w1333, y=w1331) -> (x .or. y?=w1332:bool)
        }
        n658 = call <vilib>:"Add State(s) to Queue__jki_lib_state_machine.vi"("State(s) in Front (\"\")"=w1325, "State(s) in (\"\")"=w1330) -> ("States Out"=w1329:string)  [unwired: 13 in]
      }
      frame "Macro: Reset DAQ SMO" {
        # "same as \"Macro: Initialize DAQ SMO\""
        n659 = Unbundle By Name(w1350) -> ("Lockin.DAQ"=w1353:refnum<class "Lockin.DAQ.lvclass">)
        n660 = while {
          tunnel: [w1368] -> w1351
          tunnel: w1353 -> [w1367]
          tunnel: w1352 -> [w1366]
          tunnel: [w1364] -> w1349
          i -> [w1361]
          stop <- w1358 stop-if-true
          n661 = call <vilib>:"GetState.vi"("error in (no error)"=w1366, "SMO"=w1367) -> ("error out"=w1365:errorcluster, "SMO State"=w1363:T16)  [unwired: 7 in, 1 out]
          n662 = case shown="\"Started\"" w1363 {
            tunnel: ["" "Lockin SMO: Set AI Config\nLockin SMO: Set AO Config\nLockin SMO: Set AI\nLockin SMO: Set AO\nLockin SMO: Set REF\nLockin SMO: Set Input Gain\nLockin SMO: Set Output Gain\nMacro: Update Sampling\n//Lockin SMO: Set Sampling"] -> w1368
            tunnel: w1365 -> [w1370 w1373]
            tunnel: [w1369 w1373] -> w1364
            frame Default {
              n663 = call <userlib>:"Wait (ms)__ogtk.vi"("error in (no error)"=w1370, "milliseconds to wait"=u32 100) -> ("error out"=w1369:errorcluster)  [unwired: 8 in, 1 out]
            }
            frame "Started" {
            }
          }
          n664 = Equal?(x=w1363, y=SMOState_--Enum."Started") -> (x = y?=w1359:bool)
          n665 = Greater?(x=w1361, y=10) -> (0:w1357:bool)
          n666 = Or(x=w1359, y=w1357) -> (x .or. y?=w1358:bool)
        }
        n667 = call <vilib>:"Add State(s) to Queue__jki_lib_state_machine.vi"("State(s) in Front (\"\")"=w1351, "State(s) in (\"\")"=w1356) -> ("States Out"=w1355:string)  [unwired: 13 in]
      }
      frame "Macro: Reset RC SMO" {
        # "unused"
        n668 = call <vilib>:"Add State(s) to Queue__jki_lib_state_machine.vi"("State(s) in Front (\"\")"="", "State(s) in (\"\")"=w1375) -> ("States Out"=w1380:string)  [unwired: 13 in]
      }
      frame "Macro: Update Sampling" {
        w1395 = T53 10123 items=["Finite Samples"=10178, "Continuous Samples"=10123] ("Sample Mode")
        w1394 = T53 10178 items=["Finite Samples"=10178, "Continuous Samples"=10123] ("Sample Mode")
        # "#todo\nthis \"macro\" needs to\nbe handled by Lockin.DAQ\nor Handle Command"
        n669 = Unbundle By Name(w1385) -> ("Lockin"=w1382:refnum<class "Instrument.Lockin.lvclass">)
        n670 = Unbundle By Name(w1382) -> ("state"=w1381:T35)
        n671 = local read "Start"() -> (w1383:bool)
        n672 = case shown="\"created\", Default" w1381 {
          tunnel: ["" ("State with Arguments") w1407] -> w1389
          frame "idle" {
          }
          frame "created", Default {
            n673 = Format Into String(Set_State-enum."start" ("State")) -> (resulting string=w1408:string)  [unwired: 3 in, 1 out]
            n674 = call <vilib>:"Build State String with Arguments__JKI_lib_State_Machine.vi"("Arguments (\"\")"=w1408, "State"="Lockin SMO: Set State" ("f")) -> ("State with Arguments"=w1407:string)  [unwired: 4 in]
          }
        }
        n675 = case shown="\"created\", Default" w1381 {
          tunnel: ["" ("State with Arguments") w1402] -> w1391
          frame "idle" {
          }
          frame "created", Default {
            n676 = Format Into String(Set_State-enum."stop" ("State")) -> (resulting string=w1405:string)  [unwired: 3 in, 1 out]
            n677 = call <vilib>:"Build State String with Arguments__JKI_lib_State_Machine.vi"("Arguments (\"\")"=w1405, "State"="Lockin SMO: Set State" ("f")) -> ("State with Arguments"=w1402:string)  [unwired: 4 in]
          }
        }
        n678 = Select(t=w1395, s=w1383, f=w1394) -> (s? t:f=w1393:T53)
        n679 = Format Into String(w1393) -> (resulting string=w1392:string)  [unwired: 3 in, 1 out]
        n680 = call <vilib>:"Build State String with Arguments__JKI_lib_State_Machine.vi"("Arguments (\"\")"=w1392, "State"="Lockin SMO: Set Sampling") -> ("State with Arguments"=w1390:string)  [unwired: 4 in]
        n681 = call <vilib>:"Add State(s) to Queue__jki_lib_state_machine.vi"("State(s) in Front (\"\")"=w1391, "State(s) in (\"\")"=w1390, "State(s) at Back (\"\")"=w1389) -> ("States Out"=w1384:string)  [unwired: 12 in]
        n682 = call <vilib>:"Add State(s) to Queue__jki_lib_state_machine.vi"("State(s) in Front (\"\")"="4461: SAMPLING SETUP" ("State(s) in Front (\"\")"), "State(s) in (\"\")"="Configuration: Write" ("State(s) in Front (\"\")"), "State(s) at Back (\"\")"=w1384) -> ("States Out"=w1386:string)  [unwired: 12 in]
        n683 = call <vilib>:"Add State(s) to Queue__jki_lib_state_machine.vi"("State(s) in Front (\"\")"=w1386, "State(s) in (\"\")"=w1400) -> ("States Out"=w1399:string)  [unwired: 13 in]
      }
      frame "Macro: Exit" {
        # "Exit Macro\n(This is called once, when the VI exits)"
        n684 = Unbundle By Name(w1415) -> ("Core.Close Panel on Exit?"=w1419:bool)
        n685 = Select(t="UI: Front Panel State >> Close", s=w1419, f="") -> (s? t:f=w1418:string)
        n686 = call <vilib>:"Add State(s) to Queue__jki_lib_state_machine.vi"("State(s) in Front (\"\")"="Lockin SMO: Set AO Zero Amplitude\nRemote SMO: Stop\nLockin SMO: Stop\nError Logger: Stop\nConfiguration: Write\nUI: Disable Buttons\nUI: Cleanup", "State(s) in (\"\")"=w1418, "State(s) at Back (\"\")"="Events: Unregister\nData: Cleanup\nExit") -> ("States Out"=w1416:string)  [unwired: 12 in]
        n687 = call <vilib>:"Add State(s) to Queue__jki_lib_state_machine.vi"("State(s) in Front (\"\")"=w1416, "State(s) in (\"\")"=w1422) -> ("States Out"=w1421:string)  [unwired: 13 in]
      }
      frame "---------- Error Logger ----------" {
        n688 = call <vilib>:"Add State(s) to Queue__jki_lib_state_machine.vi"("State(s) in (\"\")"=w1427) -> ("States Out"=w1426:string)  [unwired: 14 in]
      }
      frame "Error Logger: Create" {
        w1451 = T60 3 items=["User Home"=0, "User Desktop"=1, "User Documents"=2, "User Application Data"=3, "User Preferences"=4, "User Temporary"=5, "Public Documents"=6, "Public Application Data"=7, "Public Preferences"=8, "Public Cache"=13, "System Core Libraries"=9, "System Installed Libraries"=10, "Application Files"=11, "Boot Volume Root"=12] ("system directory type")
        # "#framework"
        n689 = Unbundle By Name(w1437) -> ("RemoteControl"=w1429:refnum<class "RemoteControl.lvclass">, "Lockin.DAQ"=w1443:refnum<class "Lockin.DAQ.lvclass">, "Logger.Error"=w1446:refnum<class "Logger.Error.lvclass">, "Lockin"=w1430:refnum<class "Instrument.Lockin.lvclass">)
        n690 = call-dynamic "Get SMO Name.vi"("error in (no error)"=w1431, "Instrument.Lockin"=w1430) -> ("error out"=w1432:errorcluster, "SMO Name"=w1434:string, "Instrument.Lockin out"=w1433:refnum<class "Instrument.Lockin.lvclass">)  [unwired: 7 in]
        n691 = call <vilib>:"Get System Directory.vi"("system directory type"=w1451) -> ("system directory"=w1453:path)  [unwired: 10 in]
        n692 = Build Path(base path=w1453, name or relative path="LevyLab") -> (appended path=w1450:path)
        n693 = call <vilib>:"Create.vi"("error in (no error)"=w1432, "SMO"=w1446) -> ("error out"=w1440:errorcluster, "SMO out"=w1445:refnum<class "Logger.Error.lvclass">)  [unwired: 7 in, 1 out]
        n694 = Build Path(base path=w1450, name or relative path="Error Logs") -> (appended path=w1448:path)
        n695 = Build Path(base path=w1448, name or relative path=w1434) -> (appended path=w1447:path)
        n696 = Build Array(w1429, w1443, w1433) -> (w1442:refnum<class "SMO.lvclass">[])
        n697 = call-dynamic "Write path.vi"("error in (no error)"=w1440, "folder"=w1447, "Logger in"=w1445) -> ("error out"=w1441:errorcluster, "Logger out"=w1444:refnum<class "Logger.Error.lvclass">)  [unwired: 7 in]
        n698 = call <userlib>:"Write Dependencies.vi"("error in (no error)"=w1441, "SMOs"=w1442, "Logger.Error in"=w1444) -> ("error out"=w1439:errorcluster, "Logger.Error out"=w1438:refnum<class "Logger.Error.lvclass">)  [unwired: 7 in]
        n699 = call <vilib>:"Start.vi"("error in (no error)"=w1439, "SMO"=w1438) -> ("error out"=w1435:errorcluster, "SMO out"=w1436:refnum<class "Logger.Error.lvclass">)  [unwired: 8 in]
        n700 = Bundle By Name(cluster=w1437, "Logger.Error"=w1436) -> (w1428:T41)
        n701 = call <vilib>:"Add State(s) to Queue__jki_lib_state_machine.vi"("State(s) in (\"\")"=w1456) -> ("States Out"=w1455:string)  [unwired: 14 in]
      }
      frame "Error Logger: Stop" {
        # "#framework"
        n702 = Unbundle By Name(w1462) -> ("Logger.Error"=w1459:refnum<class "Logger.Error.lvclass">)
        n703 = call <vilib>:"GetState.vi"("error in (no error)"=w1458, "SMO"=w1459) -> ("SMO State"=w1460:T16, "SMO out"=w1461:refnum<class "Logger.Error.lvclass">)  [unwired: 7 in, 1 out]
        n704 = case shown="Default" w1460 {
          tunnel: [w1466 w1471] -> w1457
          tunnel: w1461 -> [_ w1474]
          tunnel: w1458 -> [w1466 w1473]
          frame "Stopped" {
          }
          frame Default {
            n705 = call <vilib>:"Stop.vi"("error in (no error)"=w1473, "SMO"=w1474) -> ("error out"=w1470:errorcluster, "SMO out"=w1469:refnum<class "Logger.Error.lvclass">)  [unwired: 8 in]
            n706 = call <vilib>:"GetState.vi"("error in (no error)"=w1470, "SMO"=w1469) -> ("error out"=w1468:errorcluster, "SMO out"=w1467:refnum<class "Logger.Error.lvclass">)  [unwired: 7 in, 1 out]
            n707 = call <vilib>:"Destroy.vi"("error in (no error)"=w1468, "SMO"=w1467) -> ("error out"=w1472:errorcluster)  [unwired: 9 in]
            n708 = call <vilib>:"Clear Errors.vi"("error in (no error)"=w1472) -> ("error out"=w1471:errorcluster)  [unwired: 5 in, 1 out]
          }
        }
        n709 = call <vilib>:"Add State(s) to Queue__jki_lib_state_machine.vi"("State(s) in (\"\")"=w1465) -> ("States Out"=w1464:string)  [unwired: 14 in]
      }
      frame "---------- Remote SMO ----------" {
        n710 = call <vilib>:"Add State(s) to Queue__jki_lib_state_machine.vi"("State(s) in (\"\")"=w1479) -> ("States Out"=w1478:string)  [unwired: 14 in]
      }
      frame "Remote SMO: Create" {
        # "#framework"
        n711 = Unbundle By Name(w1482) -> ("RemoteControl"=w1488:refnum<class "RemoteControl.lvclass">)
        n712 = Unbundle By Name(w1482) -> ("Lockin"=w1483:refnum<class "Instrument.Lockin.lvclass">)
        n713 = call <vilib>:"GetState.vi"("error in (no error)"=w1489, "SMO"=w1488) -> ("error out"=w1484:errorcluster, "SMO State"=w1487:T16, "SMO out"=w1486:refnum<class "RemoteControl.lvclass">)  [unwired: 7 in]
        n714 = call <vilib>:"Clear Errors.vi"("error in (no error)"=w1484) -> ("error out"=w1480:errorcluster)  [unwired: 5 in, 1 out]
        n715 = case shown="Default" w1487 {
          tunnel: [w1494 w1500] -> w1490
          tunnel: w1480 -> [w1494 _]
          tunnel: w1486 -> [_ _]
          tunnel: w1483 -> [_ w1508]
          tunnel: w1482 -> [w1493 w1514]
          tunnel: [w1493 w1513] -> w1481
          frame "Created".."Stopped" {
          }
          frame Default {
            # "this program acts as the command \"server\"\nthe list of methods is maintained here."
            n716 = call-dynamic "Get SMO RC Type.vi"("Instrument in"=w1508) -> ("error out"=w1501:errorcluster, "RC Type"=w1506:T61, "Instrument out"=w1507:refnum<class "Instrument.Lockin.lvclass">)  [unwired: 8 in]
            n717 = call <userlib>:"RC Enum to RC Object.vi"("error in (no error)"=w1501, "RC Type"=w1506) -> ("error out"=w1502:errorcluster, "RemoteControl out"=w1505:refnum<class "RemoteControl.lvclass">)  [unwired: 8 in]
            n718 = call-dynamic "Get SMO Port.vi"("error in (no error)"=w1502, "Instrument.Lockin in"=w1507) -> ("error out"=w1511:errorcluster, "Port"=w1504:u16, "Instrument.Lockin out"=w1512:refnum<class "Instrument.Lockin.lvclass">)  [unwired: 7 in]
            n719 = call-dynamic "Write Port.vi"("error in (no error)"=w1511, "Port"=w1504, "RemoteControl in"=w1505) -> ("error out"=w1510:errorcluster, "RemoteControl out"=w1518:refnum<class "RemoteControl.lvclass">)  [unwired: 7 in]
            n720 = local read "Allowed remote system"() -> (w1517:string)
            n721 = call-dynamic "Get SMO Public API.vi"("error in (no error)"=w1510, "Instrument.Lockin"=w1512) -> ("error out"=w1509:errorcluster, "Commands"=w1515:string[])  [unwired: 7 in, 1 out]
            n722 = call-dynamic "Write Commands.vi"("error in (no error)"=w1509, "Commands"=w1515, "RemoteControl in"=w1518) -> ("error out"=w1497:errorcluster, "RemoteControl out"=w1499:refnum<class "RemoteControl.lvclass">)  [unwired: 7 in]
            n723 = call <userlib>:"Write Debug Mode.vi"("error in (no error)"=w1497, "Debug Mode?"=FALSE, "RemoteControl in"=w1499) -> ("error out"=w1496:errorcluster, "RemoteControl out"=w1498:refnum<class "RemoteControl.lvclass">)  [unwired: 7 in]
            n724 = call-dynamic "Create Server SMO.vi"("error in (no error)"=w1496, "RemoteControl in"=w1498) -> ("error out"=w1500:errorcluster, "RemoteControl out"=w1503:refnum<class "RemoteControl.lvclass">)  [unwired: 8 in]
            n725 = Bundle By Name(cluster=w1514, "RemoteControl.Configure.address"="127.0.0.1", "RemoteControl.Configure.Port"=w1504, "RemoteControl.Configure.AllowedRemote"=w1517, "RemoteControl.Configure.Commands"=w1515, "RemoteControl"=w1503) -> (w1513:T41)
          }
        }
        n726 = call <vilib>:"Add State(s) to Queue__jki_lib_state_machine.vi"("State(s) in (\"\")"=w1492) -> ("States Out"=w1491:string)  [unwired: 14 in]
      }
      frame "Remote SMO: Start" {
        # "#framework"
        n727 = Unbundle By Name(w1520) -> ("RemoteControl"=w1527:refnum<class "RemoteControl.lvclass">)
        n728 = call <vilib>:"GetState.vi"("error in (no error)"=w1528, "SMO"=w1527) -> ("error out"=w1521:errorcluster, "SMO State"=w1526:T16, "SMO out"=w1525:refnum<class "RemoteControl.lvclass">)  [unwired: 7 in]
        n729 = call <vilib>:"Clear Errors.vi"("error in (no error)"=w1521) -> ("error out"=w1523:errorcluster)  [unwired: 5 in, 1 out]
        n730 = case shown="Default" w1526 {
          tunnel: [w1531 w1538] -> w1522
          tunnel: [w1532 w1534] -> w1519
          tunnel: w1523 -> [w1531 w1536]
          tunnel: w1520 -> [w1532 w1535]
          tunnel: w1525 -> [_ w1537]
          frame "Started" {
          }
          frame Default {
            # "Start SMO"
            n731 = call <vilib>:"Start.vi"("error in (no error)"=w1536, "SMO"=w1537) -> ("error out"=w1538:errorcluster, "SMO out"=w1533:refnum<class "RemoteControl.lvclass">)  [unwired: 8 in]
            n732 = Bundle By Name(cluster=w1535, "RemoteControl"=w1533) -> (w1534:T41)
          }
        }
        n733 = call <vilib>:"Add State(s) to Queue__jki_lib_state_machine.vi"("State(s) in (\"\")"=w1530) -> ("States Out"=w1529:string)  [unwired: 14 in]
      }
      frame "Remote SMO: AllowedRemote" {
        # "#framework\nbut unused..."
        # "only an \"allowed remote system\" is allowed to control this VI"
        n734 = Unbundle By Name(w1545) -> ("RemoteControl"=w1540:refnum<class "RemoteControl.lvclass">, "RemoteControl.Configure"=w1539:T37)
        n735 = local read "Allowed remote system"() -> (w1542:string)
        n736 = Bundle By Name(cluster=w1539, "AllowedRemote"=w1542) -> (w1541:T37)
        n737 = call <userlib>:"RemoteControl.Configure.vi"("error in (no error)"=w1544, "Configure"=w1541, "RemoteControl"=w1540) -> ("error out"=w1543:errorcluster)  [unwired: 7 in, 1 out]
        n738 = call <vilib>:"Add State(s) to Queue__jki_lib_state_machine.vi"("State(s) in (\"\")"=w1548) -> ("States Out"=w1547:string)  [unwired: 14 in]
      }
      frame "Remote SMO: Reply to Command" {
        # "#framework"
        # "responds to the RC:process"
        n739 = Unbundle By Name(w1553) -> ("RemoteControl"=w1554:refnum<class "RemoteControl.lvclass">, "HandledMessage"=w1550:T38)
        n740 = Bundle("HandledMessage"=w1550) -> (w1549:cluster{"HandledMessage":T38})  [unwired: 1 in]
        n741 = call <userlib>:"RemoteControl.SendMessageToProcess.vi"("error in (no error)"=w1552, "SendMessageToProcess"=w1549, "RemoteControl"=w1554) -> ("error out"=w1551:errorcluster)  [unwired: 7 in, 1 out]
        n742 = call <vilib>:"Add State(s) to Queue__jki_lib_state_machine.vi"("State(s) in (\"\")"=w1557) -> ("States Out"=w1556:string)  [unwired: 14 in]
      }
      frame "Remote SMO: Stop" {
        # "#framework"
        n743 = Unbundle By Name(w1560) -> ("RemoteControl"=w1564:refnum<class "RemoteControl.lvclass">)
        n744 = call <vilib>:"GetState.vi"("error in (no error)"=w1562, "SMO"=w1564) -> ("SMO State"=w1558:T16, "SMO out"=w1563:refnum<class "RemoteControl.lvclass">)  [unwired: 7 in, 1 out]
        n745 = case shown="Default" w1558 {
          tunnel: [w1567 w1572] -> w1559
          tunnel: w1563 -> [_ w1575]
          tunnel: w1562 -> [w1567 w1574]
          frame "Stopped" {
          }
          frame Default {
            n746 = call <vilib>:"Stop.vi"("error in (no error)"=w1574, "SMO"=w1575) -> ("error out"=w1571:errorcluster, "SMO out"=w1570:refnum<class "RemoteControl.lvclass">)  [unwired: 8 in]
            n747 = call <vilib>:"GetState.vi"("error in (no error)"=w1571, "SMO"=w1570) -> ("error out"=w1569:errorcluster, "SMO out"=w1568:refnum<class "RemoteControl.lvclass">)  [unwired: 7 in, 1 out]
            n748 = call <vilib>:"Destroy.vi"("error in (no error)"=w1569, "SMO"=w1568) -> ("error out"=w1573:errorcluster)  [unwired: 9 in]
            n749 = call <vilib>:"Clear Errors.vi"("error in (no error)"=w1573) -> ("error out"=w1572:errorcluster)  [unwired: 5 in, 1 out]
          }
        }
        n750 = call <vilib>:"Add State(s) to Queue__jki_lib_state_machine.vi"("State(s) in (\"\")"=w1566) -> ("States Out"=w1565:string)  [unwired: 14 in]
      }
      frame "---------- Lockin SMO ----------" {
        n751 = call <vilib>:"Add State(s) to Queue__jki_lib_state_machine.vi"("State(s) in (\"\")"=w1580) -> ("States Out"=w1579:string)  [unwired: 14 in]
      }
      frame "Lockin SMO: Create" {
        # "#framework"
        n752 = Unbundle By Name(w1583) -> ("Lockin.DAQ"=w1591:refnum<class "Lockin.DAQ.lvclass">)
        n753 = call <vilib>:"GetState.vi"("error in (no error)"=w1581, "SMO"=w1591) -> ("error out"=w1585:errorcluster, "SMO State"=w1590:T16, "SMO out"=w1588:refnum<class "Lockin.DAQ.lvclass">)  [unwired: 7 in]
        n754 = call <vilib>:"Clear Errors.vi"("error in (no error)"=w1585) -> ("error out"=w1589:errorcluster)  [unwired: 5 in, 1 out]
        n755 = case shown="Default" w1590 {
          tunnel: [w1595 w1596] -> w1584
          tunnel: w1589 -> [w1595 w1599]
          tunnel: w1588 -> [w1594 w1598]
          tunnel: [w1594 w1597] -> w1586
          frame "Created".."Stopped" {
          }
          frame Default {
            n756 = call <vilib>:"Create.vi"("error in (no error)"=w1599, "SMO"=w1598) -> ("error out"=w1596:errorcluster, "SMO out"=w1597:refnum<class "Lockin.DAQ.lvclass">)  [unwired: 7 in, 1 out]
          }
        }
        n757 = Bundle By Name(cluster=w1583, "Lockin.DAQ"=w1586) -> (w1582:T41)
        n758 = call <vilib>:"Add State(s) to Queue__jki_lib_state_machine.vi"("State(s) in (\"\")"=w1593) -> ("States Out"=w1592:string)  [unwired: 14 in]
      }
      frame "Lockin SMO: Start" {
        # "#framework"
        n759 = Unbundle By Name(w1600) -> ("Lockin.DAQ"=w1610:refnum<class "Lockin.DAQ.lvclass">)
        n760 = call <vilib>:"GetState.vi"("error in (no error)"=w1604, "SMO"=w1610) -> ("error out"=w1602:errorcluster, "SMO State"=w1609:T16, "SMO out"=w1608:refnum<class "Lockin.DAQ.lvclass">)  [unwired: 7 in]
        n761 = call <vilib>:"Clear Errors.vi"("error in (no error)"=w1602) -> ("error out"=w1603:errorcluster)  [unwired: 5 in, 1 out]
        n762 = case shown="Default" w1609 {
          tunnel: [w1614 w1618] -> w1605
          tunnel: w1603 -> [w1614 w1617]
          tunnel: w1608 -> [w1613 w1616]
          tunnel: [w1613 w1615] -> w1606
          frame "Started" {
          }
          frame Default {
            n763 = call <vilib>:"Start.vi"("error in (no error)"=w1617, "SMO"=w1616) -> ("error out"=w1618:errorcluster, "SMO out"=w1615:refnum<class "Lockin.DAQ.lvclass">)  [unwired: 8 in]
          }
        }
        n764 = Bundle By Name(cluster=w1600, "Lockin.DAQ"=w1606) -> (w1601:T41)
        n765 = call <vilib>:"Add State(s) to Queue__jki_lib_state_machine.vi"("State(s) in (\"\")"=w1612) -> ("States Out"=w1611:string)  [unwired: 14 in]
      }
      frame "Lockin SMO: Stop" {
        # "#framework"
        n766 = Unbundle By Name(w1619) -> ("Lockin.DAQ"=w1621:refnum<class "Lockin.DAQ.lvclass">)
        n767 = call "Lockin.DAQ.setstate.vi"("error in (no error)"=w1622, "State"=Set_State-enum."stop", "Lockin.DAQ"=w1621) -> ("error out"=w1624:errorcluster, "Lockin.DAQ out"=w1623:refnum<class "Lockin.DAQ.lvclass">)  [unwired: 7 in]
        n768 = call <vilib>:"GetState.vi"("error in (no error)"=w1624, "SMO"=w1623) -> ("SMO State"=w1626:T16, "SMO out"=w1627:refnum<class "Lockin.DAQ.lvclass">)  [unwired: 7 in, 1 out]
        n769 = case shown="Default" w1626 {
          tunnel: [w1631 w1637] -> w1628
          tunnel: w1627 -> [_ w1640]
          tunnel: w1624 -> [w1631 w1639]
          frame "Stopped" {
          }
          frame Default {
            n770 = call <vilib>:"Stop.vi"("error in (no error)"=w1639, "SMO"=w1640) -> ("error out"=w1636:errorcluster, "SMO out"=w1635:refnum<class "Lockin.DAQ.lvclass">)  [unwired: 8 in]
            n771 = call <vilib>:"GetState.vi"("error in (no error)"=w1636, "SMO"=w1635) -> ("error out"=w1634:errorcluster, "SMO State"=w1632:T16, "SMO out"=w1633:refnum<class "Lockin.DAQ.lvclass">)  [unwired: 7 in]
            n772 = local write "LockinDAQ SMO State"(w1632) -> ()
            n773 = call <vilib>:"Destroy.vi"("error in (no error)"=w1634, "SMO"=w1633) -> ("error out"=w1638:errorcluster)  [unwired: 9 in]
            n774 = call <vilib>:"Clear Errors.vi"("error in (no error)"=w1638) -> ("error out"=w1637:errorcluster)  [unwired: 5 in, 1 out]
          }
        }
        n775 = call <vilib>:"Add State(s) to Queue__jki_lib_state_machine.vi"("State(s) in (\"\")"=w1630) -> ("States Out"=w1629:string)  [unwired: 14 in]
      }
      frame "Lockin SMO: Set State" {
        n776 = Unbundle By Name(w1641) -> ("Lockin.DAQ"=w1647:refnum<class "Lockin.DAQ.lvclass">)
        n777 = case shown="\"stop\", Default" w1643 {
          tunnel: [Set_State-enum."stop" ("State") Set_State-enum."start" ("State") Set_State-enum."reset" ("State") Set_State-enum."start sweep" ("State") Set_State-enum."stop sweep" ("State")] -> w1642
          tunnel: [FALSE ("Trigger") TRUE ("Trigger") w1655 TRUE ("Trigger") TRUE ("Trigger")] -> w1644
          frame "stop", Default {
          }
          frame "start" {
          }
          frame "reset" {
            n778 = local read "Start"() -> (w1655:bool)
          }
          frame "start sweep" {
          }
          frame "stop sweep" {
          }
        }
        n779 = local write "Start"(w1644) -> ()
        n780 = call "Lockin.DAQ.setstate.vi"("error in (no error)"=w1646, "State"=w1642, "Lockin.DAQ"=w1647) -> ("error out"=w1645:errorcluster)  [unwired: 7 in, 1 out]
        n781 = call <vilib>:"Add State(s) to Queue__jki_lib_state_machine.vi"("State(s) in (\"\")"=w1650) -> ("States Out"=w1649:string)  [unwired: 14 in]
      }
      frame "Lockin SMO: Set AI Config" {
        n782 = Unbundle By Name(w1662) -> ("Lockin.DAQ"=w1667:refnum<class "Lockin.DAQ.lvclass">, "Lockin"=w1663:refnum<class "Instrument.Lockin.lvclass">)
        n783 = Unbundle By Name(w1663) -> ("AI Configuration"=w1664:T51)
        n784 = call "Lockin.DAQ.setAIconfig.vi"("error in (no error)"=w1666, "Simulation mode"="AI Simulation mode", "AI Configuration"=w1664, "Lockin.DAQ"=w1667) -> ("error out"=w1665:errorcluster)  [unwired: 6 in, 1 out]
        n785 = call <vilib>:"Add State(s) to Queue__jki_lib_state_machine.vi"("State(s) in (\"\")"=w1670) -> ("States Out"=w1669:string)  [unwired: 14 in]
      }
      frame "Lockin SMO: Set AO Config" {
        n786 = Unbundle By Name(w1672) -> ("Lockin.DAQ"=w1676:refnum<class "Lockin.DAQ.lvclass">, "Lockin"=w1673:refnum<class "Instrument.Lockin.lvclass">)
        n787 = Unbundle By Name(w1673) -> ("AO Configuration"=w1671:T49)
        n788 = call "Lockin.DAQ.setAOconfig.vi"("error in (no error)"=w1675, "AO Configuration"=w1671, "Lockin.DAQ"=w1676) -> ("error out"=w1674:errorcluster)  [unwired: 7 in, 1 out]
        n789 = call <vilib>:"Add State(s) to Queue__jki_lib_state_machine.vi"("State(s) in (\"\")"=w1679) -> ("States Out"=w1678:string)  [unwired: 14 in]
      }
      frame "Lockin SMO: Set Sampling" {
        w1681 = 100  # AI Buffer Size (S)
        # "Is there a more elegant way to do this?"
        n790 = Unbundle By Name(w1682) -> ("Lockin.DAQ"=w1689:refnum<class "Lockin.DAQ.lvclass">, "Lockin"=w1685:refnum<class "Instrument.Lockin.lvclass">)
        n791 = case shown="\"10123\"" w1684 {
          tunnel: [w1693 w1694] -> w1686
          frame "10178", Default {
            w1693 = T53 10178 items=["Finite Samples"=10178, "Continuous Samples"=10123] ("Sample Mode")
          }
          frame "10123" {
            w1694 = T53 10123 items=["Finite Samples"=10178, "Continuous Samples"=10123] ("Sample Mode")
          }
        }
        n792 = Unbundle By Name(w1685) -> ("sampling"=w1683:T11)
        n793 = call "Lockin.DAQ.setSampling.vi"("Decimation"="decimating factor", "AI Buffer Size (S)"=w1681, "error in (no error)"=w1688, "Sample Mode"=w1686, "Sampling"=w1683, "Lockin.DAQ"=w1689) -> ("error out"=w1687:errorcluster)  [unwired: 4 in, 1 out]
        n794 = call <vilib>:"Add State(s) to Queue__jki_lib_state_machine.vi"("State(s) in (\"\")"=w1692) -> ("States Out"=w1691:string)  [unwired: 14 in]
      }
      frame "Lockin SMO: Set AO" {
        n795 = Unbundle By Name(w1695) -> ("Lockin.DAQ"=w1700:refnum<class "Lockin.DAQ.lvclass">, "Lockin"=w1697:refnum<class "Instrument.Lockin.lvclass">)
        n796 = Unbundle By Name(w1697) -> ("AO Channels"=w1696:T45)
        n797 = call "Lockin.DAQ.setAO.vi"("error in (no error)"=w1699, "AO Channels"=w1696, "Lockin.DAQ"=w1700) -> ("error out"=w1698:errorcluster)  [unwired: 7 in, 1 out]
        n798 = call <vilib>:"Add State(s) to Queue__jki_lib_state_machine.vi"("State(s) in (\"\")"=w1703) -> ("States Out"=w1702:string)  [unwired: 14 in]
      }
      frame "Lockin SMO: Set AO Zero Amplitude" {
        n799 = Unbundle By Name(w1710) -> ("Lockin.DAQ"=w1717:refnum<class "Lockin.DAQ.lvclass">, "Lockin"=w1709:refnum<class "Instrument.Lockin.lvclass">)
        n800 = Unbundle By Name(w1709) -> ("AO Channels"=w1704:T45, "#s"=w1715:i32, "Fs"=w1714:dbl)
        n801 = Divide(x=w1715, y=w1714) -> (x/y=w1707:dbl)
        n802 = Multiply(x=1000.0 ("y"), y=w1707) -> (x*y=w1713:dbl)
        n803 = for {
          tunnel: w1704 -> [w1723] mode=indexing
          tunnel: [w1721] -> w1706 mode=indexing
          n804 = Bundle By Name(cluster=w1723, "Amplitude"=0.0 ("element")) -> (w1721:T3)
        }
        n805 = To Unsigned Long Integer(number=w1713) -> (unsigned 32bit integer=w1712:u32)
        n806 = call "Lockin.DAQ.setAO.vi"("error in (no error)"=w1716, "AO Channels"=w1706, "Lockin.DAQ"=w1717) -> ("error out"=w1705:errorcluster)  [unwired: 7 in, 1 out]
        n807 = call <userlib>:"Wait (ms)__ogtk.vi"("error in (no error)"=w1705, "milliseconds to wait"=w1712) -> ("error out"=w1711:errorcluster)  [unwired: 8 in, 1 out]
        n808 = call <vilib>:"Add State(s) to Queue__jki_lib_state_machine.vi"("State(s) in (\"\")"=w1720) -> ("States Out"=w1719:string)  [unwired: 14 in]
      }
      frame "Lockin SMO: Set REF" {
        n809 = Unbundle By Name(w1726) -> ("Lockin.DAQ"=w1729:refnum<class "Lockin.DAQ.lvclass">, "Lockin"=w1727:refnum<class "Instrument.Lockin.lvclass">)
        n810 = Unbundle By Name(w1727) -> ("REF Channels"=w1724:T46)
        n811 = call "Lockin.DAQ.setREF.vi"("error in (no error)"=w1725, "Channels: Lockin"=w1724, "Lockin.DAQ"=w1729) -> ("error out"=w1728:errorcluster)  [unwired: 7 in, 1 out]
        n812 = call <vilib>:"Add State(s) to Queue__jki_lib_state_machine.vi"("State(s) in (\"\")"=w1732) -> ("States Out"=w1731:string)  [unwired: 14 in]
      }
      frame "Lockin SMO: Set AI" {
        n813 = Unbundle By Name(w1737) -> ("Lockin.DAQ"=w1736:refnum<class "Lockin.DAQ.lvclass">, "Lockin"=w1738:refnum<class "Instrument.Lockin.lvclass">)
        n814 = Unbundle By Name(w1738) -> ("AI Channels"=w1733:T59)
        n815 = call "Lockin.DAQ.setAI.vi"("error in (no error)"=w1735, "AI Channels"=w1733, "Lockin.DAQ"=w1736) -> ("error out"=w1734:errorcluster)  [unwired: 7 in, 1 out]
        n816 = call <vilib>:"Add State(s) to Queue__jki_lib_state_machine.vi"("State(s) in (\"\")"=w1741) -> ("States Out"=w1740:string)  [unwired: 14 in]
      }
      frame "Lockin SMO: Set Input Gain" {
        n817 = Unbundle By Name(w1742) -> ("Lockin.DAQ"=w1747:refnum<class "Lockin.DAQ.lvclass">, "Lockin"=w1745:refnum<class "Instrument.Lockin.lvclass">)
        n818 = Unbundle By Name(w1745) -> ("Input Gain"=w1744:dbl[])
        n819 = call "Lockin.DAQ.setInputGain.vi"("error in (no error)"=w1743, "setInputGain"=w1744, "Lockin.DAQ"=w1747) -> ("error out"=w1746:errorcluster)  [unwired: 7 in, 1 out]
        n820 = call <vilib>:"Add State(s) to Queue__jki_lib_state_machine.vi"("State(s) in (\"\")"=w1750) -> ("States Out"=w1749:string)  [unwired: 14 in]
      }
      frame "Lockin SMO: Set Output Gain" {
        n821 = Unbundle By Name(w1755) -> ("Lockin.DAQ"=w1754:refnum<class "Lockin.DAQ.lvclass">, "Lockin"=w1756:refnum<class "Instrument.Lockin.lvclass">)
        n822 = Unbundle By Name(w1756) -> ("Output Gain"=w1752:dbl[])
        n823 = call "Lockin.DAQ.setOutputGain.vi"("error in (no error)"=w1753, "setOutputGain"=w1752, "Lockin.DAQ"=w1754) -> ("error out"=w1751:errorcluster)  [unwired: 7 in, 1 out]
        n824 = call <vilib>:"Add State(s) to Queue__jki_lib_state_machine.vi"("State(s) in (\"\")"=w1759) -> ("States Out"=w1758:string)  [unwired: 14 in]
      }
      frame "Lockin SMO: Set Prefilter" {
        n825 = Unbundle By Name(w1762) -> ("Lockin.DAQ"=w1764:refnum<class "Lockin.DAQ.lvclass">, "Lockin"=w1765:refnum<class "Instrument.Lockin.lvclass">)
        n826 = Unbundle By Name(w1765) -> ("REF Filter"=w1763:T62)
        n827 = call "Lockin.DAQ.setPreFilter.vi"("error in (no error)"=w1761, "PreFilter"=w1763, "Lockin.DAQ"=w1764) -> ("error out"=w1760:errorcluster)  [unwired: 7 in, 1 out]
        n828 = call <vilib>:"Add State(s) to Queue__jki_lib_state_machine.vi"("State(s) in (\"\")"=w1768) -> ("States Out"=w1767:string)  [unwired: 14 in]
      }
      frame "Lockin SMO: Calibration" {
        # "This will only get the current calibration inf\nActually doing calibration is done via Set State >> Calibration"
        n829 = Unbundle By Name(w1774) -> ("Lockin.DAQ"=w1773:refnum<class "Lockin.DAQ.lvclass">)
        n830 = case shown="\"True\"" w1769 {
          tunnel: [T27 FALSE ("setCalibration") T27 TRUE ("setCalibration")] -> w1770
          frame "False", Default {
            # "check calibration"
          }
          frame "True" {
            # "calibrate"
          }
        }
        n831 = call "Lockin.DAQ.setCalibration.vi"("error in (no error)"=w1772, "setCalibration"=w1770, "Lockin.DAQ"=w1773) -> ("error out"=w1771:errorcluster)  [unwired: 7 in, 1 out]
        n832 = call <vilib>:"Add State(s) to Queue__jki_lib_state_machine.vi"("State(s) in (\"\")"=w1777) -> ("States Out"=w1776:string)  [unwired: 14 in]
      }
      frame "Lockin SMO: Auto DAQ" {
        n833 = Unbundle By Name(w1783) -> ("Lockin.DAQ"=w1782:refnum<class "Lockin.DAQ.lvclass">)
        n834 = call "Lockin.DAQ.autoConfigureDAQ.vi"("error in (no error)"=w1781, "Lockin.DAQ"=w1782) -> ("error out"=w1780:errorcluster)  [unwired: 8 in, 1 out]
        n835 = call <vilib>:"Add State(s) to Queue__jki_lib_state_machine.vi"("State(s) in (\"\")"=w1786) -> ("States Out"=w1785:string)  [unwired: 14 in]
      }
      frame "Lockin SMO: Reset Phase" {
        n836 = Unbundle By Name(w1791) -> ("Lockin.DAQ"=w1790:refnum<class "Lockin.DAQ.lvclass">)
        n837 = call "Lockin.DAQ.ResetPhase.vi"("error in (no error)"=w1789, "Reset Phase"=T28 TRUE, "Lockin.DAQ"=w1790) -> ("error out"=w1788:errorcluster)  [unwired: 7 in, 1 out]
        n838 = call <vilib>:"Add State(s) to Queue__jki_lib_state_machine.vi"("State(s) in (\"\")"=w1794) -> ("States Out"=w1793:string)  [unwired: 14 in]
      }
      frame "Lockin SMO: Measure Offset" {
        n839 = Unbundle By Name(w1795) -> ("Lockin.DAQ"=w1799:refnum<class "Lockin.DAQ.lvclass">)
        n840 = call "Lockin.DAQ.measureOffset.vi"("error in (no error)"=w1797, "measureOffset"=T29 TRUE, "Lockin.DAQ"=w1799) -> ("error out"=w1796:errorcluster)  [unwired: 7 in, 1 out]
        n841 = call <vilib>:"Add State(s) to Queue__jki_lib_state_machine.vi"("State(s) in (\"\")"=w1802) -> ("States Out"=w1801:string)  [unwired: 14 in]
      }
      frame "Lockin SMO: Remove Offset" {
        n842 = Unbundle By Name(w1804) -> ("Lockin.DAQ"=w1807:refnum<class "Lockin.DAQ.lvclass">)
        n843 = call "Lockin.DAQ.zeroOffset.vi"("error in (no error)"=w1805, "zeroOffset"=T30 TRUE, "Lockin.DAQ"=w1807) -> ("error out"=w1803:errorcluster)  [unwired: 7 in, 1 out]
        n844 = call <vilib>:"Add State(s) to Queue__jki_lib_state_machine.vi"("State(s) in (\"\")"=w1810) -> ("States Out"=w1809:string)  [unwired: 14 in]
      }
      frame "---------- 4461----------" {
        n845 = call <vilib>:"Add State(s) to Queue__jki_lib_state_machine.vi"("State(s) in (\"\")"=w1815) -> ("States Out"=w1814:string)  [unwired: 14 in]
      }
      frame "4461: SAMPLING SETUP" {
        # "#todo\n*I think* this \"macro\" needs to\nbe handled by Lockin.DAQ\nor Handle Command"
        # "#macro sorta"
        # "#todo\nshould this be in Lockin.DAQ SMO? or in Handle Command?"
        # "Max Fs"
        n846 = Unbundle By Name(w1817) -> ("Lockin"=w1819:refnum<class "Instrument.Lockin.lvclass">)
        n847 = case shown="\"USB 4431\"" "DAQ Type" {
          tunnel: [102400.0 ("upper limit") 204800.0 ("upper limit")] -> w1820
          frame "USB 4431" {
          }
          frame Default {
          }
        }
        n848 = case shown="\"Auto Fs\"" "Sampling Mode" {
          tunnel: [w1833 w1834 w1848] -> w1822
          tunnel: w1819 -> [_ w1836 _]
          tunnel: w1820 -> [_ w1839 w1849]
          tunnel: "Max Fs Refresh Rate (Hz)" -> [_ _ w1844]
          frame "Manual", Default {
            n849 = local read "Sampling"() -> (w1833:T11)
          }
          frame "Auto Fs" {
            # "#todo: owned by Lockin or LockinDAQ?"
            # "#todo: make subVI?"
            # "max Fs"
            n850 = Unbundle By Name(w1836) -> ("AO Channels"=w1840:T45)
            n851 = Index Array(array=w1840) -> (element=w1837:T3)  [unwired: 1 in]
            n852 = Unbundle By Name(w1837) -> ("Frequency"=w1835:dbl)
            n853 = Multiply(x="Auto x*F1", y=w1835) -> (x*y=w1838:dbl)
            n854 = In Range and Coerce(upper limit=w1839, x=w1838, lower limit=1000.0) -> (coerced(x)=w1843:dbl)  [unwired: 1 out]
            n855 = call "Fs and Ns for integer periods.vi"("f integer"=w1835, "Max Fs"=w1843) -> ("Timing out"=w1834:T11)  [unwired: 9 in]
          }
          frame "Max Fs" {
            n856 = Divide(x=w1849, y=w1844) -> (x/y=w1847:dbl)
            n857 = To Long Integer(number=w1847) -> (32bit integer=w1846:i32)
            n858 = Bundle By Name(cluster=T11 {"Fs"=204789.0, "#s"=15753} ("Sampling"), "Fs"=w1849, "#s"=w1846) -> (w1848:T11)
          }
        }
        n859 = call "Coerce Timing.vi"("Max Fs"=w1820, "Sampling in"=w1822) -> ("Sampling out"=w1821:T11)  [unwired: 9 in]
        n860 = call "Write sampling.vi"("error in (no error)"=w1825, "sampling"=w1821, "Instrument.Lockin in"=w1819) -> ("error out"=w1824:errorcluster, "Instrument.Lockin out"=w1823:refnum<class "Instrument.Lockin.lvclass">)  [unwired: 7 in]
        n861 = Bundle By Name(cluster=w1817, "Lockin"=w1823) -> (w1816:T41)
        n862 = local write "Sampling"(w1821) -> ()
        n863 = call <vilib>:"Add State(s) to Queue__jki_lib_state_machine.vi"("State(s) in (\"\")"=w1830) -> ("States Out"=w1829:string)  [unwired: 14 in]
      }
      frame "4461: OUT" {
        # "#todo\nmove to Lockin.DAQ?"
        n864 = Unbundle By Name(w1851) -> ("Lockin"=w1854:refnum<class "Instrument.Lockin.lvclass">)
        n865 = case shown="True" "Enable Output" {
          tunnel: [w1858 w1867] -> w1852
          tunnel: w1854 -> [_ w1870]
          tunnel: w1850 -> [w1858 w1865]
          frame False {
          }
          frame True {
            # "this will act as a self-call\nmeaning after the remote call comes\nin the data on the data bus will get updated\nby other means"
            n866 = Unbundle By Name(w1870) -> ("Results (Dictionary)"=w1866:cluster{"key":string, "value":dbl}[], "Input Gain"=w1860:dbl[])
            n867 = call "Parse Results (single).vi"("Type"="Type", "error in (no error)"=w1865, "Reference Channel"="Reference Channel", "AI Channel"="AI Channel", "Results (Dictionary)"=w1866) -> ("error out"=w1864:errorcluster, "Data"=w1868:dbl)  [unwired: 3 in, 2 out]
            n868 = Decrement(x="AI Channel") -> (x-1=w1859:i32)
            n869 = Index Array(array=w1860, index=w1859) -> (element=w1869:dbl)
            n870 = Multiply(x=w1868, y=w1869) -> (x*y=w1871:dbl)
            "Output (V)" <- w1871
            n871 = call "setAO_DC.vi"("error in (no error)"=w1864, "DC (V)"=w1871, "AO Channel"="Output Channel", "Instrument.Lockin in"=w1870) -> ("error out"=w1867:errorcluster)  [unwired: 6 in, 1 out]
          }
        }
        n872 = call <vilib>:"Add State(s) to Queue__jki_lib_state_machine.vi"("State(s) in (\"\")"=w1856) -> ("States Out"=w1857:string)  [unwired: 14 in]
      }
      frame "4461: FFT" {
        n873 = Unbundle By Name(w1891) -> ("Lockin"=w1890:refnum<class "Instrument.Lockin.lvclass">)
        n874 = Unbundle By Name(w1890) -> ("AI WFM"=w1880:waveform(dbl)[])
        n875 = Bundle By Name(cluster=T31 {"averaging mode"=enum."No averaging", "weighting mode"=enum."Exponential", "number of averages"=10} ("averaging parameters"), "averaging mode"="averaging mode", "weighting mode"="weighting mode", "number of averages"="# averages") -> (w1883:T31)
        n876 = call-poly <vilib>:"FFT Power Spectrum and PSD.vi"("export mode"="export mode", "averaging parameters"=w1883, "restart averaging (F)"="restart", "error in (no error)"=w1879, "dB On (F)"=TRUE, "window"="window", "time signals"=w1880) -> ("error out"=w1892:errorcluster, "averages completed"=→"averages":dbl, "averaging done"=→"done?":bool, "Power Spectrum / PSD"=w1876:cluster{"f0":dbl, "df":dbl, "magnitude":dbl[]}[])  [unwired: 1 in]
        "PS WFGraph" <- w1876
        n877 = control-ref of="PS WFGraph"() -> (w1873:refnum<vi>)
        n878 = for {
          tunnel: [w1899] -> w1878
          tunnel: w1879 -> [w1898]
          tunnel: w1876 -> [_] mode=indexing
          i -> [w1901]
          n879 = property on="PS WFGraph" class="WFGraph (strict)"(error in=w1898, "Active Plot"=w1901) -> (error out=w1902:errorcluster, "Plot.Visible?"=w1900:bool)  [unwired: 1 in, 1 out]
          n880 = property on="PS Chart" class="WFChart (strict)"(error in=w1902, "Active Plot"=w1901, "Plot.Visible?"=w1900) -> (error out=w1899:errorcluster)  [unwired: 1 in, 1 out]
        }
        n881 = call "PS Chart.vi"("error in (no error)"=w1892, "Power Spectrum / PSD"=w1876, "WFGraph (WDT) in"=w1873) -> ("error out"=w1875:errorcluster, "Chart"=→"PS Chart":dbl[][])  [unwired: 7 in]
        n882 = Merge Errors(w1875, w1878) -> (w1874:errorcluster)
        n883 = call <vilib>:"Add State(s) to Queue__jki_lib_state_machine.vi"("State(s) in (\"\")"=w1893) -> ("States Out"=w1897:string)  [unwired: 14 in]
      }
      frame "4461: SAVE" {
        (unwired) i32[] [1, 1] ("X,Y Log")
        (unwired) string[] ["FFT0", "FFT1", "FFT2", "FFT3", "FFT4", "FFT5", "FFT6", "FFT7"] ("wavenames (.Vx, etc)")
        (unwired) string[] ["ch0", "ch1", "ch2", "ch3", "ch4", "ch5", "ch6", "ch7"] ("wavenames (.Vx, etc)")
        # "Wait for Trigger signal from other VI"
        n884 = local read "PS WFGraph"() -> (w1916:cluster{"f0":dbl, "df":dbl, "magnitude":dbl[]}[])
        n885 = Unbundle By Name(w1904) -> ("Lockin"=w1906:refnum<class "Instrument.Lockin.lvclass">)
        n886 = Unbundle By Name(w1906) -> ("AI WFM"=w1907:waveform(dbl)[])
        n887 = for {
          tunnel: w1916 -> [w1933] mode=indexing
          tunnel: [w1928] -> _ mode=indexing
          n888 = Unbundle By Name(w1933) -> ("df"=w1935:dbl, "magnitude"=w1934:dbl[])  [unwired: 1 out]
          n889 = Bundle By Name("dt"=w1935, "Y"=w1934) -> (w1932:waveform(dbl))  [unwired: 1 in]
          n890 = call-poly <vilib>:"Waveform to XY Pairs.vi"("waveform in"=w1932) -> ("XY pairs"=w1931:cluster{"x":timestamp, "y":dbl}[])  [unwired: 8 in, 2 out]
          n891 = for {
            tunnel: w1931 -> [w1939] mode=indexing
            tunnel: [w1937] -> w1929 mode=indexing
            tunnel: [w1936] -> w1930 mode=indexing
            n892 = Unbundle(w1939) -> ("x"=w1938:timestamp, "y"=w1937:dbl)
            n893 = To Double Precision Float(number=w1938) -> (double precision float=w1936:dbl)
          }
          n894 = Bundle(w1930, w1929) -> (w1928:cluster{dbl[], dbl[]})  [unwired: 1 in]
        }
        n895 = Get Date/Time In Seconds() -> (seconds since 1Jan1904=w1915:timestamp)
        n896 = for {
          tunnel: [w1920] -> _ mode=indexing
          tunnel: w1907 -> [w1919] mode=indexing
          n897 = call-poly <vilib>:"Waveform to XY Pairs.vi"("waveform in"=w1919) -> ("XY pairs"=w1923:cluster{"x":timestamp, "y":dbl}[])  [unwired: 8 in, 2 out]
          n898 = for {
            tunnel: w1923 -> [w1927] mode=indexing
            tunnel: [w1925] -> w1921 mode=indexing
            tunnel: [w1924] -> w1922 mode=indexing
            n899 = Unbundle(w1927) -> ("x"=w1926:timestamp, "y"=w1925:dbl)
            n900 = To Double Precision Float(number=w1926) -> (double precision float=w1924:dbl)
          }
          n901 = Bundle(w1922, w1921) -> (w1920:cluster{dbl[], dbl[]})  [unwired: 1 in]
        }
        n902 = Format Date/Time String(time format string (%c)="%Y-%m-%d", seconds (now)=w1915) -> (date/time string=w1914:string)  [unwired: 1 in]
        n903 = Build Path(base path="Path", name or relative path=w1914) -> (appended path=w1913:path)
        n904 = Build Path(base path=w1913, name or relative path="signal" ("filename")) -> ()  [unwired: 1 out]
        n905 = Build Path(base path=w1913, name or relative path="FFT" ("filename")) -> ()  [unwired: 1 out]
        n906 = local write "Save"(FALSE ("SAVE DATA")) -> ()
        n907 = call <vilib>:"Add State(s) to Queue__jki_lib_state_machine.vi"("State(s) in (\"\")"=w1905) -> ("States Out"=w1918:string)  [unwired: 14 in]
      }
      frame "----------Sweep-----------" {
        n908 = call <vilib>:"Add State(s) to Queue__jki_lib_state_machine.vi"("State(s) in (\"\")"=w1944) -> ("States Out"=w1943:string)  [unwired: 14 in]
      }
      frame "---------- AUX ----------" {
        n909 = call <vilib>:"Add State(s) to Queue__jki_lib_state_machine.vi"("State(s) in (\"\")"=w1949) -> ("States Out"=w1948:string)  [unwired: 14 in]
      }
      frame "AUX: Set AUX" {
        # "#todo\nmove to Lockin.DAQ?"
        n910 = call <userlib>:"Voltage Update.vi"("error in (no error)"=w1951, "Amplifier Gain"="Amplifier Gain", "Voltage Output"="Voltage Output (V)", "Physical Channel"="Aux Channel") -> ("error out"=w1950:errorcluster, "Amplified output"=→"Amplified Output (V)":dbl, "DAQ output"=→"DAQ Output (V)":dbl)  [unwired: 5 in]
        n911 = Unbundle By Name(w1953) -> ("Lockin"=w1956:refnum<class "Instrument.Lockin.lvclass">)
        n912 = Bundle By Name(cluster=w1956, "Aux Channel"="Aux Channel") -> (w1955:refnum<class "Instrument.Lockin.lvclass">)
        n913 = Bundle By Name(cluster=w1953, "Lockin"=w1955) -> (w1957:T41)
        n914 = call <vilib>:"Add State(s) to Queue__jki_lib_state_machine.vi"("State(s) in Front (\"\")"="Configuration: Write" ("State(s) in Front (\"\")"), "State(s) in (\"\")"=w1964) -> ("States Out"=w1963:string)  [unwired: 13 in]
      }
      frame "------------Configuration--------------" {
        n915 = call <vilib>:"Add State(s) to Queue__jki_lib_state_machine.vi"("State(s) in (\"\")"=w1969) -> ("States Out"=w1968:string)  [unwired: 14 in]
      }
      frame "Configuration: Initialize" {
        n916 = Unbundle By Name(w1970) -> ("Lockin"=w1976:refnum<class "Instrument.Lockin.lvclass">)
        n917 = call-dynamic "Get SMO Name.vi"("error in (no error)"=w1971, "Instrument.Lockin"=w1976) -> ("error out"=w1973:errorcluster, "SMO Name"=w1977:string, "Instrument.Lockin out"=w1978:refnum<class "Instrument.Lockin.lvclass">)  [unwired: 7 in]
        n918 = call <userlib>:"Write Configuration Path.vi"("error in (no error)"=w1973, "name or relative path"=w1977, "Instrument in"=w1978) -> ("error out"=w1972:errorcluster, "Instrument out"=w1974:refnum<class "Instrument.Lockin.lvclass">)  [unwired: 7 in]
        n919 = Bundle By Name(cluster=w1970, "Lockin"=w1974) -> (w1975:T41)
        n920 = call <vilib>:"Add State(s) to Queue__jki_lib_state_machine.vi"("State(s) in (\"\")"=w1981) -> ("States Out"=w1980:string)  [unwired: 14 in]
      }
      frame "Configuration: Write" {
        n921 = Unbundle By Name(w1982) -> ("Lockin"=w1984:refnum<class "Instrument.Lockin.lvclass">)
        n922 = call-dynamic "Write Configuration File.vi"("error in (no error)"=w1983, "Instrument.Lockin"=w1984) -> ("error out"=w1985:errorcluster)  [unwired: 8 in, 1 out]
        n923 = disable-structure shown="Disabled" {
          disable-tunnel: [w1991 w1992] -> w1986
          disable-tunnel: w1985 -> [w1990 w1992]
          frame Disabled {
            n924 = call "write_lockin_FP_DSC.vi"("error in (no error)"=w1990) -> ("error out"=w1991:errorcluster)  [unwired: 10 in]
          }
          frame Enabled {
          }
        }
        n925 = call <vilib>:"Add State(s) to Queue__jki_lib_state_machine.vi"("State(s) in (\"\")"=w1988) -> ("States Out"=w1989:string)  [unwired: 14 in]
      }
      frame "Configuration: Read" {
        # "Do not write values to FP if error. Eg, if file ini file does not exist yet."
        n926 = Unbundle By Name(w1996) -> ("Lockin"=w2001:refnum<class "Instrument.Lockin.lvclass">)
        n927 = disable-structure shown="Disabled" {
          disable-tunnel: w2002 -> [w2021 _]
          frame Disabled {
            n928 = call "read_lockin_FP_DSC.vi"("error in (no error)"=w2021) -> ()  [unwired: 9 in, 2 out]
          }
          frame Enabled {
          }
        }
        n929 = call-dynamic "Read Configuration File.vi"("error in (no error)"=w2002, "Instrument.Lockin"=w2001) -> ("error out"=w2000:errorcluster, "Instrument.Lockin out"=w1999:refnum<class "Instrument.Lockin.lvclass">)  [unwired: 8 in]
        n930 = call "Lockin.Read Configuration.vi"("error in (no error)"=w2000, "Instrument.Lockin"=w1999) -> ("error out"=w1997:errorcluster, "Configuration"=w1998:T63, "Instrument.Lockin out"=w1995:refnum<class "Instrument.Lockin.lvclass">)  [unwired: 7 in]
        n931 = case shown="No Error" w1997 {
          selector: w1997 -> [w2015 w2020]
          tunnel: w1998 -> [w2017 _]
          tunnel: [w2015 w2019] -> w2003
          tunnel: ["" ("State(s) in Front (\"\")") "//Configuration: Write" ("State(s) in Front (\"\")")] -> w1993
          frame No Error {
            n932 = Unbundle By Name(w2017) -> ("AI Configuration"=w2010:T51, "AO Configuration"=w2009:T49, "AO Channels"=w2013:T45, "REF Channels"=w2012:T46, "Calibration.Cal Info"=w2016:T18[], "DAQ.sampling"=w2011:T11, "Aux Channel"=w2007:tag)  [unwired: 6 out]
            n933 = local write "REF Channels"(w2012) -> ()
            n934 = call "config not UI to UI (AO and AI).vi"("AO Config"=w2009, "AI Config"=w2010) -> ("New Ch []"=w2008:T6[])  [unwired: 8 in, 1 out]
            n935 = local write "Sampling"(w2011) -> ()
            n936 = local write "DAQ Config"(w2008) -> ()
            n937 = local write "AO Channels"(w2013) -> ()
            n938 = local write "Aux Channel"(w2007) -> ()
            n939 = local write "Cal Info"(w2016) -> ()
          }
          frame Error {
            # "If error, file might not exist. Try to write it."
            n940 = call <vilib>:"Clear Errors.vi"("error in (no error)"=w2020) -> ("error out"=w2019:errorcluster)  [unwired: 5 in, 1 out]
          }
        }
        n941 = Bundle By Name(cluster=w1996, "Lockin"=w1995) -> (w1994:T41)
        n942 = call <vilib>:"Add State(s) to Queue__jki_lib_state_machine.vi"("State(s) in Front (\"\")"=w1993, "State(s) in (\"\")"=w2005) -> ("States Out"=w2006:string)  [unwired: 13 in]
      }
      frame "---------Command----------" {
        n943 = call <vilib>:"Add State(s) to Queue__jki_lib_state_machine.vi"("State(s) in (\"\")"=w2026) -> ("States Out"=w2025:string)  [unwired: 14 in]
      }
      frame "Command: Handle Command" {
        n944 = Unbundle By Name(w2029) -> ("Lockin"=w2037:refnum<class "Instrument.Lockin.lvclass">, "Message.Command"=w2035:string, "Message.Data"=w2034:variant, "Message.ID"=w2027:string)
        n945 = call-dynamic "Handle Command.vi"("error in (no error)"=w2031, "Data"=w2034, "Command"=w2035, "Instrument.Lockin"=w2037) -> ("error out"=w2030:errorcluster, "Processed Data"=w2033:variant, "Command"=w2032:string, "Instrument.Lockin out"=w2036:refnum<class "Instrument.Lockin.lvclass">)  [unwired: 4 in]
        n946 = Bundle By Name(cluster=w2029, "Lockin"=w2036, "Message.Command"=w2032, "Message.Data"=w2033, "Message.ID"=w2027) -> (w2028:T41)
        n947 = call <vilib>:"Add State(s) to Queue__jki_lib_state_machine.vi"("State(s) in (\"\")"=w2040) -> ("States Out"=w2039:string)  [unwired: 14 in]
      }
      frame "Command: COMMANDS NOT HANDLED" {
        n948 = call <vilib>:"Add State(s) to Queue__jki_lib_state_machine.vi"("State(s) in (\"\")"=w2045) -> ("States Out"=w2044:string)  [unwired: 14 in]
      }
      frame "Command: getRefreshTime" {
        # "#todo\neliminate method?"
        # "#todo\nput on class wire"
        # "Triggers User Event to update front panel\nand put data onto class wire"
        n949 = Unbundle By Name(w2050) -> ("Message"=w2048:T38)
        n950 = local read "Refresh time (ms)"() -> (w2049:u32)
        n951 = To Variant(anything=w2049) -> (Variant=w2051:variant)
        n952 = Bundle By Name(cluster=w2048, "Data"=w2051) -> (w2047:T38)
        n953 = Bundle By Name(cluster=w2050, "HandledMessage"=w2047) -> (w2046:T41)
        n954 = call <vilib>:"Add State(s) to Queue__jki_lib_state_machine.vi"("State(s) in (\"\")"=w2055) -> ("States Out"=w2054:string)  [unwired: 14 in]
      }
      frame "Command: setAUX" {
        # "Convert Data from Message\nto appropriate data type"
        # "Triggers User Event to update front panel\nand put data onto class wire"
        n955 = Unbundle By Name(w2066) -> ("Message"=w2067:T38, "Message.Data"=w2060:variant)  [unwired: 1 out]
        n956 = Variant To Data(error in=w2056, type="", Variant=w2060) -> (data=w2061:string, error out=w2063:errorcluster)
        n957 = call "From JSON Text.vim"("Data Type and Default Value"=T32 {"AO Channel"=0, "AUX (V)"=0.0} ("setAUX"), "error in (no error)"=w2063, "JSON"=w2061) -> ("error out"=w2057:errorcluster, "Data out"=w2058:T32)  [unwired: 7 in]
        n958 = Unbundle By Name(w2058) -> ("AUX (V)"=w2065:dbl)  [unwired: 1 out]
        n959 = local write "Voltage Output (V)"(w2065) -> ()
        n960 = Bundle By Name(cluster=w2067, "Data"=w2065) -> (w2064:T38)
        n961 = Bundle By Name(cluster=w2066, "HandledMessage"=w2064) -> (w2068:T41)
        n962 = call <vilib>:"Add State(s) to Queue__jki_lib_state_machine.vi"("State(s) in Front (\"\")"="AUX: Set AUX" ("State(s) in Front (\"\")"), "State(s) in (\"\")"=w2072) -> ("States Out"=w2071:string)  [unwired: 13 in]
      }
      frame "Command: setOffset" {
        # "Convert Data from Message\nto appropriate data type"
        # "Triggers User Event to update front panel\nand put data onto class wire"
        n963 = Unbundle By Name(w2082) -> ("Message"=w2081:T38, "Message.Data"=w2077:variant)  [unwired: 1 out]
        n964 = Variant To Data(error in=w2076, type="" ("String"), Variant=w2077) -> (data=w2078:string, error out=w2080:errorcluster)
        n965 = call "From JSON Text.vim"("Data Type and Default Value"=Offset_Mode--Enum."Remove" ("Offset Mode"), "error in (no error)"=w2080, "JSON"=w2078) -> ("error out"=w2074:errorcluster, "Data out"=w2073:T34)  [unwired: 7 in]
        n966 = case shown="\"Remove\"" w2073 {
          tunnel: ["Lockin SMO: Measure Offset" ("State(s) in Front (\"\")") "Lockin SMO: Remove Offset" ("State(s) in Front (\"\")")] -> w2084
          frame "Measure", Default {
          }
          frame "Remove" {
          }
        }
        n967 = Bundle By Name(cluster=w2081, "Data"=w2073) -> (w2085:T38)
        n968 = Bundle By Name(cluster=w2082, "HandledMessage"=w2085) -> (w2083:T41)
        n969 = call <vilib>:"Add State(s) to Queue__jki_lib_state_machine.vi"("State(s) in Front (\"\")"=w2084, "State(s) in (\"\")"=w2088) -> ("States Out"=w2087:string)  [unwired: 13 in]
      }
      frame "---------- Notes ----------" {
        n970 = call <vilib>:"Add State(s) to Queue__jki_lib_state_machine.vi"("State(s) in (\"\")"=w2095) -> ("States Out"=w2094:string)  [unwired: 14 in]
      }
      frame "Notes: Controls" {
        n971 = call <vilib>:"Add State(s) to Queue__jki_lib_state_machine.vi"("State(s) in (\"\")"=w2100) -> ("States Out"=w2099:string)  [unwired: 14 in]
      }
      frame "Notes: Notes" {
        # "calculate RMS, Noise bandwidth, etc"
        # "Go to \"4461: SETUP\" if Reset, remote mode,\nor IV/continuous mode buttons are pushed"
        # "Multichannel Lockin v2016/06/02 SW TIMED SINGLE POINT\nREF:\nhttp://www.ni.com/white-paper/3215/en/ Example 9"
        # "TO DO:\n- intelligent decimate to dt setpoint\ncalculate RMS, Noise bandwidth, etc"
        n972 = disable-structure shown="Enabled" {
          frame Disabled {
            n973 = call <vilib>:"Open Config Data.vi"() -> ()  [unwired: 9 in, 3 out]
          }
          frame Enabled {
            # "JKI State Machine™\nhttp://jkisoft.com/state-machine/\nCopyright (C) 2005-2008, JKI <info@jkisoft.com>\nALL RIGHTS RESERVED"
            # "State Syntax:\nStateCategory: State >> Argument\nLine Terminator: Line feed\nExample:\nUI: Help >> About\n\nWhere \"UI\" is the state category\nWhere \"Help\" is the state\nWhere \"About\" is the argument\nOther Examples:\nApp Data: Initialize\nUI: Initialize\nHelp >> About\n\nCommenting:\nTo add a comment use \"//\" or \"#\" and all text to the right will be ignored\n\nCommenting Example:\nUI: Initialize // This initializes the UI\n# This whole line is a comment\n// Another comment line"
          }
        }
        n974 = call <vilib>:"Add State(s) to Queue__jki_lib_state_machine.vi"("State(s) in (\"\")"=w2105) -> ("States Out"=w2104:string)  [unwired: 14 in]
      }
    }
    n975 = call <userlib>:"State History.vi"("Current State"=w8) -> ("History"=→"State History":string)  [unwired: 6 in]
  }
  n976 = disable-structure shown="Disabled" {
    frame Disabled {
      n977 = Variant To Data(type="") -> (data=w2106:string, error out=w2108:errorcluster)  [unwired: 2 in]
      n978 = call "From JSON Text.vim"("error in (no error)"=w2108, "JSON"=w2106) -> ()  [unwired: 8 in, 2 out]
    }
    frame Enabled {
    }
  }
